vi "NLEISView_v15.vi"() -> ()   [LabVIEW 2018]
doc: "This example shows the Standard Function output mode. \n\nIt also shows some of the parameters which can be changed on the fly."
uses:
  <vilib>/Analysis/baseanly.llb/Mean (DBL).vi
  <vilib>/gmath/NumericalOptimization/Nonlinear Curve Fit TRDL bound.vi
  <vilib>/Analysis/polynomials.llb/Scalar Polynomial Evaluation (DBL).vi
  <vilib>/gmath/NI_Gmath.lvlib
  <vilib>/Analysis/NI_AALPro.lvlib
  <vilib>/Analysis/NI_AALBase.lvlib
panel:
  out "Number of Amps erased":dbl[][](array[numeric]) caption="Mag   Re     Im     Mag   Re     Im    Mag   Re     Im   Mag   Re     Im   Mag   Re     Im\n         V1                 V2                 V3                 V4                V5"
  in  "?":T1(tab)
  in  "Voltage Signal Amplification":string(combo)="1"
  in  "Current Signal Amplification":string(combo)="1"
  in  "Perturbation Method":string(combo)="1"
  in  "IR Setting":enum32{"Single IR", "Multiple IR"}(tab)
  in  "Internal Resistor":string(combo)
  in  "Low Freq (Hz) \nFor IR Switch":dbl
  in  "IR High Freq":string(combo)
  in  "IR Mid Freq":string(combo)
  in  "IR Low Freq":string(combo)
  in  "High Freq  (Hz)\nFor IR Switch":dbl
  in  "Highest Amplitude #":dbl=20.0 format="%#.3f"
  in  "Lowest Amplitude #":dbl=1.0 caption="Amps" format="%#.3f"
  in  "Frequencies High To Low":bool=TRUE
  in  "Highest Freq #":dbl=1.0 format="%#.3f"
  in  "Lowest Freq #":dbl=1.0 caption="Freqs" format="%#.3f"
  in  "Append To File?":bool=TRUE
  in  "Write NLEIS VIEW to File?":bool=TRUE
  in  "Harmonic Nondimensionalization":enum32{"Dimensional", "NonDimensional"}(tab)
  in  "Temperature":dbl=1.0
  out "Vstar":dbl
  in  "Temperature 2":dbl=1.0
  in  "Istar (Amps)":dbl=1.0 format="%.8f"
  in  "Rchem":dbl=1.0
  out "Vstar 2":dbl
  in  "Istar Entered":bool
  in  "Write SUBVI Array?":bool
  in  "File Path Write SUBVI Array":path=path "C:/new3.txt"
  in  "Fitting Parameters":T2(tab)
  in  "LS Program":bool
  in  "Tolerance (vk)":dbl=0.0001
  in  "Fitting Method (vk)":string(combo)="0"
  in  "Gaussian Window\nParameter (B)":dbl=20.0
  in  "Error Noise Filter":dbl=1.5
  in  "Sigma Noise Filter":dbl=1.5
  in  "Lookup Table":bool
  in  "Baseline":bool
  in  "Tolerance (a)":dbl=1e-15
  in  "Max Iterations (a)":i32=1000
  in  "% of V11":dbl=10.0
  in  "% of V22/V33":dbl=50.0
  in  "Fitting Method (a)":string(combo)="0"
  in  "V15 & V35":bool
  in  "V24 Fitting":bool
  in  "V13 Fitting":bool
  in  "Weighting":bool caption="Use\n \n \nDon't Use"
  in  "V1/Alpha Amp to Noise Ratio":dbl=10.0
  in  "V2 Amp to Noise Ratio":dbl=5.0
  in  "V3 Amp to Noise Ratio":dbl=3.0
  in  "V4 Amp to Noise Ratio":dbl=3.0
  in  "V5 Amp to Noise Ratio":dbl=3.0
  out "Graphs Updated":bool
  in  "Alpha Fitting Filters":enum32{"1 Set of Param.", "3 Sets of Param."}(tab)=enum."3 Sets of Param."
  in  "Amps Erase":sgl
  in  "MSE Multiplier":dbl=1.0
  in  "V1 Amps Erase":sgl
  in  "V2 Amps Erase":sgl
  in  "V3 Amps Erase":sgl
  in  "V1 MSE Multiplier":dbl=100.0
  in  "V2 MSE Multiplier":dbl=100.0
  in  "V3 MSE Multiplier":dbl=100.0
  out "Number of Amps used":dbl[](array[numeric])
  in  "stop":bool
  in  "File Path Write NLEISVIEW Data":path=path "C:/Users/Giang/Desktop/NLEIS_test/nleis-test6/diode"
  out "Frequency":dbl=25.298234939575195 format="%#_10f"
  in  "Front Panel Tab Control Icon - Do not delete":enum32{"V vs. Alpha", "Vn vs. Alpha^n"}(tab)=enum."Vn vs. Alpha^n"
  out "V2 Re":cluster{cluster{dbl, "P(a)":dbl}[]}[](graph)
  out "V2 Mag":cluster{cluster{dbl, "P(a)":dbl}[]}[](graph)
  out "V5 Re":T3(graph)
  out "V2 Im":cluster{cluster{dbl, "P(a)":dbl}[]}[](graph)
  out "V3 Mag":cluster{cluster{dbl, "P(a)":dbl}[]}[](graph)
  out "V3 Re":cluster{cluster{dbl, "P(a)":dbl}[]}[](graph)
  out "V3 Im":cluster{cluster{dbl, "P(a)":dbl}[]}[](graph)
  out "V1 Im":cluster{cluster{dbl, "P(a)":dbl}[]}[](graph)
  out "V5 Mag":T3(graph)
  out "V4 Mag":T3(graph)
  out "V4 Re":T3(graph)
  out "V4 Im":cluster{cluster{dbl, "P(a)":dbl}[]}[](graph)
  out "V5 Im":T3(graph)
  out "V1 Mag":cluster{cluster{dbl, dbl}[]}[](graph)=[{[{0.0, 0.0}, {0.11592337776297197, 0.03304485781030145}, {0.17490677190679904, 0.04955962038935185}, {0.3482190445344051, 0.09902951519088735}, {0.5812437888783601, 0.16517748864964857}, {0.8729957405472275, 0.2483952099845861}, {0.9301513780701758, 0.2646275668898653}, {0.9887433954568534, 0.2813401317697576}, {1.0477077074181451, 0.29781838994307164}, {1.1050180353393082, 0.314210624473721}, {1.3370638463516271, 0.38017329335049976}, {1.3957495994333853, 0.39653508030752266}, {1.5127853787825267, 0.429714440189949}, {1.5708225495208372, 0.4461228771616594}]}, {[{0.0, 0.0}, {0.11592337776297197, 0.03295810708345434}, {0.17490677190679904, 0.04972841122082627}, {0.3482190445344051, 0.0990110384083542}, {0.5812437888783601, 0.16529212065005314}, {0.8729957405472275, 0.24829143514258742}, {0.9301513780701758, 0.2645473352700113}, {0.9887433954568534, 0.2812079100684176}, {1.0477077074181451, 0.2979689236770735}, {1.1050180353393082, 0.31425292299017493}, {1.3370638463516271, 0.3800753565931724}, {1.3957495994333853, 0.39668139114349815}, {1.5127853787825267, 0.4297271370666853}, {1.5708225495208372, 0.44607154435403673}]}]
  out "V1 Re":cluster{cluster{dbl, "P(a)":dbl}[]}[](graph)
  out "V4 Im vs. a^4":cluster{cluster{dbl, "P(a)":dbl}[]}[](graph)
  out "V5 Im vs. a^5":cluster{cluster{dbl, "P(a)":dbl}[]}[](graph)
  out "V3 Mag vs. a^3":cluster{cluster{dbl, "P(a)":dbl}[]}[](graph)
  out "V4 Mag vs. a^4":cluster{cluster{dbl, "P(a)":dbl}[]}[](graph)
  out "V5 Mag vs. a^5":cluster{cluster{dbl, "P(a)":dbl}[]}[](graph)
  out "V2 Im vs. a^2":cluster{cluster{dbl, "P(a)":dbl}[]}[](graph)
  out "V2 Re vs. a^2":cluster{cluster{dbl, "P(a)":dbl}[]}[](graph)
  out "V2 Mag vs. a^2":cluster{cluster{dbl, "P(a)":dbl}[]}[](graph)
  out "V3 Im vs. a^3":cluster{cluster{dbl, "P(a)":dbl}[]}[](graph)
  out "V5 Re vs. a^5":cluster{cluster{dbl, "P(a)":dbl}[]}[](graph)
  out "V4 Re vs. a^4":cluster{cluster{dbl, "P(a)":dbl}[]}[](graph)
  out "V3 Re vs. a^3":cluster{cluster{dbl, "P(a)":dbl}[]}[](graph)
  out "V1 Im vs. a^1":cluster{cluster{dbl, "P(a)":dbl}[]}[](graph)
  out "V1 Mag vs. a^1":cluster{cluster{dbl, dbl}[]}[](graph)=[{[{0.0, 0.0}, {0.11592337776297197, 0.03304485781030145}, {0.17490677190679904, 0.04955962038935185}, {0.3482190445344051, 0.09902951519088735}, {0.5812437888783601, 0.16517748864964857}, {0.8729957405472275, 0.2483952099845861}, {0.9301513780701758, 0.2646275668898653}, {0.9887433954568534, 0.2813401317697576}, {1.0477077074181451, 0.29781838994307164}, {1.1050180353393082, 0.314210624473721}, {1.3370638463516271, 0.38017329335049976}, {1.3957495994333853, 0.39653508030752266}, {1.5127853787825267, 0.429714440189949}, {1.5708225495208372, 0.4461228771616594}]}, {[{0.0, 0.0}, {0.11592337776297197, 0.03295810708345434}, {0.17490677190679904, 0.04972841122082627}, {0.3482190445344051, 0.0990110384083542}, {0.5812437888783601, 0.16529212065005314}, {0.8729957405472275, 0.24829143514258742}, {0.9301513780701758, 0.2645473352700113}, {0.9887433954568534, 0.2812079100684176}, {1.0477077074181451, 0.2979689236770735}, {1.1050180353393082, 0.31425292299017493}, {1.3370638463516271, 0.3800753565931724}, {1.3957495994333853, 0.39668139114349815}, {1.5127853787825267, 0.4297271370666853}, {1.5708225495208372, 0.44607154435403673}]}]
  out "V1 Re vs. a^1":cluster{cluster{dbl, "P(a)":dbl}[]}[](graph)
  in  "File Path Read NLEISRUN Data":path=path "C:/Users/Giang/Desktop/NLEIS_test/test6/diode"
  # "MSE Multiplier\n \nAmps Erase\n \nSigma/MSE Noise Filters"
  # "Amplitudes"
  # "Frequencies"
  # "Higher Harmonic\nBounds"
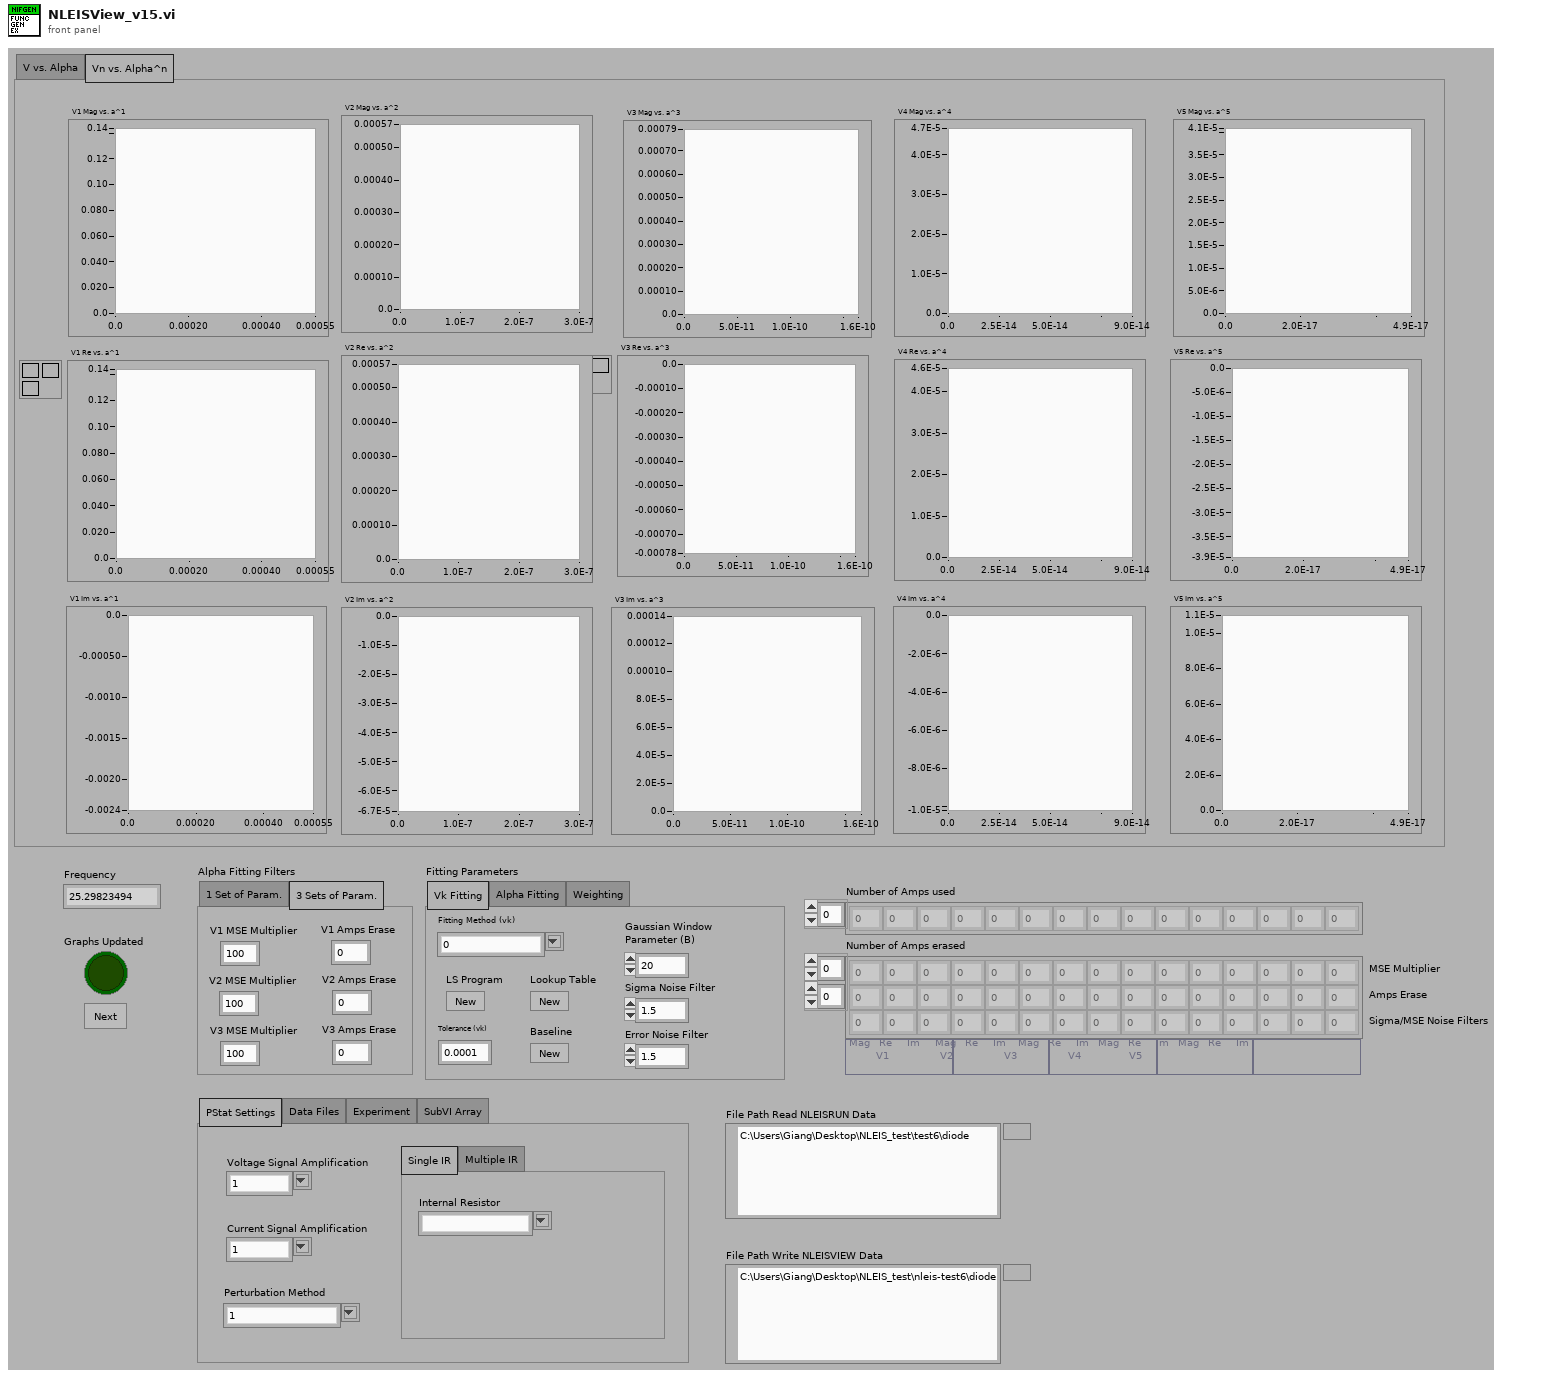
[diagram p1: front panel]
types:
  T1 = enum32{"PStat Settings", "Data Files", "Experiment", "SubVI Array"}
  T2 = enum32{"Vk Fitting", "Alpha Fitting", "Weighting"}
  T3 = cluster{cluster{"new element/subarray":dbl, "P(a)":dbl}[]}[]
  T4 = cluster{"Max Iterations (a)":i32, "Tolerance (a)":dbl}
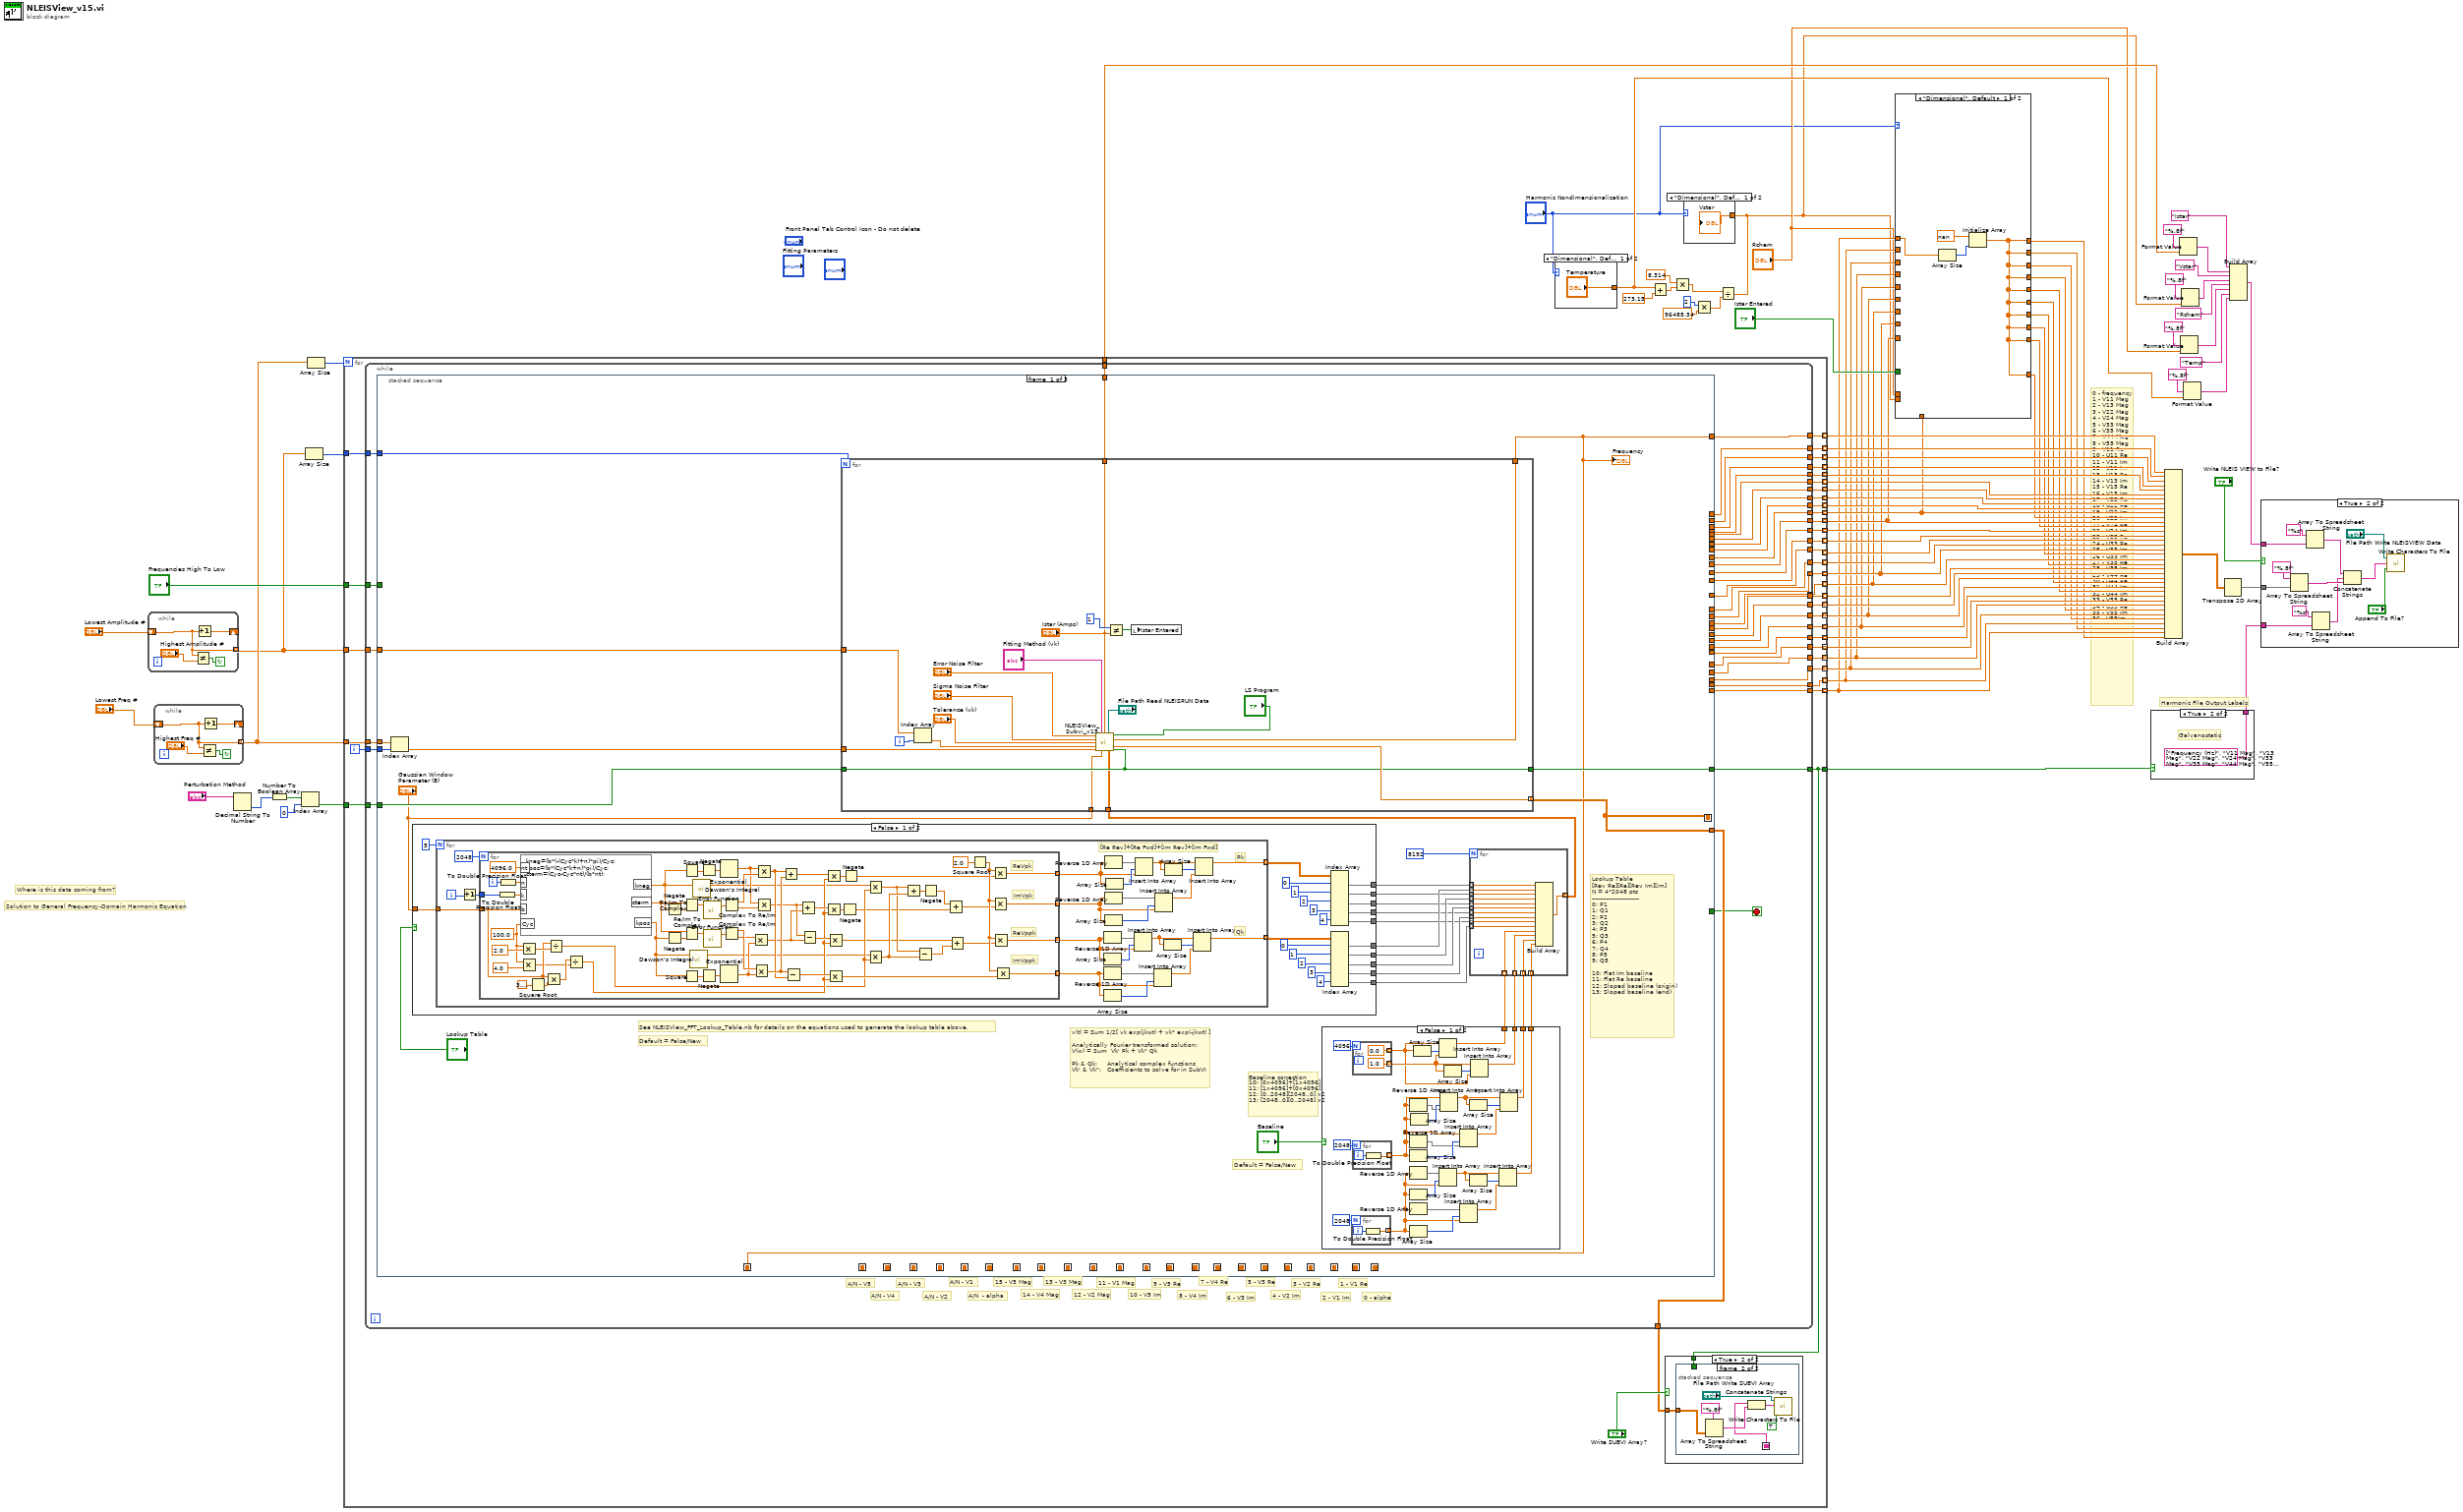
[diagram p0: block diagram]
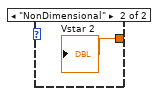
[diagram p2: hidden frame]
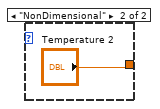
[diagram p3: hidden frame]
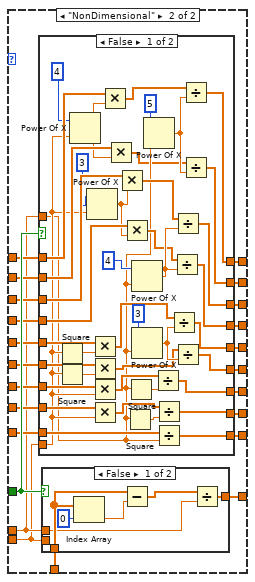
[diagram p4: hidden frame]
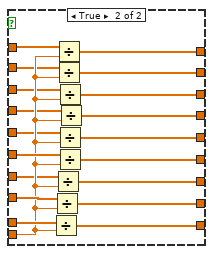
[diagram p5: hidden frame]
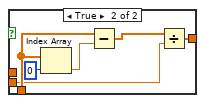
[diagram p6: hidden frame]
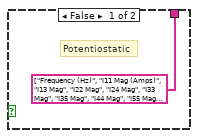
[diagram p8: hidden frame]
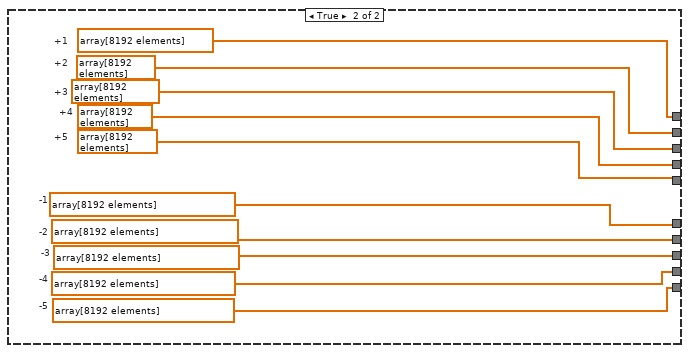
[diagram p9: hidden frame]
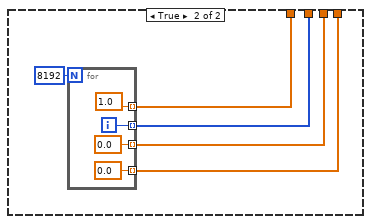
[diagram p10: hidden frame]
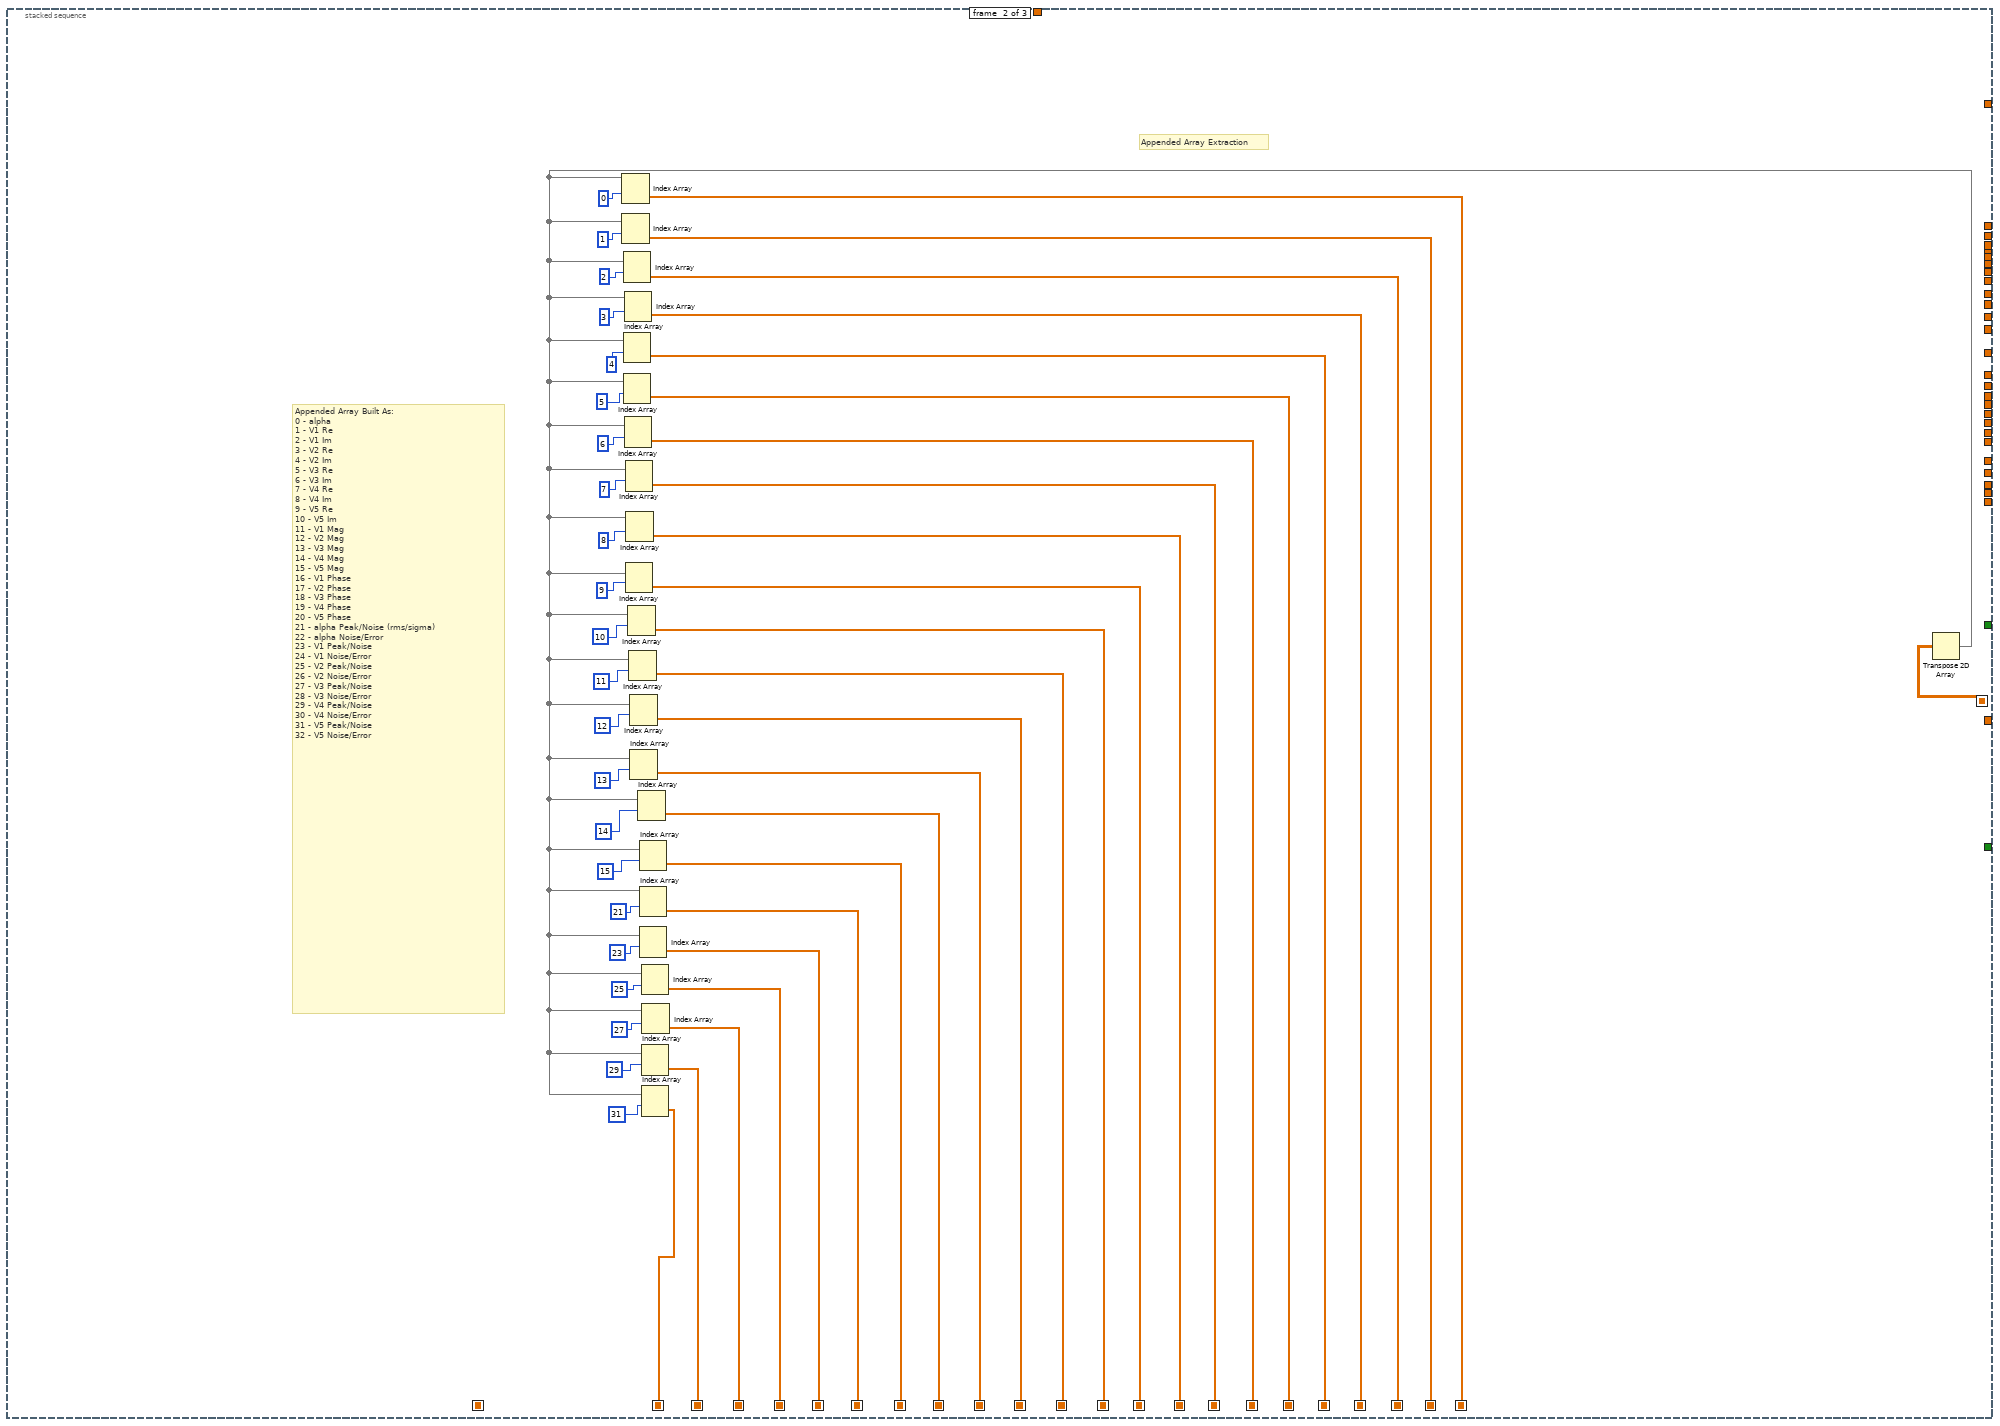
[diagram p11: hidden frame]
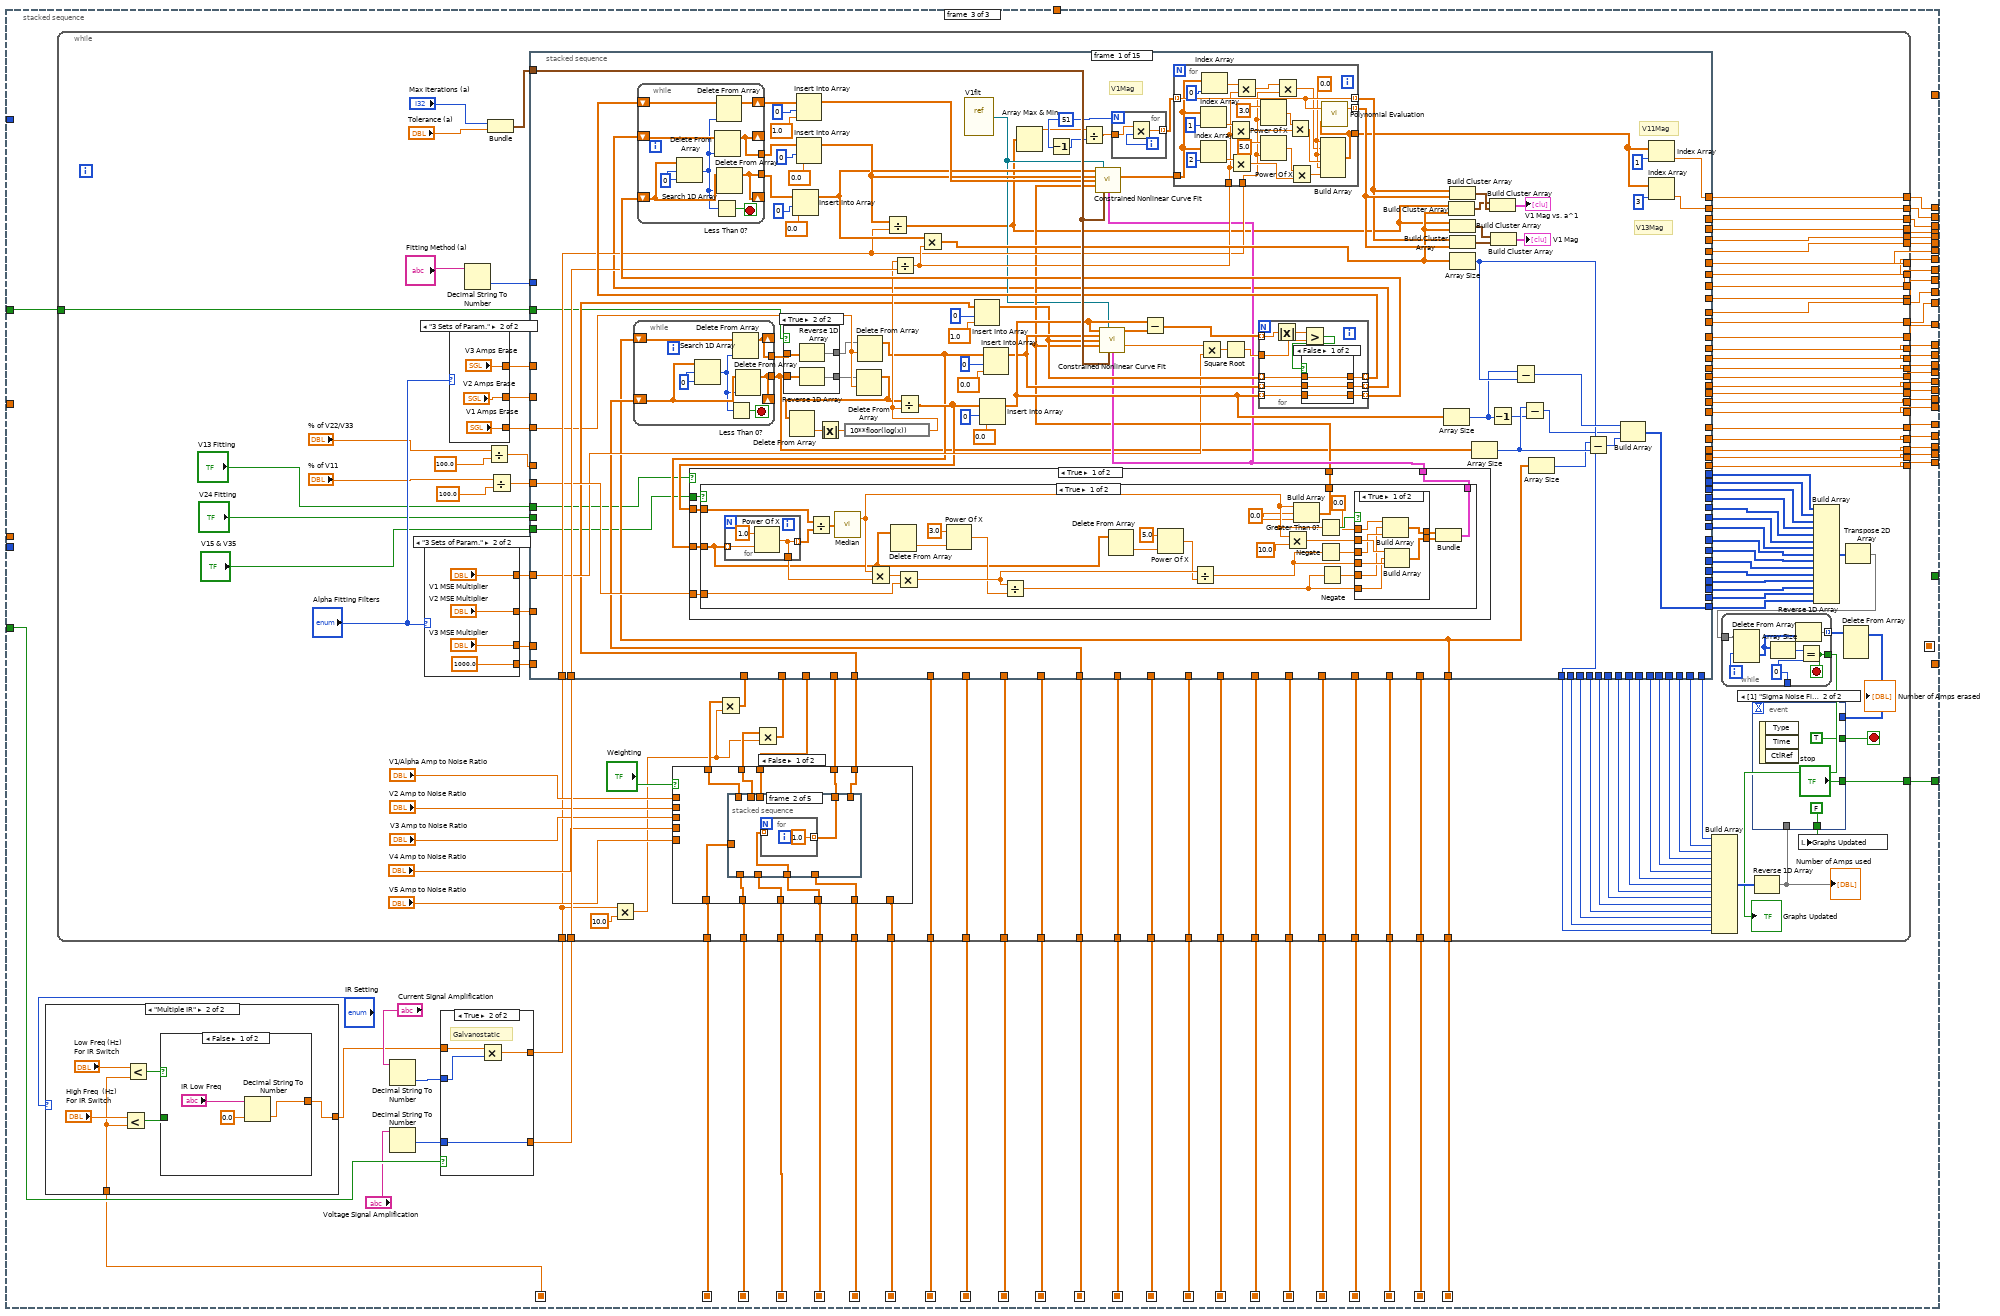
[diagram p12: hidden frame]
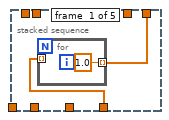
[diagram p13: hidden frame]
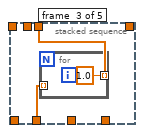
[diagram p14: hidden frame]
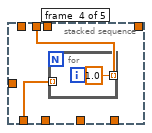
[diagram p15: hidden frame]
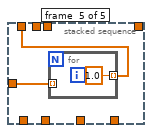
[diagram p16: hidden frame]
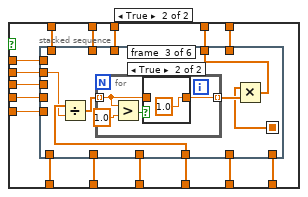
[diagram p17: hidden frame]
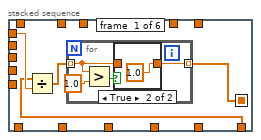
[diagram p18: hidden frame]
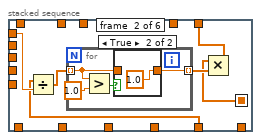
[diagram p20: hidden frame]
diagram:
  # "Where is this data coming from?"
  # "Solution to General Frequency-Domain Harmonic Equation"
  # "0 - frequency\n1 - V11 Mag\n2 - V13 Mag\n3 - V22 Mag\n4 - V24 Mag\n5 - V33 Mag\n6 - V35 Mag\n7 - V44 Mag\n8 - V55 Mag\n9 - V11 Re\n10 - U11 Re\n11 - V11 Im\n12 - U11 Im\n13 - V13 Re\n14 - V13 Im\n15 - V15 Re\n16 - V15 Im\n17 - V22 Re\n18 - U22 Re\n19 - V22 Im\n20 - U22 Im\n21 - V24 Re\n22 - V24 Im\n23 - V33 Re\n24 - U33 Re\n25 - V33 Im\n26 - U33 Im\n27 - V35 Re\n28 - V35 Im\n29 - V44 Re\n30 - U44 Re\n31 - V44 Im\n32 - U44 Im\n33 - V55 Re\n34 - U55 Re\n35 - V55 Im\n36 - U55Im"
  # "Harmonic File Output Labels"
  n1 = while {
    shift-right: [w82] -> _
    shift-left: "Lowest Amplitude #" -> [w83]
    tunnel: [w83] -> w29 mode=indexing
    stop <- w84 continue-if-true
    n2 = Not Equal?(x=w83, y="Highest Amplitude #") -> (x != y?=w84:bool)
    n3 = Increment(x=w83) -> (x+1=w82:dbl)
  }
  n4 = while {
    shift-right: [w86] -> _
    shift-left: "Lowest Freq #" -> [w87]
    tunnel: [w87] -> w30 mode=indexing
    stop <- w88 continue-if-true
    n5 = Not Equal?(x=w87, y="Highest Freq #") -> (x != y?=w88:bool)
    n6 = Increment(x=w87) -> (x+1=w86:dbl)
  }
  n7 = Decimal String To Number(string="Perturbation Method") -> (number=w78:i32)  [unwired: 2 in, 1 out]
  n8 = Number To Boolean Array(number=w78) -> (Boolean array=w80:bool[])
  n9 = Index Array(array=w80, index=0) -> (element=w76:bool)
  n10 = Array Size(array=w29) -> (size(s)=w28:i32)
  n11 = Array Size(array=w30) -> (size(s)=w31:i32)
  n12 = for {
    N: w31 -> [_]
    tunnel: [w124] -> w72 mode=indexing
    tunnel: [w123] -> w71 mode=indexing
    tunnel: [w122] -> w70 mode=indexing
    tunnel: [w121] -> w69 mode=indexing
    tunnel: [w120] -> w68 mode=indexing
    tunnel: [w119] -> w67 mode=indexing
    tunnel: [w118] -> w66 mode=indexing
    tunnel: [w117] -> w65 mode=indexing
    tunnel: [w89] -> w51 mode=indexing
    tunnel: [w116] -> w49 mode=indexing
    tunnel: [w115] -> w64 mode=indexing
    tunnel: [w114] -> w63 mode=indexing
    tunnel: [w113] -> w48 mode=indexing
    tunnel: [w112] -> w47 mode=indexing
    tunnel: [w111] -> w61 mode=indexing
    tunnel: [w110] -> w52 mode=indexing
    tunnel: [w109] -> w46 mode=indexing
    tunnel: [w108] -> w45 mode=indexing
    tunnel: [w107] -> w60 mode=indexing
    tunnel: [w106] -> w59 mode=indexing
    tunnel: [w105] -> w44 mode=indexing
    tunnel: [w104] -> w43 mode=indexing
    tunnel: [w103] -> w42 mode=indexing
    tunnel: [w102] -> w41 mode=indexing
    tunnel: [w101] -> w55 mode=indexing
    tunnel: w30 -> [w100]
    tunnel: w76 -> [w99]
    tunnel: w29 -> [w98]
    tunnel: [w90] -> w75
    tunnel: [w97] -> w62 mode=indexing
    tunnel: [w96] -> w53 mode=indexing
    tunnel: "Frequencies High To Low" -> [w95]
    tunnel: w28 -> [w94]
    tunnel: [w93] -> w18
    i -> [w125]
    n13 = while {
      tunnel: w125 -> [w162]
      tunnel: [w161] -> w124
      tunnel: [w160] -> w123
      tunnel: [w159] -> w122
      tunnel: [w158] -> w121
      tunnel: [w157] -> w120
      tunnel: [w156] -> w119
      tunnel: [w155] -> w118
      tunnel: [w154] -> w117
      tunnel: [w153] -> w116
      tunnel: [w152] -> w115
      tunnel: [w151] -> w114
      tunnel: [w150] -> w113
      tunnel: [w149] -> w112
      tunnel: [w148] -> w111
      tunnel: [w147] -> w110
      tunnel: [w146] -> w109
      tunnel: [w145] -> w108
      tunnel: [w144] -> w107
      tunnel: [w143] -> w106
      tunnel: [w142] -> w105
      tunnel: [w141] -> w104
      tunnel: [w140] -> w103
      tunnel: [w139] -> w102
      tunnel: [w138] -> w101
      tunnel: w100 -> [w137]
      tunnel: w99 -> [w136]
      tunnel: w98 -> [w135]
      tunnel: [w134] -> w97
      tunnel: [w133] -> w96
      tunnel: w95 -> [w132]
      tunnel: w94 -> [w131]
      tunnel: [w130] -> w93
      tunnel: [w129] -> w91
      tunnel: [w128] -> w90
      tunnel: [w127] -> w89
      stop <- w126 stop-if-true
      # "A/N - V5"
      # "A/N - V4"
      # "A/N - V3"
      # "A/N - V2"
      # "A/N - V1"
      # "A/N  - alpha"
      # "15 - V5 Mag"
      # "14 - V4 Mag"
      # "13 - V3 Mag"
      # "12 - V2 Mag"
      # "11 - V1 Mag"
      # "10 - V5 Im"
      # "9 - V5 Re"
      # "8 - V4 Im"
      # "7 - V4 Re"
      # "6 - V3 Im"
      # "5 - V3 Re"
      # "4 - V2 Im"
      # "3 - V2 Re"
      # "2 - V1 Im"
      # "1 - V1 Re"
      # "0 - alpha"
      n14 = stacked-sequence {
        seq-local: [w189 _ _] -> [_ w434 _]
        seq-local: [_ w404 _] -> [_ _ w472]
        seq-local: [_ w402 _] -> [_ _ w471]
        seq-local: [_ w401 _] -> [_ _ w470]
        seq-local: [_ w399 _] -> [_ _ w469]
        seq-local: [_ w398 _] -> [_ _ w468]
        seq-local: [_ w396 _] -> [_ _ w467]
        seq-local: [_ w395 _] -> [_ _ w466]
        seq-local: [_ w417 _] -> [_ _ w465]
        seq-local: [_ w416 _] -> [_ _ w464]
        seq-local: [_ w415 _] -> [_ _ w463]
        seq-local: [_ w414 _] -> [_ _ w462]
        seq-local: [_ w403 _] -> [_ _ w461]
        seq-local: [_ w400 _] -> [_ _ w460]
        seq-local: [_ w397 _] -> [_ _ w459]
        seq-local: [_ w413 _] -> [_ _ w458]
        seq-local: [_ w412 _] -> [_ _ w457]
        seq-local: [w182 _ _] -> [_ _ w444]
        seq-local: [_ w394 _] -> [_ _ w441]
        seq-local: [_ w393 _] -> [_ _ w440]
        seq-local: [_ w392 _] -> [_ _ w439]
        seq-local: [_ w391 _] -> [_ _ w438]
        seq-local: [_ w390 _] -> [_ _ w437]
        seq-local: [_ w389 _] -> [_ _ w436]
        tunnel: w162 -> [w191 _ _]
        tunnel: [_ _ w494] -> w127
        tunnel: [_ _ w493] -> w153
        tunnel: [_ _ w492] -> w152
        tunnel: [_ _ w491] -> w151
        tunnel: [_ _ w490] -> w134
        tunnel: [_ _ w489] -> w133
        tunnel: [_ _ w456] -> w150
        tunnel: [_ _ w488] -> w149
        tunnel: [_ _ w455] -> w148
        tunnel: [_ _ w487] -> w147
        tunnel: [_ _ w452] -> w146
        tunnel: [_ _ w450] -> w145
        tunnel: [_ _ w451] -> w144
        tunnel: [_ _ w449] -> w143
        tunnel: [_ _ w486] -> w142
        tunnel: [_ _ w485] -> w141
        tunnel: [_ _ w484] -> w140
        tunnel: [_ _ w483] -> w139
        tunnel: [_ _ w482] -> w160
        tunnel: [w182 _ _] -> w161
        tunnel: [_ _ w481] -> w159
        tunnel: [_ _ w480] -> w158
        tunnel: [_ _ w479] -> w157
        tunnel: [_ _ w454] -> w156
        tunnel: [_ _ w453] -> w155
        tunnel: [_ _ w448] -> w154
        tunnel: [_ _ w447] -> w138
        tunnel: w137 -> [w190 _ _]
        tunnel: [w189 _ _] -> w129
        tunnel: w136 -> [w188 _ w478]
        tunnel: w135 -> [w187 _ _]
        tunnel: [w186 _ _] -> w128
        tunnel: w132 -> [_ _ w446]
        tunnel: w131 -> [w185 _ _]
        tunnel: [w184 _ _] -> w130
        tunnel: [_ _ w435] -> w126
        frame #0 {
          # "Baseline correction\n10: [0x4096]+[1x4096]\n11: [1x4096]+[0x4096]\n12: [0..2048][2048..0] x2\n13: [2048..0][0..2048] x2"
          # "v(t) = Sum 1/2[ vk exp(jkwt) + vk* exp(-jkwt) ]\n\nAnalytically Fourier transformed solution:\nV(w) = Sum  Vk' Pk + Vk\" Qk\n\nPk & Qk:     Analytical complex functions\nVk' & Vk\":   Coefficients to solve for in SubVI"
          # "Lookup Table\n[Rev Re][Re][Rev Im][Im]\nN = 4*2048 pts\n------------------------\n0: P1\n1: Q1\n2: P2\n3: Q2\n4: P3\n5: Q3\n6: P4\n7: Q4\n8: P5\n9: Q5\n\n10: Flat Im baseline\n11: Flat Re baseline\n12: Sloped baseline (origin)\n13: Sloped baseline (end)"
          # "Default = False/New"
          # "Default = False/New"
          # "See NLEISView_FFT_Lookup_Table.nb for details on the equations used to generate the lookup table above."
          n15 = Index Array(array=w190, index=w191) -> (element=w183:dbl)
          n16 = case shown="False" "Lookup Table" {
            tunnel: [w213 w313] -> w180
            tunnel: [w212 w308] -> w179
            tunnel: [w211 w312] -> w178
            tunnel: [w210 w307] -> w177
            tunnel: [w209 w311] -> w176
            tunnel: [w208 w306] -> w175
            tunnel: [w207 w310] -> w174
            tunnel: [w206 w305] -> w173
            tunnel: [w205 w309] -> w172
            tunnel: [w204 w304] -> w171
            tunnel: "Gaussian Window\nParameter (B)" -> [w203 _]
            frame False {
              n17 = for {
                N: 5 -> [_]
                tunnel: w203 -> [w238]
                tunnel: [w219] -> w215 mode=indexing
                tunnel: [w218] -> w214 mode=indexing
                i -> [w237]
                # "[Re Rev]+[Re Fwd]+[Im Rev]+[Im Fwd]"
                # "Qk"
                # "Pk"
                n18 = Increment(x=w237) -> (x+1=w236:i32)
                n19 = for {
                  N: 2048 -> [_]
                  tunnel: w238 -> [w275]
                  tunnel: w236 -> [w300]
                  tunnel: [w293] -> w229 mode=indexing
                  tunnel: [w294] -> w228 mode=indexing
                  tunnel: [w295] -> w221 mode=indexing
                  tunnel: [w296] -> w220 mode=indexing
                  i -> [w303]
                  w278 = 100.0 ("element")
                  # "ImVppk"
                  # "ReVppk"
                  # "ImVpk"
                  # "ReVpk"
                  n20 = To Double Precision Float(number=w300) -> (double precision float=w299:dbl)
                  n21 = To Double Precision Float(number=w303) -> (double precision float=w301:dbl)
                  n22 = Multiply(x=w278, y=2.0 ("element")) -> (x*y=w279:dbl)
                  n23 = Multiply(x=w278, y=4.0 ("element")) -> (x*y=w272:dbl)
                  n24 = formula code="kneg=(b*(-(Cyc*k)+n)*pi)/Cyc;\nkpos=(b*(Cyc*k+n)*pi)/Cyc;\ncterm=(Cyc-Cyc*nt)/(b*nt);"("n"=w301, "Cyc"=w278, "b"=w275, "k"=w299, "nt"=4096.0 ("element")) -> ("kpos"=w264:dbl, "kneg"=w263:dbl, "cterm"=w285:dbl)
                  n25 = Square Root(x=3.141592653589793) -> (sqrt(x)=w274:dbl)
                  n26 = Multiply(x=w275, y=w274) -> (x*y=w273:dbl)
                  n27 = Divide(x=w275, y=w279) -> (x/y=w251:dbl)
                  n28 = Divide(x=w273, y=w272) -> (x/y=w256:dbl)
                  n29 = Negate(x=w263) -> (-x=w291:dbl)
                  n30 = Negate(x=w264) -> (-x=w284:dbl)
                  n31 = Square(x=w263) -> (x^2=w289:dbl)
                  n32 = Re/Im To Complex(1:w291, 2:w285) -> (0:w290:cdb)
                  n33 = Re/Im To Complex(1:w284, 2:w285) -> (0:w283:cdb)
                  n34 = Square(x=w264) -> (x^2=w282:dbl)
                  n35 = call <vilib>:"Dawson's Integral.vi"("x"=w264) -> ("daw(x)"=w250:dbl)  [unwired: 2 in]
                  n36 = call <vilib>:"Dawson's Integral.vi"("x"=w263) -> ("daw(x)"=w252:dbl)  [unwired: 2 in]
                  n37 = Negate(x=w289) -> (-x=w288:dbl)
                  n38 = Negate(x=w282) -> (-x=w281:dbl)
                  n39 = call <vilib>:"Error Function.vi"("x"=w290) -> ("erf(x)"=w292:dbl)  [unwired: 2 in]
                  n40 = call <vilib>:"Error Function.vi"("x"=w283) -> ("erf(x)"=w286:dbl)  [unwired: 2 in]
                  n41 = Exponential(1:w288) -> (0:w260:dbl)
                  n42 = Exponential(1:w281) -> (0:w257:dbl)
                  n43 = Complex To Re/Im(x + iy=w292) -> (x=w287:dbl, y=w261:dbl)
                  n44 = Complex To Re/Im(x + iy=w286) -> (x=w280:dbl, y=w258:dbl)
                  n45 = Multiply(x=w258, y=w257) -> (x*y=w253:dbl)
                  n46 = Multiply(x=w280, y=w257) -> (x*y=w267:dbl)
                  n47 = Multiply(x=w260, y=w287) -> (x*y=w266:dbl)
                  n48 = Multiply(x=w260, y=w261) -> (x*y=w254:dbl)
                  n49 = Add(x=w266, y=w267) -> (x+y=w271:dbl)
                  n50 = Subtract(x=w267, y=w266) -> (x-y=w268:dbl)
                  n51 = Add(x=w254, y=w253) -> (x+y=w262:dbl)
                  n52 = Subtract(x=w254, y=w253) -> (x-y=w259:dbl)
                  n53 = Multiply(x=w271, y=w256) -> (x*y=w270:dbl)
                  n54 = Multiply(x=w262, y=w256) -> (x*y=w255:dbl)
                  n55 = Multiply(x=w259, y=w256) -> (x*y=w243:dbl)
                  n56 = Multiply(x=w268, y=w256) -> (x*y=w265:dbl)
                  n57 = Negate(x=w255) -> (-x=w246:dbl)
                  n58 = Negate(x=w270) -> (-x=w269:dbl)
                  n59 = Multiply(x=w252, y=w251) -> (x*y=w248:dbl)
                  n60 = Multiply(x=w250, y=w251) -> (x*y=w249:dbl)
                  n61 = Add(x=w248, y=w249) -> (x+y=w247:dbl)
                  n62 = Subtract(x=w248, y=w249) -> (x-y=w244:dbl)
                  n63 = Negate(x=w247) -> (-x=w245:dbl)
                  n64 = Add(x=w245, y=w246) -> (x+y=w242:dbl)
                  n65 = Add(x=w243, y=w244) -> (x+y=w241:dbl)
                  n66 = Square Root(x=2.0 ("element")) -> (sqrt(x)=w297:dbl)
                  n67 = Multiply(x=w297, y=w269) -> (x*y=w293:dbl)
                  n68 = Multiply(x=w297, y=w242) -> (x*y=w294:dbl)
                  n69 = Multiply(x=w297, y=w241) -> (x*y=w295:dbl)
                  n70 = Multiply(x=w297, y=w265) -> (x*y=w296:dbl)
                }
                n71 = Reverse 1D Array(array=w221) -> (reversed array=w222:dbl[])
                n72 = Reverse 1D Array(array=w220) -> (reversed array=w216:dbl[])
                n73 = Array Size(array=w220) -> (size(s)=w223:i32)
                n74 = Array Size(array=w221) -> (size(s)=w224:i32)
                n75 = Reverse 1D Array(array=w229) -> (reversed array=w230:dbl[])
                n76 = Reverse 1D Array(array=w228) -> (reversed array=w217:dbl[])
                n77 = Array Size(array=w228) -> (size(s)=w231:i32)
                n78 = Array Size(array=w229) -> (size(s)=w232:i32)
                n79 = Insert Into Array(array=w222, index=w224, new element=w221) -> (w227:dbl[])
                n80 = Insert Into Array(array=w230, index=w232, new element=w229) -> (w235:dbl[])
                n81 = Insert Into Array(array=w216, index=w223, new element=w220) -> (w226:dbl[])
                n82 = Insert Into Array(array=w217, index=w231, new element=w228) -> (w234:dbl[])
                n83 = Array Size(array=w227) -> (size(s)=w225:i32)
                n84 = Array Size(array=w235) -> (size(s)=w233:i32)
                n85 = Insert Into Array(array=w227, index=w225, new element=w226) -> (w218:dbl[])
                n86 = Insert Into Array(array=w235, index=w233, new element=w234) -> (w219:dbl[])
              }
              n87 = Index Array(array=w215, index (row) #1=0, index (row) #2=1, index (row) #3=2, index (row) #4=3, index (row) #5=4) -> (element #1=w213:dbl[], element #2=w211:dbl[], element #3=w209:dbl[], element #4=w207:dbl[], element #5=w205:dbl[])  [unwired: 5 in]
              n88 = Index Array(array=w214, index (row) #1=0, index (row) #2=1, index (row) #3=2, index (row) #4=3, index (row) #5=4) -> (element #1=w212:dbl[], element #2=w210:dbl[], element #3=w208:dbl[], element #4=w206:dbl[], element #5=w204:dbl[])  [unwired: 5 in]
            }
            frame True {
              w304 = dbl[] array[8192 elements]  # -5
              w309 = dbl[] array[8192 elements]  # +5
              w305 = dbl[] array[8192 elements]  # -4
              w310 = dbl[] array[8192 elements]  # +4
              w306 = dbl[] array[8192 elements]  # -3
              w311 = dbl[] array[8192 elements]  # +3
              w307 = dbl[] array[8192 elements]  # -2
              w312 = dbl[] array[8192 elements]  # +2
              w308 = dbl[] array[8192 elements]  # -1
              w313 = dbl[] array[8192 elements]  # +1
            }
          }
          n89 = case shown="False" "Baseline" {
            tunnel: [w332 w347] -> w170
            tunnel: [w322 w348] -> w169
            tunnel: [w317 w350] -> w168
            tunnel: [w316 w349] -> w167
            frame False {
              n90 = for {
                N: 2048 -> [_]
                tunnel: [w345] -> w333 mode=indexing
                i -> [w346]
                n91 = To Double Precision Float(number=w346) -> (double precision float=w345:dbl)
              }
              n92 = for {
                N: 4096 -> [_]
                tunnel: [0.0 ("element")] -> w318 mode=indexing
                tunnel: [1.0 ("element")] -> w319 mode=indexing
              }
              n93 = for {
                N: 2048 -> [_]
                tunnel: [w341] -> w315 mode=indexing
                i -> [w342]
                n94 = To Double Precision Float(number=w342) -> (double precision float=w341:dbl)
              }
              n95 = Reverse 1D Array(array=w333) -> (reversed array=w335:dbl[])
              n96 = Reverse 1D Array(array=w333) -> (reversed array=w314:dbl[])
              n97 = Array Size(array=w333) -> (size(s)=w336:i32)
              n98 = Reverse 1D Array(array=w315) -> (reversed array=w324:dbl[])
              n99 = Reverse 1D Array(array=w315) -> (reversed array=w323:dbl[])
              n100 = Array Size(array=w315) -> (size(s)=w326:i32)
              n101 = Array Size(array=w333) -> (size(s)=w337:i32)
              n102 = Array Size(array=w315) -> (size(s)=w327:i32)
              n103 = Array Size(array=w318) -> (size(s)=w321:i32)
              n104 = Insert Into Array(array=w318, index=w321, new element=w319) -> (w317:dbl[])
              n105 = Insert Into Array(array=w335, index=w337, new element=w333) -> (w340:dbl[])
              n106 = Insert Into Array(array=w315, index=w327, new element=w324) -> (w330:dbl[])
              n107 = Array Size(array=w319) -> (size(s)=w320:i32)
              n108 = Insert Into Array(array=w314, index=w336, new element=w333) -> (w339:dbl[])
              n109 = Insert Into Array(array=w315, index=w326, new element=w323) -> (w329:dbl[])
              n110 = Array Size(array=w340) -> (size(s)=w338:i32)
              n111 = Array Size(array=w330) -> (size(s)=w328:i32)
              n112 = Insert Into Array(array=w319, index=w320, new element=w318) -> (w316:dbl[])
              n113 = Insert Into Array(array=w340, index=w338, new element=w339) -> (w332:dbl[])
              n114 = Insert Into Array(array=w330, index=w328, new element=w329) -> (w322:dbl[])
            }
            frame True {
              n115 = for {
                N: 8192 -> [_]
                tunnel: [1.0 ("element")] -> w350 mode=indexing
                tunnel: [w354] -> w349 mode=indexing
                tunnel: [0.0 ("element")] -> w348 mode=indexing
                tunnel: [0.0 ("element")] -> w347 mode=indexing
                i -> [w354]
              }
            }
          }
          n116 = for {
            N: 8192 -> [_]
            tunnel: [w370] -> w166 mode=indexing
            tunnel: w180 -> [w369] mode=indexing
            tunnel: w179 -> [w368] mode=indexing
            tunnel: w178 -> [w367] mode=indexing
            tunnel: w177 -> [w366] mode=indexing
            tunnel: w176 -> [w365] mode=indexing
            tunnel: w175 -> [w364] mode=indexing
            tunnel: w174 -> [w363] mode=indexing
            tunnel: w173 -> [w362] mode=indexing
            tunnel: w172 -> [w361] mode=indexing
            tunnel: w171 -> [w360] mode=indexing
            tunnel: w170 -> [w359] mode=indexing
            tunnel: w169 -> [w358] mode=indexing
            tunnel: w168 -> [w357] mode=indexing
            tunnel: w167 -> [w356] mode=indexing
            n117 = Build Array(w369, w368, w367, w366, w365, w364, w363, w362, w361, w360, w357, w356, w358, w359) -> (w370:dbl[])
          }
          n118 = for {
            N: w185 -> [_]
            tunnel: w183 -> [w380]
            tunnel: [w388] -> w189 mode=indexing
            tunnel: w188 -> [w385]
            tunnel: w187 -> [w387]
            tunnel: [w385] -> w186
            tunnel: [w384] -> w182
            tunnel: ["Istar (Amps)"] -> w184
            tunnel: w166 -> [w375]
            tunnel: "Gaussian Window\nParameter (B)" -> [w376]
            i -> [w386]
            n119 = Index Array(array=w387, index=w386) -> (element=w379:dbl)
            n120 = call "NLEISView_Subvi_v15.vi"("Ratio Multiplier"="Error Noise Filter", "Vk Fitting Algorithm"="Fitting Method (vk)", "Char Current (Amps)"="Istar (Amps)", "file path (dialog if empty)"="File Path Read NLEISRUN Data", "LS Program"="LS Program", "Sigma Multiplier"="Sigma Noise Filter", "Vk Fitting Tolerance"="Tolerance (vk)", "Amplitude Run Number"=w379, "Frequency Run Number"=w380, "Gaussian Window\nParameter (B)"=w376, "Lookup Table"=w375, "Perturbation Method"=w385) -> ("Frequency"=w384:sgl, "Fit Coefficients and Noise Ratios"=w388:dbl[])  [unwired: 2 in]
            n121 = Not Equal?(x=1, y="Istar (Amps)") -> (x != y?=w382:bool)
            n122 = local write "Istar Entered"(w382) -> ()
          }
          "Frequency" <- w182
        }
        frame #1 {
          # "Appended Array Built As:\n0 - alpha\n1 - V1 Re\n2 - V1 Im\n3 - V2 Re\n4 - V2 Im\n5 - V3 Re\n6 - V3 Im\n7 - V4 Re\n8 - V4 Im\n9 - V5 Re\n10 - V5 Im\n11 - V1 Mag\n12 - V2 Mag\n13 - V3 Mag\n14 - V4 Mag\n15 - V5 Mag\n16 - V1 Phase\n17 - V2 Phase\n18 - V3 Phase\n19 - V4 Phase\n20 - V5 Phase\n21 - alpha Peak/Noise (rms/sigma)\n22 - alpha Noise/Error\n23 - V1 Peak/Noise\n24 - V1 Noise/Error\n25 - V2 Peak/Noise\n26 - V2 Noise/Error\n27 - V3 Peak/Noise\n28 - V3 Noise/Error\n29 - V4 Peak/Noise\n30 - V4 Noise/Error\n31 - V5 Peak/Noise\n32 - V5 Noise/Error"
          # "Appended Array Extraction"
          n123 = Transpose 2D Array(2D array=w434) -> (transposed array=w405:dbl[][])
          n124 = Index Array(array=w405, index (row)=0) -> (element=w404:dbl[])  [unwired: 1 in]
          n125 = Index Array(array=w405, index (row)=1) -> (element=w402:dbl[])  [unwired: 1 in]
          n126 = Index Array(array=w405, index (row)=2) -> (element=w401:dbl[])  [unwired: 1 in]
          n127 = Index Array(array=w405, index (row)=4) -> (element=w398:dbl[])  [unwired: 1 in]
          n128 = Index Array(array=w405, index (row)=5) -> (element=w396:dbl[])  [unwired: 1 in]
          n129 = Index Array(array=w405, index (row)=3) -> (element=w399:dbl[])  [unwired: 1 in]
          n130 = Index Array(array=w405, index (row)=6) -> (element=w395:dbl[])  [unwired: 1 in]
          n131 = Index Array(array=w405, index (row)=7) -> (element=w417:dbl[])  [unwired: 1 in]
          n132 = Index Array(array=w405, index (row)=9) -> (element=w415:dbl[])  [unwired: 1 in]
          n133 = Index Array(array=w405, index (row)=8) -> (element=w416:dbl[])  [unwired: 1 in]
          n134 = Index Array(array=w405, index (row)=10) -> (element=w414:dbl[])  [unwired: 1 in]
          n135 = Index Array(array=w405, index (row)=11) -> (element=w403:dbl[])  [unwired: 1 in]
          n136 = Index Array(array=w405, index (row)=12) -> (element=w400:dbl[])  [unwired: 1 in]
          n137 = Index Array(array=w405, index (row)=13) -> (element=w397:dbl[])  [unwired: 1 in]
          n138 = Index Array(array=w405, index (row)=14) -> (element=w413:dbl[])  [unwired: 1 in]
          n139 = Index Array(array=w405, index (row)=15) -> (element=w412:dbl[])  [unwired: 1 in]
          n140 = Index Array(array=w405, index (row)=21) -> (element=w394:dbl[])  [unwired: 1 in]
          n141 = Index Array(array=w405, index (row)=23) -> (element=w393:dbl[])  [unwired: 1 in]
          n142 = Index Array(array=w405, index (row)=25) -> (element=w392:dbl[])  [unwired: 1 in]
          n143 = Index Array(array=w405, index (row)=29) -> (element=w390:dbl[])  [unwired: 1 in]
          n144 = Index Array(array=w405, index (row)=31) -> (element=w389:dbl[])  [unwired: 1 in]
          n145 = Index Array(array=w405, index (row)=27) -> (element=w391:dbl[])  [unwired: 1 in]
        }
        frame #2 {
          n146 = case shown="\"Multiple IR\"" "IR Setting" {
            tunnel: w444 -> [_ w3641]
            tunnel: [w3637 w3640] -> w443
            frame "Single IR", Default {
              n147 = Decimal String To Number(string="Internal Resistor", default (0L)=0.0 ("y")) -> (number=w3637:dbl)  [unwired: 1 in, 1 out]
            }
            frame "Multiple IR" {
              n148 = Less?(x="High Freq  (Hz)\nFor IR Switch", y=w3641) -> (x < y?=w3644:bool)
              n149 = Less?(x="Low Freq (Hz) \nFor IR Switch", y=w3641) -> (x < y?=w3642:bool)
              n150 = case shown="False" w3642 {
                tunnel: w3644 -> [_ w3650]
                tunnel: [w3646 w3649] -> w3640
                frame False {
                  n151 = Decimal String To Number(string="IR Low Freq", default (0L)=0.0 ("y")) -> (number=w3646:dbl)  [unwired: 1 in, 1 out]
                }
                frame True {
                  n152 = case shown="True" w3650 {
                    tunnel: [w3651 w3655] -> w3649
                    frame False {
                      n153 = Decimal String To Number(string="IR Mid Freq", default (0L)=0.0 ("y")) -> (number=w3651:dbl)  [unwired: 1 in, 1 out]
                    }
                    frame True {
                      n154 = Decimal String To Number(string="IR High Freq", default (0L)=0.0 ("y")) -> (number=w3655:dbl)  [unwired: 1 in, 1 out]
                    }
                  }
                }
              }
            }
          }
          n155 = Decimal String To Number(string="Current Signal Amplification") -> (number=w476:i32)  [unwired: 2 in, 1 out]
          n156 = Decimal String To Number(string="Voltage Signal Amplification") -> (number=w474:i32)  [unwired: 2 in, 1 out]
          n157 = case shown="True" w478 {
            tunnel: w443 -> [w3660 w3664]
            tunnel: w476 -> [w3659 w3663]
            tunnel: [w3658 w3662] -> w445
            tunnel: w474 -> [w3658 w3661]
            tunnel: [w3657 w3661] -> w473
            frame False {
              # "Potentiostatic"
              n158 = Multiply(x=w3660, y=w3659) -> (x*y=w3657:dbl)
            }
            frame True {
              # "Galvanostatic"
              n159 = Multiply(x=w3664, y=w3663) -> (x*y=w3662:dbl)
            }
          }
          n160 = while {
            tunnel: [w577] -> w494
            tunnel: [w622] -> w493
            tunnel: [w621] -> w492
            tunnel: [w620] -> w491
            tunnel: [w619] -> w490
            tunnel: [w618] -> w489
            tunnel: [w617] -> w488
            tunnel: [w616] -> w487
            tunnel: [w615] -> w486
            tunnel: [w614] -> w485
            tunnel: [w613] -> w484
            tunnel: [w612] -> w483
            tunnel: [w576] -> w482
            tunnel: [w611] -> w481
            tunnel: [w610] -> w480
            tunnel: [w609] -> w479
            tunnel: w473 -> [w607]
            tunnel: w472 -> [w502]
            tunnel: w471 -> [w503]
            tunnel: w470 -> [w504]
            tunnel: w469 -> [w505]
            tunnel: w468 -> [w506]
            tunnel: w467 -> [w507]
            tunnel: w466 -> [w508]
            tunnel: w465 -> [w509]
            tunnel: w464 -> [w510]
            tunnel: w463 -> [w511]
            tunnel: w462 -> [w512]
            tunnel: w461 -> [w513]
            tunnel: w460 -> [w514]
            tunnel: w459 -> [w515]
            tunnel: w458 -> [w516]
            tunnel: w457 -> [w517]
            tunnel: [w606] -> w456
            tunnel: [w605] -> w455
            tunnel: [w604] -> w454
            tunnel: [w603] -> w453
            tunnel: [w602] -> w452
            tunnel: [w601] -> w451
            tunnel: [w600] -> w450
            tunnel: [w599] -> w449
            tunnel: [w598] -> w448
            tunnel: [w597] -> w447
            tunnel: w446 -> [w596]
            tunnel: w445 -> [w526]
            tunnel: w441 -> [w538]
            tunnel: w440 -> [w525]
            tunnel: w439 -> [w524]
            tunnel: w438 -> [w546]
            tunnel: w437 -> [w545]
            tunnel: w436 -> [w544]
            tunnel: [w495] -> w435
            stop <- w553 stop-if-true
            n161 = case shown="\"3 Sets of Param.\"" "Alpha Fitting Filters" {
              tunnel: ["MSE Multiplier" "V3 MSE Multiplier"] -> w608
              tunnel: ["MSE Multiplier" "V2 MSE Multiplier"] -> w559
              tunnel: ["MSE Multiplier" "V1 MSE Multiplier"] -> w558
              tunnel: [1000.0 1000.0] -> w539
              frame "1 Set of Param.", Default {
              }
              frame "3 Sets of Param." {
              }
            }
            n162 = case shown="\"3 Sets of Param.\"" "Alpha Fitting Filters" {
              tunnel: ["Amps Erase" "V1 Amps Erase"] -> w501
              tunnel: ["Amps Erase" "V2 Amps Erase"] -> w500
              tunnel: ["Amps Erase" "V3 Amps Erase"] -> w499
              frame "1 Set of Param.", Default {
              }
              frame "3 Sets of Param." {
              }
            }
            n163 = Decimal String To Number(string="Fitting Method (a)") -> (number=w536:i32)  [unwired: 2 in, 1 out]
            n164 = Divide(x="% of V22/V33", y=100.0) -> (x/y=w528:dbl)
            n165 = Bundle("Max Iterations (a)"="Max Iterations (a)", "Tolerance (a)"="Tolerance (a)") -> (w540:T4)  [unwired: 1 in]
            n166 = Divide(x="% of V11", y=100.0) -> (x/y=w532:dbl)
            n167 = Multiply(x=w526, y=10.0) -> (x*y=w523:dbl)
            n168 = case shown="False" "Weighting" {
              tunnel: w524 -> [w631 w663]
              tunnel: "V1/Alpha Amp to Noise Ratio" -> [_ w662]
              tunnel: "V2 Amp to Noise Ratio" -> [_ w661]
              tunnel: "V3 Amp to Noise Ratio" -> [_ w660]
              tunnel: [w627 w659] -> w518
              tunnel: [w626 w658] -> w519
              tunnel: [w625 w657] -> w520
              tunnel: [w624 w656] -> w534
              tunnel: [w623 w655] -> w535
              tunnel: w538 -> [_ w654]
              tunnel: w525 -> [w632 w653]
              tunnel: w546 -> [w630 w652]
              tunnel: w545 -> [w629 w651]
              tunnel: w544 -> [w628 w650]
              tunnel: "V4 Amp to Noise Ratio" -> [_ w649]
              tunnel: "V5 Amp to Noise Ratio" -> [_ w648]
              frame False {
                n169 = stacked-sequence {
                  tunnel: w632 -> [w634 _ _ _ _]
                  tunnel: w631 -> [_ w636 _ _ _]
                  tunnel: w630 -> [_ _ w640 _ _]
                  tunnel: w629 -> [_ _ _ w643 _]
                  tunnel: w628 -> [_ _ _ _ w646]
                  tunnel: [w633 _ _ _ _] -> w627
                  tunnel: [_ w637 _ _ _] -> w626
                  tunnel: [_ _ w639 _ _] -> w625
                  tunnel: [_ _ _ w642 _] -> w624
                  tunnel: [_ _ _ _ w645] -> w623
                  frame #0 {
                    n170 = for {
                      tunnel: [1.0] -> w633 mode=indexing
                      tunnel: w634 -> [_] mode=indexing
                    }
                  }
                  frame #1 {
                    n171 = for {
                      tunnel: [1.0] -> w637 mode=indexing
                      tunnel: w636 -> [_] mode=indexing
                    }
                  }
                  frame #2 {
                    n172 = for {
                      tunnel: [1.0] -> w639 mode=indexing
                      tunnel: w640 -> [_] mode=indexing
                    }
                  }
                  frame #3 {
                    n173 = for {
                      tunnel: [1.0] -> w642 mode=indexing
                      tunnel: w643 -> [_] mode=indexing
                    }
                  }
                  frame #4 {
                    n174 = for {
                      tunnel: [1.0] -> w645 mode=indexing
                      tunnel: w646 -> [_] mode=indexing
                    }
                  }
                }
              }
              frame True {
                n175 = stacked-sequence {
                  seq-local: [w665 _ _ _ _ _] -> [_ w676 w689 w701 w713 w725]
                  tunnel: w663 -> [_ _ w688 _ _ _]
                  tunnel: w662 -> [w666 w678 _ _ _ _]
                  tunnel: w661 -> [_ _ w687 _ _ _]
                  tunnel: w660 -> [_ _ _ w699 _ _]
                  tunnel: [_ _ _ _ _ w722] -> w655
                  tunnel: [_ _ _ _ w710 _] -> w656
                  tunnel: [_ _ _ w698 _ _] -> w657
                  tunnel: [_ _ w686 _ _ _] -> w658
                  tunnel: [_ w674 _ _ _ _] -> w659
                  tunnel: w654 -> [w664 _ _ _ _ _]
                  tunnel: w653 -> [_ w675 _ _ _ _]
                  tunnel: w652 -> [_ _ _ w700 _ _]
                  tunnel: w651 -> [_ _ _ _ w712 _]
                  tunnel: w650 -> [_ _ _ _ _ w724]
                  tunnel: w649 -> [_ _ _ _ w711 _]
                  tunnel: w648 -> [_ _ _ _ _ w723]
                  frame #0 {
                    n176 = Divide(x=w664, y=w666) -> (x/y=w667:dbl[])
                    n177 = for {
                      tunnel: w667 -> [w669] mode=indexing
                      tunnel: [w668] -> w665 mode=indexing
                      n178 = Greater?(x=w669, y=1.0) -> (0:w671:bool)
                      n179 = case shown="True" w671 {
                        tunnel: w669 -> [w672 _]
                        tunnel: [w672 1.0] -> w668
                        frame False {
                        }
                        frame True {
                        }
                      }
                    }
                  }
                  frame #1 {
                    n180 = Divide(x=w675, y=w678) -> (x/y=w679:dbl[])
                    n181 = for {
                      tunnel: w679 -> [w681] mode=indexing
                      tunnel: [w680] -> w677 mode=indexing
                      n182 = Greater?(x=w681, y=1.0) -> (0:w683:bool)
                      n183 = case shown="True" w683 {
                        tunnel: w681 -> [w684 _]
                        tunnel: [w684 1.0] -> w680
                        frame False {
                        }
                        frame True {
                        }
                      }
                    }
                    n184 = Multiply(x=w676, y=w677) -> (x*y=w674:dbl[])
                  }
                  frame #2 {
                    n185 = Divide(x=w688, y=w687) -> (x/y=w691:dbl[])
                    n186 = for {
                      tunnel: w691 -> [w693] mode=indexing
                      tunnel: [w692] -> w690 mode=indexing
                      n187 = Greater?(x=w693, y=1.0) -> (0:w695:bool)
                      n188 = case shown="True" w695 {
                        tunnel: w693 -> [w696 _]
                        tunnel: [w696 1.0] -> w692
                        frame False {
                        }
                        frame True {
                        }
                      }
                    }
                    n189 = Multiply(x=w689, y=w690) -> (x*y=w686:dbl[])
                  }
                  frame #3 {
                    n190 = Divide(x=w700, y=w699) -> (x/y=w703:dbl[])
                    n191 = for {
                      tunnel: w703 -> [w705] mode=indexing
                      tunnel: [w704] -> w702 mode=indexing
                      n192 = Greater?(x=w705, y=1.0) -> (0:w707:bool)
                      n193 = case shown="True" w707 {
                        tunnel: w705 -> [w708 _]
                        tunnel: [w708 1.0] -> w704
                        frame False {
                        }
                        frame True {
                        }
                      }
                    }
                    n194 = Multiply(x=w701, y=w702) -> (x*y=w698:dbl[])
                  }
                  frame #4 {
                    n195 = Divide(x=w712, y=w711) -> (x/y=w715:dbl[])
                    n196 = for {
                      tunnel: w715 -> [w717] mode=indexing
                      tunnel: [w716] -> w714 mode=indexing
                      n197 = Greater?(x=w717, y=1.0) -> (0:w719:bool)
                      n198 = case shown="True" w719 {
                        tunnel: w717 -> [w720 _]
                        tunnel: [w720 1.0] -> w716
                        frame False {
                        }
                        frame True {
                        }
                      }
                    }
                    n199 = Multiply(x=w713, y=w714) -> (x*y=w710:dbl[])
                  }
                  frame #5 {
                    n200 = Divide(x=w724, y=w723) -> (x/y=w727:dbl[])
                    n201 = for {
                      tunnel: w727 -> [w729] mode=indexing
                      tunnel: [w728] -> w726 mode=indexing
                      n202 = Greater?(x=w729, y=1.0) -> (0:w731:bool)
                      n203 = case shown="True" w731 {
                        tunnel: w729 -> [w732 _]
                        tunnel: [w732 1.0] -> w728
                        frame False {
                        }
                        frame True {
                        }
                      }
                    }
                    n204 = Multiply(x=w725, y=w726) -> (x*y=w722:dbl[])
                  }
                }
              }
            }
            n205 = Multiply(x=w535, y=w523) -> (x*y=w522:dbl[])
            n206 = Multiply(x=w534, y=w523) -> (x*y=w521:dbl[])
            n207 = stacked-sequence {
              tunnel: w607 -> [w798 w1064 w1329 w1584 w1798 w2012 w2229 w2444 w2657 w2902 w3036 w3170 w3304 w3438 w3572]
              tunnel: w503 -> [_ w1043 _ _ _ _ _ _ _ _ _ _ _ _ _]
              tunnel: w504 -> [_ _ w1308 _ _ _ _ _ _ _ _ _ _ _ _]
              tunnel: w526 -> [w794 w1061 w1327 w1581 w1795 w2009 w2226 w2441 w2654 w2906 w3040 w3174 w3308 w3442 w3576]
              tunnel: [_ w1044 _ _ _ _ _ _ _ _ _ _ _ _ _] -> w577
              tunnel: [_ _ w1309 _ _ _ _ _ _ _ _ _ _ _ _] -> w622
              tunnel: [_ w1049 _ _ _ _ _ _ _ _ _ _ _ _ _] -> w621
              tunnel: [_ _ w1314 _ _ _ _ _ _ _ _ _ _ _ _] -> w620
              tunnel: [_ w1048 _ _ _ _ _ _ _ _ _ _ _ _ _] -> w619
              tunnel: [_ _ w1313 _ _ _ _ _ _ _ _ _ _ _ _] -> w618
              tunnel: [_ _ _ _ w1789 _ _ _ _ _ _ _ _ _ _] -> w606
              tunnel: [_ _ _ _ _ w2003 _ _ _ _ _ _ _ _ _] -> w617
              tunnel: [_ _ _ _ w1794 _ _ _ _ _ _ _ _ _ _] -> w605
              tunnel: [_ _ _ _ _ w2006 _ _ _ _ _ _ _ _ _] -> w616
              tunnel: [_ _ _ _ _ _ _ w2432 _ _ _ _ _ _ _] -> w602
              tunnel: [_ _ _ _ _ _ _ _ w2645 _ _ _ _ _ _] -> w600
              tunnel: [_ _ _ _ _ _ _ w2437 _ _ _ _ _ _ _] -> w601
              tunnel: [_ _ _ _ _ _ _ _ w2650 _ _ _ _ _ _] -> w599
              tunnel: [_ _ _ _ _ _ _ _ _ _ w3015 _ _ _ _] -> w615
              tunnel: [_ _ _ _ _ _ _ _ _ _ _ w3148 _ _ _] -> w614
              tunnel: [_ _ _ _ _ _ _ _ _ _ _ _ _ w3415 _] -> w613
              tunnel: [_ _ _ _ _ _ _ _ _ _ _ _ _ _ w3549] -> w612
              tunnel: w507 -> [_ _ _ _ _ _ _ w2420 _ _ _ _ _ _ _]
              tunnel: w505 -> [_ _ _ _ w1788 _ _ _ _ _ _ _ _ _ _]
              tunnel: w506 -> [_ _ _ _ _ w2002 _ _ _ _ _ _ _ _ _]
              tunnel: w508 -> [_ _ _ _ _ _ _ _ w2644 _ _ _ _ _ _]
              tunnel: w509 -> [_ _ _ _ _ _ _ _ _ _ w3012 _ _ _ _]
              tunnel: w510 -> [_ _ _ _ _ _ _ _ _ _ _ w3146 _ _ _]
              tunnel: w511 -> [_ _ _ _ _ _ _ _ _ _ _ _ _ w3414 _]
              tunnel: w512 -> [_ _ _ _ _ _ _ _ _ _ _ _ _ _ w3548]
              tunnel: w513 -> [w774 _ _ _ _ _ _ _ _ _ _ _ _ _ _]
              tunnel: w514 -> [_ _ _ w1574 _ _ _ _ _ _ _ _ _ _ _]
              tunnel: w515 -> [_ _ _ _ _ _ w2216 _ _ _ _ _ _ _ _]
              tunnel: w516 -> [_ _ _ _ _ _ _ _ _ w2878 _ _ _ _ _]
              tunnel: w517 -> [_ _ _ _ _ _ _ _ _ _ _ _ w3280 _ _]
              tunnel: [w781 _ _ _ _ _ _ _ _ _ _ _ _ _ _] -> w576
              tunnel: [w782 _ _ _ _ _ _ _ _ _ _ _ _ _ _] -> w611
              tunnel: [_ _ _ w1578 _ _ _ _ _ _ _ _ _ _ _] -> w610
              tunnel: [_ _ _ w1577 _ _ _ _ _ _ _ _ _ _ _] -> w609
              tunnel: [_ _ _ _ _ _ w2221 _ _ _ _ _ _ _ _] -> w604
              tunnel: [_ _ _ _ _ _ w2222 _ _ _ _ _ _ _ _] -> w603
              tunnel: [_ _ _ _ _ _ _ _ _ w2880 _ _ _ _ _] -> w598
              tunnel: [_ _ _ _ _ _ _ _ _ _ _ _ w3281 _ _] -> w597
              tunnel: w608 -> [_ _ _ _ _ _ w2224 w2439 w2652 _ _ _ _ _ _]
              tunnel: w596 -> [w766 w1035 w1301 w1568 w1779 w1994 w2206 w2421 w2634 w2895 w3029 w3163 w3297 w3431 w3565]
              tunnel: [w762 _ _ _ _ _ _ _ _ _ _ _ _ _ _] -> w560
              tunnel: [_ w1029 _ _ _ _ _ _ _ _ _ _ _ _ _] -> w561
              tunnel: [_ _ w1290 _ _ _ _ _ _ _ _ _ _ _ _] -> w562
              tunnel: [_ _ _ w1560 _ _ _ _ _ _ _ _ _ _ _] -> w563
              tunnel: [_ _ _ _ w1773 _ _ _ _ _ _ _ _ _ _] -> w564
              tunnel: [_ _ _ _ _ w1987 _ _ _ _ _ _ _ _ _] -> w565
              tunnel: [_ _ _ _ _ _ w2199 _ _ _ _ _ _ _ _] -> w566
              tunnel: [_ _ _ _ _ _ _ w2415 _ _ _ _ _ _ _] -> w567
              tunnel: [_ _ _ _ _ _ _ _ w2627 _ _ _ _ _ _] -> w568
              tunnel: [_ _ _ _ _ _ _ _ _ w2837 _ _ _ _ _] -> w569
              tunnel: [_ _ _ _ _ _ _ _ _ _ w2971 _ _ _ _] -> w570
              tunnel: [_ _ _ _ _ _ _ _ _ _ _ w3106 _ _ _] -> w571
              tunnel: [_ _ _ _ _ _ _ _ _ _ _ _ w3238 _ _] -> w572
              tunnel: [_ _ _ _ _ _ _ _ _ _ _ _ _ w3374 _] -> w573
              tunnel: [_ _ _ _ _ _ _ _ _ _ _ _ _ _ w3507] -> w574
              tunnel: [w780 _ _ _ _ _ _ _ _ _ _ _ _ _ _] -> w594
              tunnel: [_ w1028 _ _ _ _ _ _ _ _ _ _ _ _ _] -> w593
              tunnel: [_ _ w1293 _ _ _ _ _ _ _ _ _ _ _ _] -> w592
              tunnel: [_ _ _ w1557 _ _ _ _ _ _ _ _ _ _ _] -> w591
              tunnel: [_ _ _ _ w1770 _ _ _ _ _ _ _ _ _ _] -> w590
              tunnel: [_ _ _ _ _ w1984 _ _ _ _ _ _ _ _ _] -> w589
              tunnel: [_ _ _ _ _ _ w2198 _ _ _ _ _ _ _ _] -> w588
              tunnel: [_ _ _ _ _ _ _ w2412 _ _ _ _ _ _ _] -> w587
              tunnel: [_ _ _ _ _ _ _ _ w2626 _ _ _ _ _ _] -> w586
              tunnel: [_ _ _ _ _ _ _ _ _ w2879 _ _ _ _ _] -> w585
              tunnel: [_ _ _ _ _ _ _ _ _ _ w2970 _ _ _ _] -> w584
              tunnel: [_ _ _ _ _ _ _ _ _ _ _ w3103 _ _ _] -> w583
              tunnel: [_ _ _ _ _ _ _ _ _ _ _ _ w3237 _ _] -> w582
              tunnel: [_ _ _ _ _ _ _ _ _ _ _ _ _ w3372 _] -> w581
              tunnel: [_ _ _ _ _ _ _ _ _ _ _ _ _ _ w3506] -> w580
              tunnel: w502 -> [w760 w1022 w1287 w1556 w1769 w1983 w2195 w2409 w2623 w2836 w2969 w3104 w3240 w3371 w3505]
              tunnel: w559 -> [_ _ _ w1622 w1836 w2050 _ _ _ _ _ _ _ _ _]
              tunnel: w558 -> [w789 w1056 w1321 _ _ _ _ _ _ _ _ _ _ _ _]
              tunnel: w518 -> [w788 w1055 w1320 _ _ _ _ _ _ _ _ _ _ _ _]
              tunnel: w519 -> [_ _ _ w1588 w1802 w2016 _ _ _ _ _ _ _ _ _]
              tunnel: w520 -> [_ _ _ _ _ _ w2223 w2438 w2651 _ _ _ _ _ _]
              tunnel: w521 -> [_ _ _ _ _ _ _ _ _ w2877 w3014 w3147 _ _ _]
              tunnel: w522 -> [_ _ _ _ _ _ _ _ _ _ _ _ w3282 w3416 w3550]
              tunnel: w540 -> [w827 w1093 w1358 w1624 w1838 w2052 w2266 w2480 w2694 w2885 w3020 w3154 w3288 w3422 w3556]
              tunnel: w539 -> [_ _ _ _ _ _ _ _ _ w2876 w3013 w3149 w3283 w3417 w3551]
              tunnel: w536 -> [_ _ _ _ _ _ _ _ _ _ _ _ _ _ _]
              tunnel: w532 -> [w790 w1057 w1322 _ _ _ _ _ _ _ _ _ _ _ _]
              tunnel: w528 -> [_ _ _ w1590 w1804 w2018 w2234 w2448 w2662 _ _ _ _ _ _]
              tunnel: w501 -> [w773 w1036 w1300 _ _ _ _ _ _ _ _ _ _ _ _]
              tunnel: w500 -> [_ _ _ w1567 w1778 w1993 _ _ _ _ _ _ _ _ _]
              tunnel: w499 -> [_ _ _ _ _ _ w2207 w2422 w2635 _ _ _ _ _ _]
              tunnel: "V13 Fitting" -> [w756 w1019 w1284 _ _ _ _ _ _ _ _ _ _ _ _]
              tunnel: "V15 & V35" -> [w755 w1018 w1283 _ _ _ w2192 w2406 w2620 _ _ _ _ _ _]
              tunnel: "V24 Fitting" -> [_ _ _ w1551 w1764 w1978 _ _ _ _ _ _ _ _ _]
              frame #0 {
                w824 = 51
                # "V1Mag"
                # "V11Mag"
                # "V13Mag"
                n208 = while {
                  shift-right: [w1014] -> _
                  shift-left: w760 -> [w1016]
                  shift-right: [w1017] -> _
                  shift-left: w774 -> [w1015]
                  tunnel: [w1017] -> w764
                  tunnel: [w1014] -> w769
                  stop <- w1012 stop-if-true
                  w1013 = 0
                  n209 = Search 1D Array(1D array=w1015, element=w1013, start index (0)=w1013) -> (index of element=w1011:i32)
                  n210 = Less Than 0?(x=w1011) -> (x < 0?=w1012:bool)
                  n211 = Delete From Array(array=w1016, index=w1011) -> (array with subset deleted=w1014:dbl[])  [unwired: 1 in, 1 out]
                  n212 = Delete From Array(array=w1015, index=w1011) -> (array with subset deleted=w1017:dbl[])  [unwired: 1 in, 1 out]
                }
                n213 = case shown="True" w766 {
                  tunnel: w769 -> [w841 w845]
                  tunnel: [w841 w844] -> w768
                  tunnel: w764 -> [w840 w843]
                  tunnel: [w840 w842] -> w767
                  frame False {
                  }
                  frame True {
                    n214 = Reverse 1D Array(array=w845) -> (reversed array=w844:dbl[])
                    n215 = Reverse 1D Array(array=w843) -> (reversed array=w842:dbl[])
                  }
                }
                n216 = Delete From Array(array=w767, length=w773) -> (array with subset deleted=w772:dbl[])  [unwired: 1 in, 1 out]
                n217 = Delete From Array(array=w772) -> (deleted portion=w779:dbl)  [unwired: 2 in, 1 out]
                n218 = Absolute Value(x=w779) -> (abs(x)=w778:dbl)
                n219 = expression code="10**floor(log(x))"(w778) -> (w796:dbl)
                n220 = Delete From Array(array=w768, length=w773) -> (array with subset deleted=w770:dbl[])  [unwired: 1 in, 1 out]
                n221 = Divide(x=w796, y=w798) -> (x/y=w795:dbl)
                n222 = Divide(x=w772, y=w796) -> (x/y=w771:dbl[])
                n223 = case shown="True" w756 {
                  tunnel: w755 -> [w851 _]
                  tunnel: w770 -> [w850 w950]
                  tunnel: w771 -> [w849 w949]
                  tunnel: [w848 w948] -> w791
                  tunnel: [w847 w947] -> w792
                  tunnel: w790 -> [w846 _]
                  frame True {
                    n224 = case shown="True" w851 {
                      tunnel: w850 -> [w854 w901]
                      tunnel: w849 -> [w879 w921]
                      tunnel: [w877 w919] -> w848
                      tunnel: [w872 w914] -> w847
                      tunnel: w846 -> [w859 w903]
                      frame True {
                        w860 = 0.0 ("y")
                        n225 = for {
                          tunnel: [w896] -> w878 mode=indexing
                          tunnel: w854 -> [w897] mode=indexing
                          tunnel: [w896] -> w866
                          n226 = Power Of X(1:w897, 2:1.0 ("y")) -> (0:w896:dbl)
                        }
                        n227 = Divide(x=w879, y=w878) -> (x/y=w876:dbl[])
                        n228 = call <vilib>:"Median.vi"("X"=w876) -> ("median"=w867:dbl)  [unwired: 1 out]
                        n229 = Multiply(x=w867, y=w866) -> (x*y=w865:dbl)
                        n230 = Delete From Array(array=w854) -> (deleted portion=w857:dbl)  [unwired: 2 in, 1 out]
                        n231 = Multiply(x=w865, y=w859) -> (x*y=w864:dbl)
                        n232 = Power Of X(1:w857, 2:3.0 ("y")) -> (0:w856:dbl)
                        n233 = Divide(x=w864, y=w856) -> (x/y=w861:dbl)
                        n234 = Delete From Array(array=w854) -> (deleted portion=w853:dbl)  [unwired: 2 in, 1 out]
                        n235 = Power Of X(1:w853, 2:5.0 ("y")) -> (0:w852:dbl)
                        n236 = Divide(x=w864, y=w852) -> (x/y=w863:dbl)
                        n237 = Multiply(x=w867, y=10.0) -> (x*y=w870:dbl)
                        n238 = Build Array(w867, w860, w860) -> (w877:dbl[])
                        n239 = Greater Than 0?(x=w867) -> (x > 0?=w871:bool)
                        n240 = Negate(x=w863) -> (-x=w869:dbl)
                        n241 = Negate(x=w861) -> (-x=w862:dbl)
                        n242 = case shown="True" w871 {
                          tunnel: [w887 w895] -> w874
                          tunnel: [w886 w894] -> w873
                          tunnel: w870 -> [w884 w893]
                          tunnel: w869 -> [w883 w891]
                          tunnel: 0.0 ("y") -> [w885 w892]
                          tunnel: w863 -> [w882 w890]
                          tunnel: w862 -> [w881 w888]
                          tunnel: w861 -> [w880 w889]
                          frame True {
                            n243 = Build Array(w885, w881, w883) -> (w887:dbl[])
                            n244 = Build Array(w884, w880, w882) -> (w886:dbl[])
                          }
                          frame False {
                            n245 = Build Array(w892, w888, w891) -> (w894:dbl[])
                            n246 = Build Array(w893, w889, w890) -> (w895:dbl[])
                          }
                        }
                        n247 = Bundle(w874, w873) -> (w872:cluster{dbl[], dbl[]})  [unwired: 1 in]
                      }
                      frame False {
                        w904 = 0.0 ("y")
                        n248 = for {
                          tunnel: [w934] -> w920 mode=indexing
                          tunnel: w901 -> [w935] mode=indexing
                          tunnel: [w934] -> w909
                          n249 = Power Of X(1:w935, 2:1.0 ("y")) -> (0:w934:dbl)
                        }
                        n250 = Divide(x=w921, y=w920) -> (x/y=w918:dbl[])
                        n251 = call <vilib>:"Median.vi"("X"=w918) -> ("median"=w910:dbl)  [unwired: 1 out]
                        n252 = Multiply(x=w910, y=w909) -> (x*y=w908:dbl)
                        n253 = Multiply(x=w908, y=w903) -> (x*y=w907:dbl)
                        n254 = Delete From Array(array=w901) -> (deleted portion=w900:dbl)  [unwired: 2 in, 1 out]
                        n255 = Power Of X(1:w900, 2:3.0 ("y")) -> (0:w899:dbl)
                        n256 = Divide(x=w907, y=w899) -> (x/y=w905:dbl)
                        n257 = Multiply(x=w910, y=10.0) -> (x*y=w912:dbl)
                        n258 = Build Array(w910, w904, w904) -> (w919:dbl[])
                        n259 = Greater Than 0?(x=w910) -> (x > 0?=w913:bool)
                        n260 = Negate(x=w905) -> (-x=w906:dbl)
                        n261 = case shown="True" w913 {
                          tunnel: [w927 w933] -> w916
                          tunnel: [w926 w932] -> w915
                          tunnel: w912 -> [w925 w931]
                          tunnel: 0.0 ("y") -> [w922 w928]
                          tunnel: w906 -> [w924 w929]
                          tunnel: w905 -> [w923 w930]
                          frame True {
                            n262 = Build Array(w922, w924, w922) -> (w927:dbl[])
                            n263 = Build Array(w925, w923, w922) -> (w926:dbl[])
                          }
                          frame False {
                            n264 = Build Array(w928, w929, w928) -> (w932:dbl[])
                            n265 = Build Array(w931, w930, w928) -> (w933:dbl[])
                          }
                        }
                        n266 = Bundle(w916, w915) -> (w914:cluster{dbl[], dbl[]})  [unwired: 1 in]
                      }
                    }
                  }
                  frame False {
                    w937 = 0.0 ("y")
                    n267 = for {
                      tunnel: [w959] -> w946 mode=indexing
                      tunnel: w950 -> [w960] mode=indexing
                      n268 = Power Of X(1:w960, 2:1.0 ("y")) -> (0:w959:dbl)
                    }
                    n269 = Divide(x=w949, y=w946) -> (x/y=w945:dbl[])
                    n270 = call <vilib>:"Median.vi"("X"=w945) -> ("median"=w938:dbl)  [unwired: 1 out]
                    n271 = Multiply(x=w938, y=10.0) -> (x*y=w940:dbl)
                    n272 = Build Array(w938, w937, w937) -> (w948:dbl[])
                    n273 = Greater Than 0?(x=w938) -> (x > 0?=w941:bool)
                    n274 = case shown="False" w941 {
                      tunnel: [w954 w958] -> w943
                      tunnel: [w953 w957] -> w942
                      tunnel: w940 -> [w952 w956]
                      tunnel: 0.0 ("y") -> [w951 w955]
                      frame True {
                        n275 = Build Array(w951, w951, w951) -> (w954:dbl[])
                        n276 = Build Array(w952, w951, w951) -> (w953:dbl[])
                      }
                      frame False {
                        n277 = Build Array(w955, w955, w955) -> (w957:dbl[])
                        n278 = Build Array(w956, w955, w955) -> (w958:dbl[])
                      }
                    }
                    n279 = Bundle(w943, w942) -> (w947:cluster{dbl[], dbl[]})  [unwired: 1 in]
                  }
                }
                n280 = vi-ref "V1fit.vi"() -> (w787:refnum<vi>)
                n281 = Insert Into Array(array=w788, index=0, new element=1.0 ("new element/subarray")) -> (w803:dbl[])
                n282 = Insert Into Array(array=w771, index=0, new element=0.0 ("new element/subarray")) -> (w808:dbl[])
                n283 = Insert Into Array(array=w770, index=0, new element=0.0 ("new element/subarray")) -> (w807:dbl[])
                n284 = Decrement(x=w824) -> (x-1=w823:i32)
                n285 = call-poly <vilib>:"Constrained Nonlinear Curve Fit.vi"("Y"=w808, "f(x,a)"=w787, "X"=w807, "Weight"=w803, "initial parameters"=w791, "termination"=w827, "parameter bounds"=w792) -> ("best nonlinear fit"=w830:dbl[], "residue"=w831:dbl)  [unwired: 3 in, 4 out]
                n286 = Subtract(x=w808, y=w830) -> (x-y=w805:dbl[])
                n287 = Multiply(x=w831, y=w789) -> (x*y=w839:dbl)
                n288 = Square Root(x=w839) -> (sqrt(x)=w804:dbl)
                n289 = for {
                  tunnel: w805 -> [w979] mode=indexing
                  tunnel: w804 -> [w980]
                  tunnel: w807 -> [w976] mode=indexing
                  tunnel: w808 -> [w975] mode=indexing
                  tunnel: [w974] -> w776 mode=indexing
                  tunnel: [w973] -> w806 mode=indexing
                  tunnel: w803 -> [w972] mode=indexing
                  tunnel: [w971] -> w802 mode=indexing
                  n290 = Absolute Value(x=w979) -> (abs(x)=w978:dbl)
                  n291 = Greater?(x=w978, y=w980) -> (0:w977:bool)
                  n292 = case shown="False" w977 {
                    tunnel: w976 -> [w983 _]
                    tunnel: w975 -> [w982 _]
                    tunnel: [w983 w984] -> w974
                    tunnel: [w982 w984] -> w973
                    tunnel: w972 -> [w981 _]
                    tunnel: [w981 w984] -> w971
                    frame False {
                    }
                    frame True {
                      w984 = 0.0
                    }
                  }
                }
                n293 = while {
                  shift-right: [w967] -> _
                  shift-left: w776 -> [w969]
                  shift-right: [w970] -> _
                  shift-left: w806 -> [w968]
                  tunnel: [w970] -> w812
                  tunnel: [w967] -> w813
                  shift-right: [w963] -> w809
                  shift-left: w802 -> [w962]
                  stop <- w965 stop-if-true
                  w966 = 0
                  n294 = Search 1D Array(1D array=w968, element=w966, start index (0)=w966) -> (index of element=w964:i32)
                  n295 = Less Than 0?(x=w964) -> (x < 0?=w965:bool)
                  n296 = Delete From Array(array=w969, index=w964) -> (array with subset deleted=w967:dbl[])  [unwired: 1 in, 1 out]
                  n297 = Delete From Array(array=w962, index=w964) -> (array with subset deleted=w963:dbl[])  [unwired: 1 in, 1 out]
                  n298 = Delete From Array(array=w968, index=w964) -> (array with subset deleted=w970:dbl[])  [unwired: 1 in, 1 out]
                }
                n299 = Insert Into Array(array=w812, index=0, new element=0.0 ("new element/subarray")) -> (w799:dbl[])
                n300 = Insert Into Array(array=w809, index=0, new element=1.0 ("new element/subarray")) -> (w801:dbl[])
                n301 = Insert Into Array(array=w813, index=0, new element=0.0 ("new element/subarray")) -> (w800:dbl[])
                n302 = Divide(x=w800, y=w794) -> (x/y=w785:dbl[])
                n303 = Multiply(x=w799, y=w795) -> (x*y=w797:dbl[])
                n304 = Array Max & Min(array=w785) -> (max value=w775:dbl)  [unwired: 3 out]
                n305 = Divide(x=w775, y=w823) -> (x/y=w825:dbl)
                n306 = call-poly <vilib>:"Constrained Nonlinear Curve Fit.vi"("Y"=w799, "f(x,a)"=w787, "X"=w800, "Weight"=w801, "initial parameters"=w791, "termination"=w827, "parameter bounds"=w792) -> ("best fit parameters"=w793:dbl[])  [unwired: 3 in, 5 out]
                n307 = for {
                  N: w824 -> [_]
                  tunnel: w825 -> [w987]
                  tunnel: [w985] -> w826 mode=indexing
                  i -> [w986]
                  n308 = Multiply(x=w987, y=w986) -> (x*y=w985:dbl)
                }
                n309 = for {
                  tunnel: w826 -> [w1009] mode=indexing
                  tunnel: [w1010] -> w818 mode=indexing
                  tunnel: w793 -> [w994]
                  tunnel: [w1009] -> w786 mode=indexing
                  tunnel: w795 -> [w993]
                  tunnel: w794 -> [w989]
                  tunnel: [w988] -> w777
                  w996 = 0.0
                  n310 = Index Array(array=w994, index=1) -> (element=w1006:dbl)
                  n311 = Index Array(array=w994, index=2) -> (element=w1005:dbl)
                  n312 = Index Array(array=w994, index=0) -> (element=w992:dbl)
                  n313 = Multiply(x=w1006, y=w993) -> (x*y=w1001:dbl)
                  n314 = Multiply(x=w1005, y=w993) -> (x*y=w999:dbl)
                  n315 = Multiply(x=w992, y=w993) -> (x*y=w991:dbl)
                  n316 = Power Of X(1:w989, 2:3.0 ("y")) -> (0:w1003:dbl)
                  n317 = Power Of X(1:w989, 2:5.0 ("y")) -> (0:w1000:dbl)
                  n318 = Multiply(x=w991, y=w989) -> (x*y=w990:dbl)
                  n319 = Multiply(x=w1003, y=w1001) -> (x*y=w998:dbl)
                  n320 = Multiply(x=w1000, y=w999) -> (x*y=w997:dbl)
                  n321 = Build Array(w996, w990, w996, w998, w996, w997) -> (w988:dbl[])
                  n322 = call-poly <vilib>:"Polynomial Evaluation.vi"("P(x)"=w988, "a"=w1009) -> ("P(a)"=w1010:dbl)  [unwired: 1 out]
                }
                n323 = Array Size(array=w808) -> (size(s)=w758:i32)
                n324 = Build Cluster Array(w785, w797) -> (w821:cluster{dbl, dbl}[])
                n325 = Build Cluster Array(w786, w818) -> (w822:cluster{dbl, "P(a)":dbl}[])
                n326 = Build Cluster Array(w785, w797) -> (w820:cluster{dbl, dbl}[])
                n327 = Build Cluster Array(w786, w818) -> (w819:cluster{dbl, "P(a)":dbl}[])
                n328 = Array Size(array=w797) -> (size(s)=w762:i32)
                n329 = Array Size(array=w764) -> (size(s)=w763:i32)
                n330 = Build Cluster Array(w821, w822) -> (→"V1 Mag vs. a^1":cluster{cluster{dbl, "P(a)":dbl}[]}[])
                n331 = Decrement(x=w758) -> (x-1=w757:i32)
                n332 = Build Cluster Array(w820, w819) -> (→"V1 Mag":cluster{cluster{dbl, "P(a)":dbl}[]}[])
                n333 = Subtract(x=w758, y=w762) -> (x-y=w834:i32)
                n334 = Subtract(x=w763, y=w757) -> (x-y=w761:i32)
                n335 = Array Size(array=w760) -> (size(s)=w759:i32)
                n336 = Subtract(x=w759, y=w763) -> (x-y=w765:i32)
                n337 = Build Array(w834, w761, w765) -> (w780:i32[])
                n338 = Index Array(array=w777, index=1) -> (element=w781:dbl)
                n339 = Index Array(array=w777, index=3) -> (element=w782:dbl)
              }
              frame #1 {
                w1090 = 51
                # "V11 Re"
                # "V13 Re"
                # "V15 Re"
                # "V1 Re"
                n340 = while {
                  shift-right: [w1114] -> _
                  shift-left: w1022 -> [w1116]
                  shift-right: [w1117] -> _
                  shift-left: w1043 -> [w1115]
                  tunnel: [w1117] -> w1026
                  tunnel: [w1114] -> w1037
                  stop <- w1112 stop-if-true
                  w1113 = 0
                  n341 = Search 1D Array(1D array=w1115, element=w1113, start index (0)=w1113) -> (index of element=w1111:i32)
                  n342 = Less Than 0?(x=w1111) -> (x < 0?=w1112:bool)
                  n343 = Delete From Array(array=w1116, index=w1111) -> (array with subset deleted=w1114:dbl[])  [unwired: 1 in, 1 out]
                  n344 = Delete From Array(array=w1115, index=w1111) -> (array with subset deleted=w1117:dbl[])  [unwired: 1 in, 1 out]
                }
                n345 = case shown="True" w1035 {
                  tunnel: w1037 -> [w1106 w1110]
                  tunnel: [w1106 w1109] -> w1039
                  tunnel: w1026 -> [w1105 w1108]
                  tunnel: [w1105 w1107] -> w1038
                  frame False {
                  }
                  frame True {
                    n346 = Reverse 1D Array(array=w1110) -> (reversed array=w1109:dbl[])
                    n347 = Reverse 1D Array(array=w1108) -> (reversed array=w1107:dbl[])
                  }
                }
                n348 = Delete From Array(array=w1038, length=w1036) -> (array with subset deleted=w1040:dbl[])  [unwired: 1 in, 1 out]
                n349 = Delete From Array(array=w1040) -> (deleted portion=w1042:dbl)  [unwired: 2 in, 1 out]
                n350 = Absolute Value(x=w1042) -> (abs(x)=w1041:dbl)
                n351 = expression code="10**floor(log(x))"(w1041) -> (w1034:dbl)
                n352 = Delete From Array(array=w1039, length=w1036) -> (array with subset deleted=w1032:dbl[])  [unwired: 1 in, 1 out]
                n353 = Divide(x=w1034, y=w1064) -> (x/y=w1062:dbl)
                n354 = Divide(x=w1040, y=w1034) -> (x/y=w1033:dbl[])
                n355 = case shown="True" w1019 {
                  tunnel: w1018 -> [w1123 _]
                  tunnel: w1032 -> [w1122 w1222]
                  tunnel: w1033 -> [w1121 w1221]
                  tunnel: [w1120 w1220] -> w1058
                  tunnel: [w1119 w1219] -> w1059
                  tunnel: w1057 -> [w1118 _]
                  frame True {
                    n356 = case shown="True" w1123 {
                      tunnel: w1122 -> [w1126 w1173]
                      tunnel: w1121 -> [w1151 w1193]
                      tunnel: [w1149 w1191] -> w1120
                      tunnel: [w1144 w1186] -> w1119
                      tunnel: w1118 -> [w1131 w1175]
                      frame True {
                        w1132 = 0.0 ("y")
                        n357 = for {
                          tunnel: [w1168] -> w1150 mode=indexing
                          tunnel: w1126 -> [w1169] mode=indexing
                          tunnel: [w1168] -> w1138
                          n358 = Power Of X(1:w1169, 2:1.0 ("y")) -> (0:w1168:dbl)
                        }
                        n359 = Divide(x=w1151, y=w1150) -> (x/y=w1148:dbl[])
                        n360 = call <vilib>:"Median.vi"("X"=w1148) -> ("median"=w1139:dbl)  [unwired: 1 out]
                        n361 = Multiply(x=w1139, y=w1138) -> (x*y=w1137:dbl)
                        n362 = Delete From Array(array=w1126) -> (deleted portion=w1129:dbl)  [unwired: 2 in, 1 out]
                        n363 = Multiply(x=w1137, y=w1131) -> (x*y=w1136:dbl)
                        n364 = Power Of X(1:w1129, 2:3.0 ("y")) -> (0:w1128:dbl)
                        n365 = Divide(x=w1136, y=w1128) -> (x/y=w1133:dbl)
                        n366 = Delete From Array(array=w1126) -> (deleted portion=w1125:dbl)  [unwired: 2 in, 1 out]
                        n367 = Power Of X(1:w1125, 2:5.0 ("y")) -> (0:w1124:dbl)
                        n368 = Divide(x=w1136, y=w1124) -> (x/y=w1135:dbl)
                        n369 = Multiply(x=w1139, y=10.0) -> (x*y=w1142:dbl)
                        n370 = Build Array(w1139, w1132, w1132) -> (w1149:dbl[])
                        n371 = Greater Than 0?(x=w1139) -> (x > 0?=w1143:bool)
                        n372 = Negate(x=w1135) -> (-x=w1141:dbl)
                        n373 = Negate(x=w1133) -> (-x=w1134:dbl)
                        n374 = case shown="True" w1143 {
                          tunnel: [w1159 w1167] -> w1146
                          tunnel: [w1158 w1166] -> w1145
                          tunnel: w1142 -> [w1156 w1165]
                          tunnel: w1141 -> [w1155 w1163]
                          tunnel: 0.0 ("y") -> [w1157 w1164]
                          tunnel: w1135 -> [w1154 w1162]
                          tunnel: w1134 -> [w1153 w1160]
                          tunnel: w1133 -> [w1152 w1161]
                          frame True {
                            n375 = Build Array(w1157, w1153, w1155) -> (w1159:dbl[])
                            n376 = Build Array(w1156, w1152, w1154) -> (w1158:dbl[])
                          }
                          frame False {
                            n377 = Build Array(w1164, w1160, w1163) -> (w1166:dbl[])
                            n378 = Build Array(w1165, w1161, w1162) -> (w1167:dbl[])
                          }
                        }
                        n379 = Bundle(w1146, w1145) -> (w1144:cluster{dbl[], dbl[]})  [unwired: 1 in]
                      }
                      frame False {
                        w1176 = 0.0 ("y")
                        n380 = for {
                          tunnel: [w1206] -> w1192 mode=indexing
                          tunnel: w1173 -> [w1207] mode=indexing
                          tunnel: [w1206] -> w1181
                          n381 = Power Of X(1:w1207, 2:1.0 ("y")) -> (0:w1206:dbl)
                        }
                        n382 = Divide(x=w1193, y=w1192) -> (x/y=w1190:dbl[])
                        n383 = call <vilib>:"Median.vi"("X"=w1190) -> ("median"=w1182:dbl)  [unwired: 1 out]
                        n384 = Multiply(x=w1182, y=w1181) -> (x*y=w1180:dbl)
                        n385 = Multiply(x=w1180, y=w1175) -> (x*y=w1179:dbl)
                        n386 = Delete From Array(array=w1173) -> (deleted portion=w1172:dbl)  [unwired: 2 in, 1 out]
                        n387 = Power Of X(1:w1172, 2:3.0 ("y")) -> (0:w1171:dbl)
                        n388 = Divide(x=w1179, y=w1171) -> (x/y=w1177:dbl)
                        n389 = Multiply(x=w1182, y=10.0) -> (x*y=w1184:dbl)
                        n390 = Build Array(w1182, w1176, w1176) -> (w1191:dbl[])
                        n391 = Greater Than 0?(x=w1182) -> (x > 0?=w1185:bool)
                        n392 = Negate(x=w1177) -> (-x=w1178:dbl)
                        n393 = case shown="True" w1185 {
                          tunnel: [w1199 w1205] -> w1188
                          tunnel: [w1198 w1204] -> w1187
                          tunnel: w1184 -> [w1197 w1203]
                          tunnel: 0.0 ("y") -> [w1194 w1200]
                          tunnel: w1178 -> [w1196 w1201]
                          tunnel: w1177 -> [w1195 w1202]
                          frame True {
                            n394 = Build Array(w1194, w1196, w1194) -> (w1199:dbl[])
                            n395 = Build Array(w1197, w1195, w1194) -> (w1198:dbl[])
                          }
                          frame False {
                            n396 = Build Array(w1200, w1201, w1200) -> (w1204:dbl[])
                            n397 = Build Array(w1203, w1202, w1200) -> (w1205:dbl[])
                          }
                        }
                        n398 = Bundle(w1188, w1187) -> (w1186:cluster{dbl[], dbl[]})  [unwired: 1 in]
                      }
                    }
                  }
                  frame False {
                    w1209 = 0.0 ("y")
                    n399 = for {
                      tunnel: [w1231] -> w1218 mode=indexing
                      tunnel: w1222 -> [w1232] mode=indexing
                      n400 = Power Of X(1:w1232, 2:1.0 ("y")) -> (0:w1231:dbl)
                    }
                    n401 = Divide(x=w1221, y=w1218) -> (x/y=w1217:dbl[])
                    n402 = call <vilib>:"Median.vi"("X"=w1217) -> ("median"=w1210:dbl)  [unwired: 1 out]
                    n403 = Multiply(x=w1210, y=10.0) -> (x*y=w1212:dbl)
                    n404 = Build Array(w1210, w1209, w1209) -> (w1220:dbl[])
                    n405 = Greater Than 0?(x=w1210) -> (x > 0?=w1213:bool)
                    n406 = case shown="False" w1213 {
                      tunnel: [w1226 w1230] -> w1215
                      tunnel: [w1225 w1229] -> w1214
                      tunnel: w1212 -> [w1224 w1228]
                      tunnel: 0.0 ("y") -> [w1223 w1227]
                      frame True {
                        n407 = Build Array(w1223, w1223, w1223) -> (w1226:dbl[])
                        n408 = Build Array(w1224, w1223, w1223) -> (w1225:dbl[])
                      }
                      frame False {
                        n409 = Build Array(w1227, w1227, w1227) -> (w1229:dbl[])
                        n410 = Build Array(w1228, w1227, w1227) -> (w1230:dbl[])
                      }
                    }
                    n411 = Bundle(w1215, w1214) -> (w1219:cluster{dbl[], dbl[]})  [unwired: 1 in]
                  }
                }
                n412 = vi-ref "V1fit.vi"() -> (w1054:refnum<vi>)
                n413 = Insert Into Array(array=w1055, index=0, new element=1.0 ("new element/subarray")) -> (w1069:dbl[])
                n414 = Insert Into Array(array=w1033, index=0, new element=0.0 ("new element/subarray")) -> (w1027:dbl[])
                n415 = Insert Into Array(array=w1032, index=0, new element=0.0 ("new element/subarray")) -> (w1074:dbl[])
                n416 = Decrement(x=w1090) -> (x-1=w1089:i32)
                n417 = call-poly <vilib>:"Constrained Nonlinear Curve Fit.vi"("Y"=w1027, "f(x,a)"=w1054, "X"=w1074, "Weight"=w1069, "initial parameters"=w1058, "termination"=w1093, "parameter bounds"=w1059) -> ("best nonlinear fit"=w1096:dbl[], "residue"=w1097:dbl)  [unwired: 3 in, 4 out]
                n418 = Subtract(x=w1027, y=w1096) -> (x-y=w1071:dbl[])
                n419 = Multiply(x=w1097, y=w1056) -> (x*y=w1104:dbl)
                n420 = Square Root(x=w1104) -> (sqrt(x)=w1070:dbl)
                n421 = for {
                  tunnel: w1071 -> [w1251] mode=indexing
                  tunnel: w1070 -> [w1252]
                  tunnel: w1074 -> [w1248] mode=indexing
                  tunnel: w1027 -> [w1247] mode=indexing
                  tunnel: [w1246] -> w1072 mode=indexing
                  tunnel: [w1245] -> w1073 mode=indexing
                  tunnel: w1069 -> [w1244] mode=indexing
                  tunnel: [w1243] -> w1068 mode=indexing
                  n422 = Absolute Value(x=w1251) -> (abs(x)=w1250:dbl)
                  n423 = Greater?(x=w1250, y=w1252) -> (0:w1249:bool)
                  n424 = case shown="False" w1249 {
                    tunnel: w1248 -> [w1255 _]
                    tunnel: w1247 -> [w1254 _]
                    tunnel: [w1255 w1256] -> w1246
                    tunnel: [w1254 w1256] -> w1245
                    tunnel: w1244 -> [w1253 _]
                    tunnel: [w1253 w1256] -> w1243
                    frame False {
                    }
                    frame True {
                      w1256 = 0.0
                    }
                  }
                }
                n425 = while {
                  shift-right: [w1239] -> _
                  shift-left: w1072 -> [w1241]
                  shift-right: [w1242] -> _
                  shift-left: w1073 -> [w1240]
                  tunnel: [w1242] -> w1078
                  tunnel: [w1239] -> w1079
                  shift-right: [w1235] -> w1075
                  shift-left: w1068 -> [w1234]
                  stop <- w1237 stop-if-true
                  w1238 = 0
                  n426 = Search 1D Array(1D array=w1240, element=w1238, start index (0)=w1238) -> (index of element=w1236:i32)
                  n427 = Less Than 0?(x=w1236) -> (x < 0?=w1237:bool)
                  n428 = Delete From Array(array=w1241, index=w1236) -> (array with subset deleted=w1239:dbl[])  [unwired: 1 in, 1 out]
                  n429 = Delete From Array(array=w1234, index=w1236) -> (array with subset deleted=w1235:dbl[])  [unwired: 1 in, 1 out]
                  n430 = Delete From Array(array=w1240, index=w1236) -> (array with subset deleted=w1242:dbl[])  [unwired: 1 in, 1 out]
                }
                n431 = Insert Into Array(array=w1078, index=0, new element=0.0 ("new element/subarray")) -> (w1065:dbl[])
                n432 = Insert Into Array(array=w1075, index=0, new element=1.0 ("new element/subarray")) -> (w1067:dbl[])
                n433 = Insert Into Array(array=w1079, index=0, new element=0.0 ("new element/subarray")) -> (w1066:dbl[])
                n434 = Divide(x=w1066, y=w1061) -> (x/y=w1052:dbl[])
                n435 = Multiply(x=w1065, y=w1062) -> (x*y=w1063:dbl[])
                n436 = Array Max & Min(array=w1052) -> (max value=w1045:dbl)  [unwired: 3 out]
                n437 = Divide(x=w1045, y=w1089) -> (x/y=w1091:dbl)
                n438 = call-poly <vilib>:"Constrained Nonlinear Curve Fit.vi"("Y"=w1065, "f(x,a)"=w1054, "X"=w1066, "Weight"=w1067, "initial parameters"=w1058, "termination"=w1093, "parameter bounds"=w1059) -> ("best fit parameters"=w1047:dbl[])  [unwired: 3 in, 5 out]
                n439 = for {
                  N: w1090 -> [_]
                  tunnel: w1091 -> [w1259]
                  tunnel: [w1257] -> w1092 mode=indexing
                  i -> [w1258]
                  n440 = Multiply(x=w1259, y=w1258) -> (x*y=w1257:dbl)
                }
                n441 = for {
                  tunnel: w1092 -> [w1281] mode=indexing
                  tunnel: [w1282] -> w1084 mode=indexing
                  tunnel: w1047 -> [w1266]
                  tunnel: [w1281] -> w1053 mode=indexing
                  tunnel: w1062 -> [w1265]
                  tunnel: w1061 -> [w1261]
                  tunnel: [w1260] -> w1046
                  w1268 = 0.0
                  n442 = Index Array(array=w1266, index=1) -> (element=w1278:dbl)
                  n443 = Index Array(array=w1266, index=2) -> (element=w1277:dbl)
                  n444 = Index Array(array=w1266, index=0) -> (element=w1264:dbl)
                  n445 = Multiply(x=w1278, y=w1265) -> (x*y=w1273:dbl)
                  n446 = Multiply(x=w1277, y=w1265) -> (x*y=w1271:dbl)
                  n447 = Multiply(x=w1264, y=w1265) -> (x*y=w1263:dbl)
                  n448 = Power Of X(1:w1261, 2:3.0 ("y")) -> (0:w1275:dbl)
                  n449 = Power Of X(1:w1261, 2:5.0 ("y")) -> (0:w1272:dbl)
                  n450 = Multiply(x=w1263, y=w1261) -> (x*y=w1262:dbl)
                  n451 = Multiply(x=w1275, y=w1273) -> (x*y=w1270:dbl)
                  n452 = Multiply(x=w1272, y=w1271) -> (x*y=w1269:dbl)
                  n453 = Build Array(w1268, w1262, w1268, w1270, w1268, w1269) -> (w1260:dbl[])
                  n454 = call-poly <vilib>:"Polynomial Evaluation.vi"("P(x)"=w1260, "a"=w1281) -> ("P(a)"=w1282:dbl)  [unwired: 1 out]
                }
                n455 = Array Size(array=w1027) -> (size(s)=w1030:i32)
                n456 = Build Cluster Array(w1052, w1063) -> (w1087:cluster{dbl, dbl}[])
                n457 = Build Cluster Array(w1053, w1084) -> (w1088:cluster{dbl, "P(a)":dbl}[])
                n458 = Build Cluster Array(w1052, w1063) -> (w1086:cluster{dbl, dbl}[])
                n459 = Build Cluster Array(w1053, w1084) -> (w1085:cluster{dbl, "P(a)":dbl}[])
                n460 = Array Size(array=w1063) -> (size(s)=w1029:i32)
                n461 = Array Size(array=w1026) -> (size(s)=w1024:i32)
                n462 = Decrement(x=w1030) -> (x-1=w1021:i32)
                n463 = Build Cluster Array(w1087, w1088) -> (→"V1 Re vs. a^1":cluster{cluster{dbl, "P(a)":dbl}[]}[])
                n464 = Build Cluster Array(w1086, w1085) -> (→"V1 Re":cluster{cluster{dbl, "P(a)":dbl}[]}[])
                n465 = Subtract(x=w1030, y=w1029) -> (x-y=w1031:i32)
                n466 = Subtract(x=w1024, y=w1021) -> (x-y=w1025:i32)
                n467 = Array Size(array=w1022) -> (size(s)=w1020:i32)
                n468 = Subtract(x=w1020, y=w1024) -> (x-y=w1023:i32)
                n469 = Build Array(w1031, w1025, w1023) -> (w1028:i32[])
                n470 = Index Array(array=w1046, index=5) -> (element=w1048:dbl)
                n471 = Index Array(array=w1046, index=1) -> (element=w1044:dbl)
                n472 = Index Array(array=w1046, index=3) -> (element=w1049:dbl)
              }
              frame #2 {
                w1355 = 51
                # "V11 Im"
                # "V13 Im"
                # "V15 Im"
                # "V1 Im"
                n473 = while {
                  shift-right: [w1379] -> _
                  shift-left: w1287 -> [w1381]
                  shift-right: [w1382] -> _
                  shift-left: w1308 -> [w1380]
                  tunnel: [w1382] -> w1292
                  tunnel: [w1379] -> w1302
                  stop <- w1377 stop-if-true
                  w1378 = 0
                  n474 = Search 1D Array(1D array=w1380, element=w1378, start index (0)=w1378) -> (index of element=w1376:i32)
                  n475 = Less Than 0?(x=w1376) -> (x < 0?=w1377:bool)
                  n476 = Delete From Array(array=w1381, index=w1376) -> (array with subset deleted=w1379:dbl[])  [unwired: 1 in, 1 out]
                  n477 = Delete From Array(array=w1380, index=w1376) -> (array with subset deleted=w1382:dbl[])  [unwired: 1 in, 1 out]
                }
                n478 = case shown="True" w1301 {
                  tunnel: w1302 -> [w1371 w1375]
                  tunnel: [w1371 w1374] -> w1304
                  tunnel: w1292 -> [w1370 w1373]
                  tunnel: [w1370 w1372] -> w1303
                  frame False {
                  }
                  frame True {
                    n479 = Reverse 1D Array(array=w1375) -> (reversed array=w1374:dbl[])
                    n480 = Reverse 1D Array(array=w1373) -> (reversed array=w1372:dbl[])
                  }
                }
                n481 = Delete From Array(array=w1303, length=w1300) -> (array with subset deleted=w1305:dbl[])  [unwired: 1 in, 1 out]
                n482 = Delete From Array(array=w1305) -> (deleted portion=w1307:dbl)  [unwired: 2 in, 1 out]
                n483 = Absolute Value(x=w1307) -> (abs(x)=w1306:dbl)
                n484 = expression code="10**floor(log(x))"(w1306) -> (w1299:dbl)
                n485 = Delete From Array(array=w1304, length=w1300) -> (array with subset deleted=w1297:dbl[])  [unwired: 1 in, 1 out]
                n486 = Divide(x=w1299, y=w1329) -> (x/y=w1328:dbl)
                n487 = Divide(x=w1305, y=w1299) -> (x/y=w1298:dbl[])
                n488 = case shown="True" w1284 {
                  tunnel: w1283 -> [w1388 _]
                  tunnel: w1297 -> [w1387 w1487]
                  tunnel: w1298 -> [w1386 w1486]
                  tunnel: [w1385 w1485] -> w1323
                  tunnel: [w1384 w1484] -> w1324
                  tunnel: w1322 -> [w1383 _]
                  frame True {
                    n489 = case shown="True" w1388 {
                      tunnel: w1387 -> [w1391 w1438]
                      tunnel: w1386 -> [w1416 w1458]
                      tunnel: [w1414 w1456] -> w1385
                      tunnel: [w1409 w1451] -> w1384
                      tunnel: w1383 -> [w1396 w1440]
                      frame True {
                        w1397 = 0.0 ("y")
                        n490 = for {
                          tunnel: [w1433] -> w1415 mode=indexing
                          tunnel: w1391 -> [w1434] mode=indexing
                          tunnel: [w1433] -> w1403
                          n491 = Power Of X(1:w1434, 2:1.0 ("y")) -> (0:w1433:dbl)
                        }
                        n492 = Divide(x=w1416, y=w1415) -> (x/y=w1413:dbl[])
                        n493 = call <vilib>:"Median.vi"("X"=w1413) -> ("median"=w1404:dbl)  [unwired: 1 out]
                        n494 = Multiply(x=w1404, y=w1403) -> (x*y=w1402:dbl)
                        n495 = Delete From Array(array=w1391) -> (deleted portion=w1394:dbl)  [unwired: 2 in, 1 out]
                        n496 = Multiply(x=w1402, y=w1396) -> (x*y=w1401:dbl)
                        n497 = Power Of X(1:w1394, 2:3.0 ("y")) -> (0:w1393:dbl)
                        n498 = Divide(x=w1401, y=w1393) -> (x/y=w1398:dbl)
                        n499 = Delete From Array(array=w1391) -> (deleted portion=w1390:dbl)  [unwired: 2 in, 1 out]
                        n500 = Power Of X(1:w1390, 2:5.0 ("y")) -> (0:w1389:dbl)
                        n501 = Divide(x=w1401, y=w1389) -> (x/y=w1400:dbl)
                        n502 = Multiply(x=w1404, y=10.0) -> (x*y=w1407:dbl)
                        n503 = Build Array(w1404, w1397, w1397) -> (w1414:dbl[])
                        n504 = Greater Than 0?(x=w1404) -> (x > 0?=w1408:bool)
                        n505 = Negate(x=w1400) -> (-x=w1406:dbl)
                        n506 = Negate(x=w1398) -> (-x=w1399:dbl)
                        n507 = case shown="True" w1408 {
                          tunnel: [w1424 w1432] -> w1411
                          tunnel: [w1423 w1431] -> w1410
                          tunnel: w1407 -> [w1421 w1430]
                          tunnel: w1406 -> [w1420 w1428]
                          tunnel: 0.0 ("y") -> [w1422 w1429]
                          tunnel: w1400 -> [w1419 w1427]
                          tunnel: w1399 -> [w1418 w1425]
                          tunnel: w1398 -> [w1417 w1426]
                          frame True {
                            n508 = Build Array(w1422, w1418, w1420) -> (w1424:dbl[])
                            n509 = Build Array(w1421, w1417, w1419) -> (w1423:dbl[])
                          }
                          frame False {
                            n510 = Build Array(w1429, w1425, w1428) -> (w1431:dbl[])
                            n511 = Build Array(w1430, w1426, w1427) -> (w1432:dbl[])
                          }
                        }
                        n512 = Bundle(w1411, w1410) -> (w1409:cluster{dbl[], dbl[]})  [unwired: 1 in]
                      }
                      frame False {
                        w1441 = 0.0 ("y")
                        n513 = for {
                          tunnel: [w1471] -> w1457 mode=indexing
                          tunnel: w1438 -> [w1472] mode=indexing
                          tunnel: [w1471] -> w1446
                          n514 = Power Of X(1:w1472, 2:1.0 ("y")) -> (0:w1471:dbl)
                        }
                        n515 = Divide(x=w1458, y=w1457) -> (x/y=w1455:dbl[])
                        n516 = call <vilib>:"Median.vi"("X"=w1455) -> ("median"=w1447:dbl)  [unwired: 1 out]
                        n517 = Multiply(x=w1447, y=w1446) -> (x*y=w1445:dbl)
                        n518 = Multiply(x=w1445, y=w1440) -> (x*y=w1444:dbl)
                        n519 = Delete From Array(array=w1438) -> (deleted portion=w1437:dbl)  [unwired: 2 in, 1 out]
                        n520 = Power Of X(1:w1437, 2:3.0 ("y")) -> (0:w1436:dbl)
                        n521 = Divide(x=w1444, y=w1436) -> (x/y=w1442:dbl)
                        n522 = Multiply(x=w1447, y=10.0) -> (x*y=w1449:dbl)
                        n523 = Build Array(w1447, w1441, w1441) -> (w1456:dbl[])
                        n524 = Greater Than 0?(x=w1447) -> (x > 0?=w1450:bool)
                        n525 = Negate(x=w1442) -> (-x=w1443:dbl)
                        n526 = case shown="True" w1450 {
                          tunnel: [w1464 w1470] -> w1453
                          tunnel: [w1463 w1469] -> w1452
                          tunnel: w1449 -> [w1462 w1468]
                          tunnel: 0.0 ("y") -> [w1459 w1465]
                          tunnel: w1443 -> [w1461 w1466]
                          tunnel: w1442 -> [w1460 w1467]
                          frame True {
                            n527 = Build Array(w1459, w1461, w1459) -> (w1464:dbl[])
                            n528 = Build Array(w1462, w1460, w1459) -> (w1463:dbl[])
                          }
                          frame False {
                            n529 = Build Array(w1465, w1466, w1465) -> (w1469:dbl[])
                            n530 = Build Array(w1468, w1467, w1465) -> (w1470:dbl[])
                          }
                        }
                        n531 = Bundle(w1453, w1452) -> (w1451:cluster{dbl[], dbl[]})  [unwired: 1 in]
                      }
                    }
                  }
                  frame False {
                    w1474 = 0.0 ("y")
                    n532 = for {
                      tunnel: [w1496] -> w1483 mode=indexing
                      tunnel: w1487 -> [w1497] mode=indexing
                      n533 = Power Of X(1:w1497, 2:1.0 ("y")) -> (0:w1496:dbl)
                    }
                    n534 = Divide(x=w1486, y=w1483) -> (x/y=w1482:dbl[])
                    n535 = call <vilib>:"Median.vi"("X"=w1482) -> ("median"=w1475:dbl)  [unwired: 1 out]
                    n536 = Multiply(x=w1475, y=10.0) -> (x*y=w1477:dbl)
                    n537 = Build Array(w1475, w1474, w1474) -> (w1485:dbl[])
                    n538 = Greater Than 0?(x=w1475) -> (x > 0?=w1478:bool)
                    n539 = case shown="False" w1478 {
                      tunnel: [w1491 w1495] -> w1480
                      tunnel: [w1490 w1494] -> w1479
                      tunnel: w1477 -> [w1489 w1493]
                      tunnel: 0.0 ("y") -> [w1488 w1492]
                      frame True {
                        n540 = Build Array(w1488, w1488, w1488) -> (w1491:dbl[])
                        n541 = Build Array(w1489, w1488, w1488) -> (w1490:dbl[])
                      }
                      frame False {
                        n542 = Build Array(w1492, w1492, w1492) -> (w1494:dbl[])
                        n543 = Build Array(w1493, w1492, w1492) -> (w1495:dbl[])
                      }
                    }
                    n544 = Bundle(w1480, w1479) -> (w1484:cluster{dbl[], dbl[]})  [unwired: 1 in]
                  }
                }
                n545 = vi-ref "V1fit.vi"() -> (w1319:refnum<vi>)
                n546 = Insert Into Array(array=w1320, index=0, new element=1.0 ("new element/subarray")) -> (w1334:dbl[])
                n547 = Insert Into Array(array=w1298, index=0, new element=0.0 ("new element/subarray")) -> (w1291:dbl[])
                n548 = Insert Into Array(array=w1297, index=0, new element=0.0 ("new element/subarray")) -> (w1339:dbl[])
                n549 = Decrement(x=w1355) -> (x-1=w1354:i32)
                n550 = call-poly <vilib>:"Constrained Nonlinear Curve Fit.vi"("Y"=w1291, "f(x,a)"=w1319, "X"=w1339, "Weight"=w1334, "initial parameters"=w1323, "termination"=w1358, "parameter bounds"=w1324) -> ("best nonlinear fit"=w1361:dbl[], "residue"=w1362:dbl)  [unwired: 3 in, 4 out]
                n551 = Subtract(x=w1291, y=w1361) -> (x-y=w1336:dbl[])
                n552 = Multiply(x=w1362, y=w1321) -> (x*y=w1369:dbl)
                n553 = Square Root(x=w1369) -> (sqrt(x)=w1335:dbl)
                n554 = for {
                  tunnel: w1336 -> [w1516] mode=indexing
                  tunnel: w1335 -> [w1517]
                  tunnel: w1339 -> [w1513] mode=indexing
                  tunnel: w1291 -> [w1512] mode=indexing
                  tunnel: [w1511] -> w1337 mode=indexing
                  tunnel: [w1510] -> w1338 mode=indexing
                  tunnel: w1334 -> [w1509] mode=indexing
                  tunnel: [w1508] -> w1333 mode=indexing
                  n555 = Absolute Value(x=w1516) -> (abs(x)=w1515:dbl)
                  n556 = Greater?(x=w1515, y=w1517) -> (0:w1514:bool)
                  n557 = case shown="False" w1514 {
                    tunnel: w1513 -> [w1520 _]
                    tunnel: w1512 -> [w1519 _]
                    tunnel: [w1520 w1521] -> w1511
                    tunnel: [w1519 w1521] -> w1510
                    tunnel: w1509 -> [w1518 _]
                    tunnel: [w1518 w1521] -> w1508
                    frame False {
                    }
                    frame True {
                      w1521 = 0.0
                    }
                  }
                }
                n558 = while {
                  shift-right: [w1504] -> _
                  shift-left: w1337 -> [w1506]
                  shift-right: [w1507] -> _
                  shift-left: w1338 -> [w1505]
                  tunnel: [w1507] -> w1343
                  tunnel: [w1504] -> w1344
                  shift-right: [w1500] -> w1340
                  shift-left: w1333 -> [w1499]
                  stop <- w1502 stop-if-true
                  w1503 = 0
                  n559 = Search 1D Array(1D array=w1505, element=w1503, start index (0)=w1503) -> (index of element=w1501:i32)
                  n560 = Less Than 0?(x=w1501) -> (x < 0?=w1502:bool)
                  n561 = Delete From Array(array=w1506, index=w1501) -> (array with subset deleted=w1504:dbl[])  [unwired: 1 in, 1 out]
                  n562 = Delete From Array(array=w1499, index=w1501) -> (array with subset deleted=w1500:dbl[])  [unwired: 1 in, 1 out]
                  n563 = Delete From Array(array=w1505, index=w1501) -> (array with subset deleted=w1507:dbl[])  [unwired: 1 in, 1 out]
                }
                n564 = Insert Into Array(array=w1343, index=0, new element=0.0 ("new element/subarray")) -> (w1330:dbl[])
                n565 = Insert Into Array(array=w1340, index=0, new element=1.0 ("new element/subarray")) -> (w1332:dbl[])
                n566 = Insert Into Array(array=w1344, index=0, new element=0.0 ("new element/subarray")) -> (w1331:dbl[])
                n567 = Divide(x=w1331, y=w1327) -> (x/y=w1317:dbl[])
                n568 = Multiply(x=w1330, y=w1328) -> (x*y=w1312:dbl[])
                n569 = Array Max & Min(array=w1317) -> (max value=w1310:dbl)  [unwired: 3 out]
                n570 = Divide(x=w1310, y=w1354) -> (x/y=w1356:dbl)
                n571 = call-poly <vilib>:"Constrained Nonlinear Curve Fit.vi"("Y"=w1330, "f(x,a)"=w1319, "X"=w1331, "Weight"=w1332, "initial parameters"=w1323, "termination"=w1358, "parameter bounds"=w1324) -> ("best fit parameters"=w1325:dbl[])  [unwired: 3 in, 5 out]
                n572 = for {
                  N: w1355 -> [_]
                  tunnel: w1356 -> [w1524]
                  tunnel: [w1522] -> w1357 mode=indexing
                  i -> [w1523]
                  n573 = Multiply(x=w1524, y=w1523) -> (x*y=w1522:dbl)
                }
                n574 = for {
                  tunnel: w1357 -> [w1546] mode=indexing
                  tunnel: [w1547] -> w1349 mode=indexing
                  tunnel: w1325 -> [w1531]
                  tunnel: [w1546] -> w1318 mode=indexing
                  tunnel: w1328 -> [w1530]
                  tunnel: w1327 -> [w1526]
                  tunnel: [w1525] -> w1311
                  w1533 = 0.0
                  n575 = Index Array(array=w1531, index=1) -> (element=w1543:dbl)
                  n576 = Index Array(array=w1531, index=2) -> (element=w1542:dbl)
                  n577 = Index Array(array=w1531, index=0) -> (element=w1529:dbl)
                  n578 = Multiply(x=w1543, y=w1530) -> (x*y=w1538:dbl)
                  n579 = Multiply(x=w1542, y=w1530) -> (x*y=w1536:dbl)
                  n580 = Multiply(x=w1529, y=w1530) -> (x*y=w1528:dbl)
                  n581 = Power Of X(1:w1526, 2:3.0 ("y")) -> (0:w1540:dbl)
                  n582 = Power Of X(1:w1526, 2:5.0 ("y")) -> (0:w1537:dbl)
                  n583 = Multiply(x=w1528, y=w1526) -> (x*y=w1527:dbl)
                  n584 = Multiply(x=w1540, y=w1538) -> (x*y=w1535:dbl)
                  n585 = Multiply(x=w1537, y=w1536) -> (x*y=w1534:dbl)
                  n586 = Build Array(w1533, w1527, w1533, w1535, w1533, w1534) -> (w1525:dbl[])
                  n587 = call-poly <vilib>:"Polynomial Evaluation.vi"("P(x)"=w1525, "a"=w1546) -> ("P(a)"=w1547:dbl)  [unwired: 1 out]
                }
                n588 = Array Size(array=w1291) -> (size(s)=w1295:i32)
                n589 = Build Cluster Array(w1317, w1312) -> (w1352:cluster{dbl, dbl}[])
                n590 = Build Cluster Array(w1318, w1349) -> (w1353:cluster{dbl, "P(a)":dbl}[])
                n591 = Build Cluster Array(w1317, w1312) -> (w1351:cluster{dbl, dbl}[])
                n592 = Build Cluster Array(w1318, w1349) -> (w1350:cluster{dbl, "P(a)":dbl}[])
                n593 = Array Size(array=w1312) -> (size(s)=w1290:i32)
                n594 = Array Size(array=w1292) -> (size(s)=w1289:i32)
                n595 = Decrement(x=w1295) -> (x-1=w1286:i32)
                n596 = Build Cluster Array(w1352, w1353) -> (→"V1 Im vs. a^1":cluster{cluster{dbl, "P(a)":dbl}[]}[])
                n597 = Build Cluster Array(w1351, w1350) -> (→"V1 Im":cluster{cluster{dbl, "P(a)":dbl}[]}[])
                n598 = Subtract(x=w1295, y=w1290) -> (x-y=w1296:i32)
                n599 = Subtract(x=w1289, y=w1286) -> (x-y=w1294:i32)
                n600 = Array Size(array=w1287) -> (size(s)=w1285:i32)
                n601 = Subtract(x=w1285, y=w1289) -> (x-y=w1288:i32)
                n602 = Build Array(w1296, w1294, w1288) -> (w1293:i32[])
                n603 = Index Array(array=w1311, index=5) -> (element=w1313:dbl)
                n604 = Index Array(array=w1311, index=1) -> (element=w1309:dbl)
                n605 = Index Array(array=w1311, index=3) -> (element=w1314:dbl)
              }
              frame #3 {
                (unwired) 0 ("index")
                w1618 = 51
                # "V2 Mag"
                # "V24 Mag"
                # "V22 Mag"
                n606 = while {
                  shift-right: [w1645] -> _
                  shift-left: w1556 -> [w1647]
                  shift-right: [w1648] -> _
                  shift-left: w1574 -> [w1646]
                  tunnel: [w1648] -> w1558
                  tunnel: [w1645] -> w1564
                  stop <- w1643 stop-if-true
                  w1644 = 0
                  n607 = Search 1D Array(1D array=w1646, element=w1644, start index (0)=w1644) -> (index of element=w1642:i32)
                  n608 = Less Than 0?(x=w1642) -> (x < 0?=w1643:bool)
                  n609 = Delete From Array(array=w1647, index=w1642) -> (array with subset deleted=w1645:dbl[])  [unwired: 1 in, 1 out]
                  n610 = Delete From Array(array=w1646, index=w1642) -> (array with subset deleted=w1648:dbl[])  [unwired: 1 in, 1 out]
                }
                n611 = case shown="True" w1568 {
                  tunnel: w1564 -> [w1637 w1641]
                  tunnel: [w1637 w1640] -> w1570
                  tunnel: w1558 -> [w1636 w1639]
                  tunnel: [w1636 w1638] -> w1569
                  frame False {
                  }
                  frame True {
                    n612 = Reverse 1D Array(array=w1641) -> (reversed array=w1640:dbl[])
                    n613 = Reverse 1D Array(array=w1639) -> (reversed array=w1638:dbl[])
                  }
                }
                n614 = Delete From Array(array=w1570, length=w1567, index=0) -> (array with subset deleted=w1566:dbl[])  [unwired: 1 out]
                n615 = feedback #1() -> (w1548:dbl)  [unwired: 1 in]
                n616 = Delete From Array(array=w1569, length=w1567, index=w1548) -> (array with subset deleted=w1571:dbl[])  [unwired: 1 out]
                n617 = Delete From Array(array=w1571) -> (deleted portion=w1573:dbl)  [unwired: 2 in, 1 out]
                n618 = Absolute Value(x=w1573) -> (abs(x)=w1572:dbl)
                n619 = expression code="10**floor(log(x))"(w1572) -> (w1549:dbl)
                n620 = Divide(x=w1548, y=w1584) -> (x/y=w1582:dbl)
                n621 = Divide(x=w1571, y=w1548) -> (x/y=w1565:dbl[])
                n622 = case shown="True" w1551 {
                  tunnel: w1566 -> [w1654 w1700]
                  tunnel: w1565 -> [w1671 w1699]
                  tunnel: [w1670 w1698] -> w1592
                  tunnel: [w1669 w1697] -> w1591
                  tunnel: w1590 -> [w1651 _]
                  frame True {
                    n623 = for {
                      tunnel: [w1684] -> w1668 mode=indexing
                      tunnel: w1654 -> [w1685] mode=indexing
                      tunnel: [w1684] -> w1660
                      n624 = Power Of X(1:w1685, 2:2.0 ("y")) -> (0:w1684:dbl)
                    }
                    n625 = Divide(x=w1671, y=w1668) -> (x/y=w1667:dbl[])
                    n626 = call <vilib>:"Median.vi"("X"=w1667) -> ("median"=w1649:dbl)  [unwired: 1 out]
                    n627 = Multiply(x=w1649, y=w1660) -> (x*y=w1659:dbl)
                    n628 = Multiply(x=w1659, y=w1651) -> (x*y=w1658:dbl)
                    n629 = Delete From Array(array=w1654) -> (deleted portion=w1655:dbl)  [unwired: 2 in, 1 out]
                    n630 = Power Of X(1:w1655, 2:4.0 ("y")) -> (0:w1653:dbl)
                    n631 = Divide(x=w1658, y=w1653) -> (x/y=w1656:dbl)
                    n632 = Multiply(x=w1649, y=10.0) -> (x*y=w1662:dbl)
                    n633 = Build Array(w1649, 0.0 ("y")) -> (w1670:dbl[])
                    n634 = Greater Than 0?(x=w1649) -> (x > 0?=w1663:bool)
                    n635 = Negate(x=w1656) -> (-x=w1657:dbl)
                    n636 = case shown="True" w1663 {
                      tunnel: [w1677 w1683] -> w1665
                      tunnel: [w1676 w1682] -> w1664
                      tunnel: w1662 -> [w1675 w1681]
                      tunnel: 0.0 ("y") -> [w1672 w1678]
                      tunnel: w1657 -> [w1674 w1679]
                      tunnel: w1656 -> [w1673 w1680]
                      frame True {
                        n637 = Build Array(w1672, w1674) -> (w1677:dbl[])
                        n638 = Build Array(w1675, w1673) -> (w1676:dbl[])
                      }
                      frame False {
                        n639 = Build Array(w1678, w1679) -> (w1682:dbl[])
                        n640 = Build Array(w1681, w1680) -> (w1683:dbl[])
                      }
                    }
                    n641 = Bundle(w1665, w1664) -> (w1669:cluster{dbl[], dbl[]})  [unwired: 1 in]
                  }
                  frame False {
                    n642 = for {
                      tunnel: [w1709] -> w1696 mode=indexing
                      tunnel: w1700 -> [w1710] mode=indexing
                      n643 = Power Of X(1:w1710, 2:2.0 ("y")) -> (0:w1709:dbl)
                    }
                    n644 = Divide(x=w1699, y=w1696) -> (x/y=w1695:dbl[])
                    n645 = call <vilib>:"Median.vi"("X"=w1695) -> ("median"=w1688:dbl)  [unwired: 1 out]
                    n646 = Multiply(x=w1688, y=10.0) -> (x*y=w1690:dbl)
                    n647 = Build Array(w1688, 0.0 ("y")) -> (w1698:dbl[])
                    n648 = Greater Than 0?(x=w1688) -> (x > 0?=w1691:bool)
                    n649 = case shown="True" w1691 {
                      tunnel: [w1704 w1708] -> w1693
                      tunnel: [w1703 w1707] -> w1692
                      tunnel: w1690 -> [w1702 w1706]
                      tunnel: 0.0 ("y") -> [w1701 w1705]
                      frame True {
                        n650 = Build Array(w1701, w1701) -> (w1704:dbl[])
                        n651 = Build Array(w1702, w1701) -> (w1703:dbl[])
                      }
                      frame False {
                        n652 = Build Array(w1705, w1705) -> (w1707:dbl[])
                        n653 = Build Array(w1706, w1705) -> (w1708:dbl[])
                      }
                    }
                    n654 = Bundle(w1693, w1692) -> (w1697:cluster{dbl[], dbl[]})  [unwired: 1 in]
                  }
                }
                n655 = feedback-in #1(w1549) -> ()
                n656 = vi-ref "V2fit.vi"() -> (w1623:refnum<vi>)
                n657 = Insert Into Array(array=w1588, index=0, new element=1.0 ("new element/subarray")) -> (w1594:dbl[])
                n658 = Insert Into Array(array=w1565, index=0, new element=0.0 ("new element/subarray")) -> (w1559:dbl[])
                n659 = Insert Into Array(array=w1566, index=0, new element=0.0 ("new element/subarray")) -> (w1599:dbl[])
                n660 = Decrement(x=w1618) -> (x-1=w1617:i32)
                n661 = call-poly <vilib>:"Constrained Nonlinear Curve Fit.vi"("Y"=w1559, "f(x,a)"=w1623, "X"=w1599, "Weight"=w1594, "initial parameters"=w1592, "termination"=w1624, "parameter bounds"=w1591) -> ("best nonlinear fit"=w1627:dbl[], "residue"=w1628:dbl)  [unwired: 3 in, 4 out]
                n662 = Subtract(x=w1559, y=w1627) -> (x-y=w1596:dbl[])
                n663 = Multiply(x=w1628, y=w1622) -> (x*y=w1635:dbl)
                n664 = Square Root(x=w1635) -> (sqrt(x)=w1595:dbl)
                n665 = for {
                  tunnel: w1596 -> [w1729] mode=indexing
                  tunnel: w1595 -> [w1730]
                  tunnel: w1599 -> [w1726] mode=indexing
                  tunnel: w1559 -> [w1725] mode=indexing
                  tunnel: [w1724] -> w1597 mode=indexing
                  tunnel: [w1723] -> w1598 mode=indexing
                  tunnel: w1594 -> [w1722] mode=indexing
                  tunnel: [w1721] -> w1593 mode=indexing
                  n666 = Absolute Value(x=w1729) -> (abs(x)=w1728:dbl)
                  n667 = Greater?(x=w1728, y=w1730) -> (0:w1727:bool)
                  n668 = case shown="False" w1727 {
                    tunnel: w1726 -> [w1733 _]
                    tunnel: w1725 -> [w1732 _]
                    tunnel: [w1733 w1734] -> w1724
                    tunnel: [w1732 w1734] -> w1723
                    tunnel: w1722 -> [w1731 _]
                    tunnel: [w1731 w1734] -> w1721
                    frame False {
                    }
                    frame True {
                      w1734 = 0.0
                    }
                  }
                }
                n669 = while {
                  shift-right: [w1717] -> _
                  shift-left: w1597 -> [w1719]
                  shift-right: [w1720] -> _
                  shift-left: w1598 -> [w1718]
                  tunnel: [w1720] -> w1603
                  tunnel: [w1717] -> w1604
                  shift-right: [w1713] -> w1600
                  shift-left: w1593 -> [w1712]
                  stop <- w1715 stop-if-true
                  w1716 = 0
                  n670 = Search 1D Array(1D array=w1718, element=w1716, start index (0)=w1716) -> (index of element=w1714:i32)
                  n671 = Less Than 0?(x=w1714) -> (x < 0?=w1715:bool)
                  n672 = Delete From Array(array=w1719, index=w1714) -> (array with subset deleted=w1717:dbl[])  [unwired: 1 in, 1 out]
                  n673 = Delete From Array(array=w1712, index=w1714) -> (array with subset deleted=w1713:dbl[])  [unwired: 1 in, 1 out]
                  n674 = Delete From Array(array=w1718, index=w1714) -> (array with subset deleted=w1720:dbl[])  [unwired: 1 in, 1 out]
                }
                n675 = Insert Into Array(array=w1603, index=0, new element=0.0 ("new element/subarray")) -> (w1586:dbl[])
                n676 = Insert Into Array(array=w1600, index=0, new element=1.0 ("new element/subarray")) -> (w1589:dbl[])
                n677 = Insert Into Array(array=w1604, index=0, new element=0.0 ("new element/subarray")) -> (w1587:dbl[])
                n678 = Divide(x=w1587, y=w1581) -> (x/y=w1585:dbl[])
                n679 = Multiply(x=w1586, y=w1582) -> (x*y=w1583:dbl[])
                n680 = Array Max & Min(array=w1585) -> (max value=w1575:dbl)  [unwired: 3 out]
                n681 = Divide(x=w1575, y=w1617) -> (x/y=w1619:dbl)
                n682 = call-poly <vilib>:"Constrained Nonlinear Curve Fit.vi"("Y"=w1586, "f(x,a)"=w1623, "X"=w1587, "Weight"=w1589, "initial parameters"=w1592, "termination"=w1624, "parameter bounds"=w1591) -> ("best fit parameters"=w1611:dbl[])  [unwired: 3 in, 5 out]
                n683 = for {
                  N: w1618 -> [_]
                  tunnel: w1619 -> [w1740]
                  tunnel: [w1738] -> w1621 mode=indexing
                  i -> [w1739]
                  n684 = Multiply(x=w1740, y=w1739) -> (x*y=w1738:dbl)
                }
                n685 = for {
                  tunnel: w1621 -> [w1758] mode=indexing
                  tunnel: [w1759] -> w1610 mode=indexing
                  tunnel: w1611 -> [w1755]
                  tunnel: [w1758] -> w1609 mode=indexing
                  tunnel: w1582 -> [w1750]
                  tunnel: w1581 -> [w1742]
                  tunnel: [w1741] -> w1576
                  w1743 = 0.0
                  n686 = Index Array(array=w1755, index=0) -> (element=w1754:dbl)
                  n687 = Index Array(array=w1755, index=1) -> (element=w1753:dbl)
                  n688 = Multiply(x=w1754, y=w1750) -> (x*y=w1746:dbl)
                  n689 = Multiply(x=w1753, y=w1750) -> (x*y=w1744:dbl)
                  n690 = Power Of X(1:w1742, 2:2.0 ("y")) -> (0:w1748:dbl)
                  n691 = Power Of X(1:w1742, 2:4.0 ("y")) -> (0:w1745:dbl)
                  n692 = Multiply(x=w1748, y=w1746) -> (x*y=w1752:dbl)
                  n693 = Multiply(x=w1745, y=w1744) -> (x*y=w1751:dbl)
                  n694 = Build Array(w1743, w1743, w1752, w1743, w1751, w1743) -> (w1741:dbl[])
                  n695 = call-poly <vilib>:"Polynomial Evaluation.vi"("P(x)"=w1741, "a"=w1758) -> ("P(a)"=w1759:dbl)  [unwired: 1 out]
                }
                n696 = for {
                  tunnel: [w1761] -> w1614 mode=indexing
                  tunnel: w1585 -> [w1760] mode=indexing
                  n697 = Power Of X(1:w1760, 2:2.0 ("y")) -> (0:w1761:dbl)
                }
                n698 = for {
                  tunnel: [w1736] -> w1620 mode=indexing
                  tunnel: w1609 -> [w1735] mode=indexing
                  n699 = Power Of X(1:w1735, 2:2.0 ("y")) -> (0:w1736:dbl)
                }
                n700 = Array Size(array=w1559) -> (size(s)=w1562:i32)
                n701 = Build Cluster Array(w1614, w1583) -> (w1615:cluster{dbl, dbl}[])
                n702 = Build Cluster Array(w1620, w1610) -> (w1616:cluster{dbl, "P(a)":dbl}[])
                n703 = Build Cluster Array(w1585, w1583) -> (w1613:cluster{dbl, dbl}[])
                n704 = Build Cluster Array(w1609, w1610) -> (w1612:cluster{dbl, "P(a)":dbl}[])
                n705 = Array Size(array=w1583) -> (size(s)=w1560:i32)
                n706 = Array Size(array=w1558) -> (size(s)=w1554:i32)
                n707 = Decrement(x=w1562) -> (x-1=w1553:i32)
                n708 = Build Cluster Array(w1615, w1616) -> (→"V2 Mag vs. a^2":cluster{cluster{dbl, "P(a)":dbl}[]}[])
                n709 = Build Cluster Array(w1613, w1612) -> (→"V2 Mag":cluster{cluster{dbl, "P(a)":dbl}[]}[])
                n710 = Subtract(x=w1562, y=w1560) -> (x-y=w1563:i32)
                n711 = Subtract(x=w1554, y=w1553) -> (x-y=w1561:i32)
                n712 = Array Size(array=w1556) -> (size(s)=w1552:i32)
                n713 = Subtract(x=w1552, y=w1554) -> (x-y=w1555:i32)
                n714 = Build Array(w1563, w1561, w1555) -> (w1557:i32[])
                n715 = Index Array(array=w1576, index=2) -> (element=w1578:dbl)
                n716 = Index Array(array=w1576, index=4) -> (element=w1577:dbl)
              }
              frame #4 {
                w1763 = 0 ("index")
                w1832 = 51
                # "V22 Re"
                # "V24 Re"
                # "V2 Re"
                n717 = while {
                  shift-right: [w1859] -> _
                  shift-left: w1769 -> [w1861]
                  shift-right: [w1862] -> _
                  shift-left: w1788 -> [w1860]
                  tunnel: [w1862] -> w1771
                  tunnel: [w1859] -> w1782
                  stop <- w1857 stop-if-true
                  w1858 = 0
                  n718 = Search 1D Array(1D array=w1860, element=w1858, start index (0)=w1858) -> (index of element=w1856:i32)
                  n719 = Less Than 0?(x=w1856) -> (x < 0?=w1857:bool)
                  n720 = Delete From Array(array=w1861, index=w1856) -> (array with subset deleted=w1859:dbl[])  [unwired: 1 in, 1 out]
                  n721 = Delete From Array(array=w1860, index=w1856) -> (array with subset deleted=w1862:dbl[])  [unwired: 1 in, 1 out]
                }
                n722 = case shown="True" w1779 {
                  tunnel: w1782 -> [w1851 w1855]
                  tunnel: [w1851 w1854] -> w1784
                  tunnel: w1771 -> [w1850 w1853]
                  tunnel: [w1850 w1852] -> w1783
                  frame False {
                  }
                  frame True {
                    n723 = Reverse 1D Array(array=w1855) -> (reversed array=w1854:dbl[])
                    n724 = Reverse 1D Array(array=w1853) -> (reversed array=w1852:dbl[])
                  }
                }
                n725 = Delete From Array(array=w1783, length=w1778, index=w1763) -> (array with subset deleted=w1785:dbl[])  [unwired: 1 out]
                n726 = Delete From Array(array=w1785) -> (deleted portion=w1787:dbl)  [unwired: 2 in, 1 out]
                n727 = Absolute Value(x=w1787) -> (abs(x)=w1786:dbl)
                n728 = expression code="10**floor(log(x))"(w1786) -> (w1777:dbl)
                n729 = Delete From Array(array=w1784, length=w1778, index=w1763) -> (array with subset deleted=w1781:dbl[])  [unwired: 1 out]
                n730 = Divide(x=w1777, y=w1798) -> (x/y=w1796:dbl)
                n731 = Divide(x=w1785, y=w1777) -> (x/y=w1780:dbl[])
                n732 = case shown="True" w1764 {
                  tunnel: w1781 -> [w1868 w1914]
                  tunnel: w1780 -> [w1885 w1913]
                  tunnel: [w1884 w1912] -> w1806
                  tunnel: [w1883 w1911] -> w1805
                  tunnel: w1804 -> [w1865 _]
                  frame True {
                    n733 = for {
                      tunnel: [w1898] -> w1882 mode=indexing
                      tunnel: w1868 -> [w1899] mode=indexing
                      tunnel: [w1898] -> w1874
                      n734 = Power Of X(1:w1899, 2:2.0 ("y")) -> (0:w1898:dbl)
                    }
                    n735 = Divide(x=w1885, y=w1882) -> (x/y=w1881:dbl[])
                    n736 = call <vilib>:"Median.vi"("X"=w1881) -> ("median"=w1863:dbl)  [unwired: 1 out]
                    n737 = Multiply(x=w1863, y=w1874) -> (x*y=w1873:dbl)
                    n738 = Multiply(x=w1873, y=w1865) -> (x*y=w1872:dbl)
                    n739 = Delete From Array(array=w1868) -> (deleted portion=w1869:dbl)  [unwired: 2 in, 1 out]
                    n740 = Power Of X(1:w1869, 2:4.0 ("y")) -> (0:w1867:dbl)
                    n741 = Divide(x=w1872, y=w1867) -> (x/y=w1870:dbl)
                    n742 = Multiply(x=w1863, y=10.0) -> (x*y=w1876:dbl)
                    n743 = Build Array(w1863, 0.0 ("y")) -> (w1884:dbl[])
                    n744 = Greater Than 0?(x=w1863) -> (x > 0?=w1877:bool)
                    n745 = Negate(x=w1870) -> (-x=w1871:dbl)
                    n746 = case shown="True" w1877 {
                      tunnel: [w1891 w1897] -> w1879
                      tunnel: [w1890 w1896] -> w1878
                      tunnel: w1876 -> [w1889 w1895]
                      tunnel: 0.0 ("y") -> [w1886 w1892]
                      tunnel: w1871 -> [w1888 w1893]
                      tunnel: w1870 -> [w1887 w1894]
                      frame True {
                        n747 = Build Array(w1886, w1888) -> (w1891:dbl[])
                        n748 = Build Array(w1889, w1887) -> (w1890:dbl[])
                      }
                      frame False {
                        n749 = Build Array(w1892, w1893) -> (w1896:dbl[])
                        n750 = Build Array(w1895, w1894) -> (w1897:dbl[])
                      }
                    }
                    n751 = Bundle(w1879, w1878) -> (w1883:cluster{dbl[], dbl[]})  [unwired: 1 in]
                  }
                  frame False {
                    n752 = for {
                      tunnel: [w1923] -> w1910 mode=indexing
                      tunnel: w1914 -> [w1924] mode=indexing
                      n753 = Power Of X(1:w1924, 2:2.0 ("y")) -> (0:w1923:dbl)
                    }
                    n754 = Divide(x=w1913, y=w1910) -> (x/y=w1909:dbl[])
                    n755 = call <vilib>:"Median.vi"("X"=w1909) -> ("median"=w1902:dbl)  [unwired: 1 out]
                    n756 = Multiply(x=w1902, y=10.0) -> (x*y=w1904:dbl)
                    n757 = Build Array(w1902, 0.0 ("y")) -> (w1912:dbl[])
                    n758 = Greater Than 0?(x=w1902) -> (x > 0?=w1905:bool)
                    n759 = case shown="True" w1905 {
                      tunnel: [w1918 w1922] -> w1907
                      tunnel: [w1917 w1921] -> w1906
                      tunnel: w1904 -> [w1916 w1920]
                      tunnel: 0.0 ("y") -> [w1915 w1919]
                      frame True {
                        n760 = Build Array(w1915, w1915) -> (w1918:dbl[])
                        n761 = Build Array(w1916, w1915) -> (w1917:dbl[])
                      }
                      frame False {
                        n762 = Build Array(w1919, w1919) -> (w1921:dbl[])
                        n763 = Build Array(w1920, w1919) -> (w1922:dbl[])
                      }
                    }
                    n764 = Bundle(w1907, w1906) -> (w1911:cluster{dbl[], dbl[]})  [unwired: 1 in]
                  }
                }
                n765 = vi-ref "V2fit.vi"() -> (w1837:refnum<vi>)
                n766 = Insert Into Array(array=w1802, index=0, new element=1.0 ("new element/subarray")) -> (w1808:dbl[])
                n767 = Insert Into Array(array=w1780, index=0, new element=0.0 ("new element/subarray")) -> (w1772:dbl[])
                n768 = Insert Into Array(array=w1781, index=0, new element=0.0 ("new element/subarray")) -> (w1813:dbl[])
                n769 = Decrement(x=w1832) -> (x-1=w1831:i32)
                n770 = call-poly <vilib>:"Constrained Nonlinear Curve Fit.vi"("Y"=w1772, "f(x,a)"=w1837, "X"=w1813, "Weight"=w1808, "initial parameters"=w1806, "termination"=w1838, "parameter bounds"=w1805) -> ("best nonlinear fit"=w1841:dbl[], "residue"=w1842:dbl)  [unwired: 3 in, 4 out]
                n771 = Subtract(x=w1772, y=w1841) -> (x-y=w1810:dbl[])
                n772 = Multiply(x=w1842, y=w1836) -> (x*y=w1849:dbl)
                n773 = Square Root(x=w1849) -> (sqrt(x)=w1809:dbl)
                n774 = for {
                  tunnel: w1810 -> [w1943] mode=indexing
                  tunnel: w1809 -> [w1944]
                  tunnel: w1813 -> [w1940] mode=indexing
                  tunnel: w1772 -> [w1939] mode=indexing
                  tunnel: [w1938] -> w1811 mode=indexing
                  tunnel: [w1937] -> w1812 mode=indexing
                  tunnel: w1808 -> [w1936] mode=indexing
                  tunnel: [w1935] -> w1807 mode=indexing
                  n775 = Absolute Value(x=w1943) -> (abs(x)=w1942:dbl)
                  n776 = Greater?(x=w1942, y=w1944) -> (0:w1941:bool)
                  n777 = case shown="False" w1941 {
                    tunnel: w1940 -> [w1947 _]
                    tunnel: w1939 -> [w1946 _]
                    tunnel: [w1947 w1948] -> w1938
                    tunnel: [w1946 w1948] -> w1937
                    tunnel: w1936 -> [w1945 _]
                    tunnel: [w1945 w1948] -> w1935
                    frame False {
                    }
                    frame True {
                      w1948 = 0.0
                    }
                  }
                }
                n778 = while {
                  shift-right: [w1931] -> _
                  shift-left: w1811 -> [w1933]
                  shift-right: [w1934] -> _
                  shift-left: w1812 -> [w1932]
                  tunnel: [w1934] -> w1817
                  tunnel: [w1931] -> w1818
                  shift-right: [w1927] -> w1814
                  shift-left: w1807 -> [w1926]
                  stop <- w1929 stop-if-true
                  w1930 = 0
                  n779 = Search 1D Array(1D array=w1932, element=w1930, start index (0)=w1930) -> (index of element=w1928:i32)
                  n780 = Less Than 0?(x=w1928) -> (x < 0?=w1929:bool)
                  n781 = Delete From Array(array=w1933, index=w1928) -> (array with subset deleted=w1931:dbl[])  [unwired: 1 in, 1 out]
                  n782 = Delete From Array(array=w1926, index=w1928) -> (array with subset deleted=w1927:dbl[])  [unwired: 1 in, 1 out]
                  n783 = Delete From Array(array=w1932, index=w1928) -> (array with subset deleted=w1934:dbl[])  [unwired: 1 in, 1 out]
                }
                n784 = Insert Into Array(array=w1817, index=0, new element=0.0 ("new element/subarray")) -> (w1800:dbl[])
                n785 = Insert Into Array(array=w1814, index=0, new element=1.0 ("new element/subarray")) -> (w1803:dbl[])
                n786 = Insert Into Array(array=w1818, index=0, new element=0.0 ("new element/subarray")) -> (w1801:dbl[])
                n787 = Divide(x=w1801, y=w1795) -> (x/y=w1799:dbl[])
                n788 = Multiply(x=w1800, y=w1796) -> (x*y=w1797:dbl[])
                n789 = Array Max & Min(array=w1799) -> (max value=w1790:dbl)  [unwired: 3 out]
                n790 = Divide(x=w1790, y=w1831) -> (x/y=w1833:dbl)
                n791 = call-poly <vilib>:"Constrained Nonlinear Curve Fit.vi"("Y"=w1800, "f(x,a)"=w1837, "X"=w1801, "Weight"=w1803, "initial parameters"=w1806, "termination"=w1838, "parameter bounds"=w1805) -> ("best fit parameters"=w1825:dbl[])  [unwired: 3 in, 5 out]
                n792 = for {
                  N: w1832 -> [_]
                  tunnel: w1833 -> [w1954]
                  tunnel: [w1952] -> w1835 mode=indexing
                  i -> [w1953]
                  n793 = Multiply(x=w1954, y=w1953) -> (x*y=w1952:dbl)
                }
                n794 = for {
                  tunnel: w1835 -> [w1972] mode=indexing
                  tunnel: [w1973] -> w1824 mode=indexing
                  tunnel: w1825 -> [w1969]
                  tunnel: [w1972] -> w1823 mode=indexing
                  tunnel: w1796 -> [w1964]
                  tunnel: w1795 -> [w1956]
                  tunnel: [w1955] -> w1791
                  w1957 = 0.0
                  n795 = Index Array(array=w1969, index=0) -> (element=w1968:dbl)
                  n796 = Index Array(array=w1969, index=1) -> (element=w1967:dbl)
                  n797 = Multiply(x=w1968, y=w1964) -> (x*y=w1960:dbl)
                  n798 = Multiply(x=w1967, y=w1964) -> (x*y=w1958:dbl)
                  n799 = Power Of X(1:w1956, 2:2.0 ("y")) -> (0:w1962:dbl)
                  n800 = Power Of X(1:w1956, 2:4.0 ("y")) -> (0:w1959:dbl)
                  n801 = Multiply(x=w1962, y=w1960) -> (x*y=w1966:dbl)
                  n802 = Multiply(x=w1959, y=w1958) -> (x*y=w1965:dbl)
                  n803 = Build Array(w1957, w1957, w1966, w1957, w1965, w1957) -> (w1955:dbl[])
                  n804 = call-poly <vilib>:"Polynomial Evaluation.vi"("P(x)"=w1955, "a"=w1972) -> ("P(a)"=w1973:dbl)  [unwired: 1 out]
                }
                n805 = for {
                  tunnel: [w1975] -> w1828 mode=indexing
                  tunnel: w1799 -> [w1974] mode=indexing
                  n806 = Power Of X(1:w1974, 2:2.0 ("y")) -> (0:w1975:dbl)
                }
                n807 = for {
                  tunnel: [w1950] -> w1834 mode=indexing
                  tunnel: w1823 -> [w1949] mode=indexing
                  n808 = Power Of X(1:w1949, 2:2.0 ("y")) -> (0:w1950:dbl)
                }
                n809 = Array Size(array=w1772) -> (size(s)=w1775:i32)
                n810 = Build Cluster Array(w1828, w1797) -> (w1829:cluster{dbl, dbl}[])
                n811 = Build Cluster Array(w1834, w1824) -> (w1830:cluster{dbl, "P(a)":dbl}[])
                n812 = Build Cluster Array(w1799, w1797) -> (w1827:cluster{dbl, dbl}[])
                n813 = Build Cluster Array(w1823, w1824) -> (w1826:cluster{dbl, "P(a)":dbl}[])
                n814 = Array Size(array=w1797) -> (size(s)=w1773:i32)
                n815 = Array Size(array=w1771) -> (size(s)=w1768:i32)
                n816 = Decrement(x=w1775) -> (x-1=w1766:i32)
                n817 = Build Cluster Array(w1829, w1830) -> (→"V2 Re vs. a^2":cluster{cluster{dbl, "P(a)":dbl}[]}[])
                n818 = Build Cluster Array(w1827, w1826) -> (→"V2 Re":cluster{cluster{dbl, "P(a)":dbl}[]}[])
                n819 = Subtract(x=w1775, y=w1773) -> (x-y=w1776:i32)
                n820 = Subtract(x=w1768, y=w1766) -> (x-y=w1774:i32)
                n821 = Array Size(array=w1769) -> (size(s)=w1765:i32)
                n822 = Subtract(x=w1765, y=w1768) -> (x-y=w1767:i32)
                n823 = Build Array(w1776, w1774, w1767) -> (w1770:i32[])
                n824 = Index Array(array=w1791, index=2) -> (element=w1789:dbl)
                n825 = Index Array(array=w1791, index=4) -> (element=w1794:dbl)
              }
              frame #5 {
                w1977 = 0 ("index")
                w2046 = 51
                # "V24 Im"
                # "V22 Im"
                # "V2 Im"
                n826 = while {
                  shift-right: [w2073] -> _
                  shift-left: w1983 -> [w2075]
                  shift-right: [w2076] -> _
                  shift-left: w2002 -> [w2074]
                  tunnel: [w2076] -> w1985
                  tunnel: [w2073] -> w1991
                  stop <- w2071 stop-if-true
                  w2072 = 0
                  n827 = Search 1D Array(1D array=w2074, element=w2072, start index (0)=w2072) -> (index of element=w2070:i32)
                  n828 = Less Than 0?(x=w2070) -> (x < 0?=w2071:bool)
                  n829 = Delete From Array(array=w2075, index=w2070) -> (array with subset deleted=w2073:dbl[])  [unwired: 1 in, 1 out]
                  n830 = Delete From Array(array=w2074, index=w2070) -> (array with subset deleted=w2076:dbl[])  [unwired: 1 in, 1 out]
                }
                n831 = case shown="True" w1994 {
                  tunnel: w1991 -> [w2065 w2069]
                  tunnel: [w2065 w2068] -> w1998
                  tunnel: w1985 -> [w2064 w2067]
                  tunnel: [w2064 w2066] -> w1997
                  frame False {
                  }
                  frame True {
                    n832 = Reverse 1D Array(array=w2069) -> (reversed array=w2068:dbl[])
                    n833 = Reverse 1D Array(array=w2067) -> (reversed array=w2066:dbl[])
                  }
                }
                n834 = Delete From Array(array=w1997, length=w1993, index=w1977) -> (array with subset deleted=w1999:dbl[])  [unwired: 1 out]
                n835 = Delete From Array(array=w1999) -> (deleted portion=w2001:dbl)  [unwired: 2 in, 1 out]
                n836 = Absolute Value(x=w2001) -> (abs(x)=w2000:dbl)
                n837 = expression code="10**floor(log(x))"(w2000) -> (w1992:dbl)
                n838 = Delete From Array(array=w1998, length=w1993, index=w1977) -> (array with subset deleted=w1995:dbl[])  [unwired: 1 out]
                n839 = Divide(x=w1992, y=w2012) -> (x/y=w2010:dbl)
                n840 = Divide(x=w1999, y=w1992) -> (x/y=w1996:dbl[])
                n841 = case shown="True" w1978 {
                  tunnel: w1995 -> [w2082 w2128]
                  tunnel: w1996 -> [w2099 w2127]
                  tunnel: [w2098 w2126] -> w2020
                  tunnel: [w2097 w2125] -> w2019
                  tunnel: w2018 -> [w2079 _]
                  frame True {
                    n842 = for {
                      tunnel: [w2112] -> w2096 mode=indexing
                      tunnel: w2082 -> [w2113] mode=indexing
                      tunnel: [w2112] -> w2088
                      n843 = Power Of X(1:w2113, 2:2.0 ("y")) -> (0:w2112:dbl)
                    }
                    n844 = Divide(x=w2099, y=w2096) -> (x/y=w2095:dbl[])
                    n845 = call <vilib>:"Median.vi"("X"=w2095) -> ("median"=w2077:dbl)  [unwired: 1 out]
                    n846 = Multiply(x=w2077, y=w2088) -> (x*y=w2087:dbl)
                    n847 = Multiply(x=w2087, y=w2079) -> (x*y=w2086:dbl)
                    n848 = Delete From Array(array=w2082) -> (deleted portion=w2083:dbl)  [unwired: 2 in, 1 out]
                    n849 = Power Of X(1:w2083, 2:4.0 ("y")) -> (0:w2081:dbl)
                    n850 = Divide(x=w2086, y=w2081) -> (x/y=w2084:dbl)
                    n851 = Multiply(x=w2077, y=10.0) -> (x*y=w2090:dbl)
                    n852 = Build Array(w2077, 0.0 ("y")) -> (w2098:dbl[])
                    n853 = Greater Than 0?(x=w2077) -> (x > 0?=w2091:bool)
                    n854 = Negate(x=w2084) -> (-x=w2085:dbl)
                    n855 = case shown="True" w2091 {
                      tunnel: [w2105 w2111] -> w2093
                      tunnel: [w2104 w2110] -> w2092
                      tunnel: w2090 -> [w2103 w2109]
                      tunnel: 0.0 ("y") -> [w2100 w2106]
                      tunnel: w2085 -> [w2102 w2107]
                      tunnel: w2084 -> [w2101 w2108]
                      frame True {
                        n856 = Build Array(w2100, w2102) -> (w2105:dbl[])
                        n857 = Build Array(w2103, w2101) -> (w2104:dbl[])
                      }
                      frame False {
                        n858 = Build Array(w2106, w2107) -> (w2110:dbl[])
                        n859 = Build Array(w2109, w2108) -> (w2111:dbl[])
                      }
                    }
                    n860 = Bundle(w2093, w2092) -> (w2097:cluster{dbl[], dbl[]})  [unwired: 1 in]
                  }
                  frame False {
                    n861 = for {
                      tunnel: [w2137] -> w2124 mode=indexing
                      tunnel: w2128 -> [w2138] mode=indexing
                      n862 = Power Of X(1:w2138, 2:2.0 ("y")) -> (0:w2137:dbl)
                    }
                    n863 = Divide(x=w2127, y=w2124) -> (x/y=w2123:dbl[])
                    n864 = call <vilib>:"Median.vi"("X"=w2123) -> ("median"=w2116:dbl)  [unwired: 1 out]
                    n865 = Multiply(x=w2116, y=10.0) -> (x*y=w2118:dbl)
                    n866 = Build Array(w2116, 0.0 ("y")) -> (w2126:dbl[])
                    n867 = Greater Than 0?(x=w2116) -> (x > 0?=w2119:bool)
                    n868 = case shown="True" w2119 {
                      tunnel: [w2132 w2136] -> w2121
                      tunnel: [w2131 w2135] -> w2120
                      tunnel: w2118 -> [w2130 w2134]
                      tunnel: 0.0 ("y") -> [w2129 w2133]
                      frame True {
                        n869 = Build Array(w2129, w2129) -> (w2132:dbl[])
                        n870 = Build Array(w2130, w2129) -> (w2131:dbl[])
                      }
                      frame False {
                        n871 = Build Array(w2133, w2133) -> (w2135:dbl[])
                        n872 = Build Array(w2134, w2133) -> (w2136:dbl[])
                      }
                    }
                    n873 = Bundle(w2121, w2120) -> (w2125:cluster{dbl[], dbl[]})  [unwired: 1 in]
                  }
                }
                n874 = vi-ref "V2fit.vi"() -> (w2051:refnum<vi>)
                n875 = Insert Into Array(array=w2016, index=0, new element=1.0 ("new element/subarray")) -> (w2022:dbl[])
                n876 = Insert Into Array(array=w1996, index=0, new element=0.0 ("new element/subarray")) -> (w1986:dbl[])
                n877 = Insert Into Array(array=w1995, index=0, new element=0.0 ("new element/subarray")) -> (w2027:dbl[])
                n878 = Decrement(x=w2046) -> (x-1=w2045:i32)
                n879 = call-poly <vilib>:"Constrained Nonlinear Curve Fit.vi"("Y"=w1986, "f(x,a)"=w2051, "X"=w2027, "Weight"=w2022, "initial parameters"=w2020, "termination"=w2052, "parameter bounds"=w2019) -> ("best nonlinear fit"=w2055:dbl[], "residue"=w2056:dbl)  [unwired: 3 in, 4 out]
                n880 = Subtract(x=w1986, y=w2055) -> (x-y=w2024:dbl[])
                n881 = Multiply(x=w2056, y=w2050) -> (x*y=w2063:dbl)
                n882 = Square Root(x=w2063) -> (sqrt(x)=w2023:dbl)
                n883 = for {
                  tunnel: w2024 -> [w2157] mode=indexing
                  tunnel: w2023 -> [w2158]
                  tunnel: w2027 -> [w2154] mode=indexing
                  tunnel: w1986 -> [w2153] mode=indexing
                  tunnel: [w2152] -> w2025 mode=indexing
                  tunnel: [w2151] -> w2026 mode=indexing
                  tunnel: w2022 -> [w2150] mode=indexing
                  tunnel: [w2149] -> w2021 mode=indexing
                  n884 = Absolute Value(x=w2157) -> (abs(x)=w2156:dbl)
                  n885 = Greater?(x=w2156, y=w2158) -> (0:w2155:bool)
                  n886 = case shown="False" w2155 {
                    tunnel: w2154 -> [w2161 _]
                    tunnel: w2153 -> [w2160 _]
                    tunnel: [w2161 w2162] -> w2152
                    tunnel: [w2160 w2162] -> w2151
                    tunnel: w2150 -> [w2159 _]
                    tunnel: [w2159 w2162] -> w2149
                    frame False {
                    }
                    frame True {
                      w2162 = 0.0
                    }
                  }
                }
                n887 = while {
                  shift-right: [w2145] -> _
                  shift-left: w2025 -> [w2147]
                  shift-right: [w2148] -> _
                  shift-left: w2026 -> [w2146]
                  tunnel: [w2148] -> w2031
                  tunnel: [w2145] -> w2032
                  shift-right: [w2141] -> w2028
                  shift-left: w2021 -> [w2140]
                  stop <- w2143 stop-if-true
                  w2144 = 0
                  n888 = Search 1D Array(1D array=w2146, element=w2144, start index (0)=w2144) -> (index of element=w2142:i32)
                  n889 = Less Than 0?(x=w2142) -> (x < 0?=w2143:bool)
                  n890 = Delete From Array(array=w2147, index=w2142) -> (array with subset deleted=w2145:dbl[])  [unwired: 1 in, 1 out]
                  n891 = Delete From Array(array=w2140, index=w2142) -> (array with subset deleted=w2141:dbl[])  [unwired: 1 in, 1 out]
                  n892 = Delete From Array(array=w2146, index=w2142) -> (array with subset deleted=w2148:dbl[])  [unwired: 1 in, 1 out]
                }
                n893 = Insert Into Array(array=w2031, index=0, new element=0.0 ("new element/subarray")) -> (w2014:dbl[])
                n894 = Insert Into Array(array=w2028, index=0, new element=1.0 ("new element/subarray")) -> (w2017:dbl[])
                n895 = Insert Into Array(array=w2032, index=0, new element=0.0 ("new element/subarray")) -> (w2015:dbl[])
                n896 = Divide(x=w2015, y=w2009) -> (x/y=w2013:dbl[])
                n897 = Multiply(x=w2014, y=w2010) -> (x*y=w2011:dbl[])
                n898 = Array Max & Min(array=w2013) -> (max value=w2004:dbl)  [unwired: 3 out]
                n899 = Divide(x=w2004, y=w2045) -> (x/y=w2047:dbl)
                n900 = call-poly <vilib>:"Constrained Nonlinear Curve Fit.vi"("Y"=w2014, "f(x,a)"=w2051, "X"=w2015, "Weight"=w2017, "initial parameters"=w2020, "termination"=w2052, "parameter bounds"=w2019) -> ("best fit parameters"=w2039:dbl[])  [unwired: 3 in, 5 out]
                n901 = for {
                  N: w2046 -> [_]
                  tunnel: w2047 -> [w2168]
                  tunnel: [w2166] -> w2049 mode=indexing
                  i -> [w2167]
                  n902 = Multiply(x=w2168, y=w2167) -> (x*y=w2166:dbl)
                }
                n903 = for {
                  tunnel: w2049 -> [w2186] mode=indexing
                  tunnel: [w2187] -> w2038 mode=indexing
                  tunnel: w2039 -> [w2183]
                  tunnel: [w2186] -> w2037 mode=indexing
                  tunnel: w2010 -> [w2178]
                  tunnel: w2009 -> [w2170]
                  tunnel: [w2169] -> w2005
                  w2171 = 0.0
                  n904 = Index Array(array=w2183, index=0) -> (element=w2182:dbl)
                  n905 = Index Array(array=w2183, index=1) -> (element=w2181:dbl)
                  n906 = Multiply(x=w2182, y=w2178) -> (x*y=w2174:dbl)
                  n907 = Multiply(x=w2181, y=w2178) -> (x*y=w2172:dbl)
                  n908 = Power Of X(1:w2170, 2:2.0 ("y")) -> (0:w2176:dbl)
                  n909 = Power Of X(1:w2170, 2:4.0 ("y")) -> (0:w2173:dbl)
                  n910 = Multiply(x=w2176, y=w2174) -> (x*y=w2180:dbl)
                  n911 = Multiply(x=w2173, y=w2172) -> (x*y=w2179:dbl)
                  n912 = Build Array(w2171, w2171, w2180, w2171, w2179, w2171) -> (w2169:dbl[])
                  n913 = call-poly <vilib>:"Polynomial Evaluation.vi"("P(x)"=w2169, "a"=w2186) -> ("P(a)"=w2187:dbl)  [unwired: 1 out]
                }
                n914 = for {
                  tunnel: [w2189] -> w2042 mode=indexing
                  tunnel: w2013 -> [w2188] mode=indexing
                  n915 = Power Of X(1:w2188, 2:2.0 ("y")) -> (0:w2189:dbl)
                }
                n916 = for {
                  tunnel: [w2164] -> w2048 mode=indexing
                  tunnel: w2037 -> [w2163] mode=indexing
                  n917 = Power Of X(1:w2163, 2:2.0 ("y")) -> (0:w2164:dbl)
                }
                n918 = Array Size(array=w1986) -> (size(s)=w1989:i32)
                n919 = Build Cluster Array(w2042, w2011) -> (w2043:cluster{dbl, dbl}[])
                n920 = Build Cluster Array(w2048, w2038) -> (w2044:cluster{dbl, "P(a)":dbl}[])
                n921 = Build Cluster Array(w2013, w2011) -> (w2041:cluster{dbl, dbl}[])
                n922 = Build Cluster Array(w2037, w2038) -> (w2040:cluster{dbl, "P(a)":dbl}[])
                n923 = Array Size(array=w2011) -> (size(s)=w1987:i32)
                n924 = Array Size(array=w1985) -> (size(s)=w1982:i32)
                n925 = Decrement(x=w1989) -> (x-1=w1980:i32)
                n926 = Build Cluster Array(w2043, w2044) -> (→"V2 Im vs. a^2":cluster{cluster{dbl, "P(a)":dbl}[]}[])
                n927 = Build Cluster Array(w2041, w2040) -> (→"V2 Im":cluster{cluster{dbl, "P(a)":dbl}[]}[])
                n928 = Subtract(x=w1989, y=w1987) -> (x-y=w1990:i32)
                n929 = Subtract(x=w1982, y=w1980) -> (x-y=w1988:i32)
                n930 = Array Size(array=w1983) -> (size(s)=w1979:i32)
                n931 = Subtract(x=w1979, y=w1982) -> (x-y=w1981:i32)
                n932 = Build Array(w1990, w1988, w1981) -> (w1984:i32[])
                n933 = Index Array(array=w2005, index=2) -> (element=w2003:dbl)
                n934 = Index Array(array=w2005, index=4) -> (element=w2006:dbl)
              }
              frame #6 {
                w2191 = 0 ("index")
                w2262 = 51
                # "V35 Mag"
                # "V33 Mag"
                # "V3 Mag"
                n935 = while {
                  shift-right: [w2287] -> _
                  shift-left: w2195 -> [w2289]
                  shift-right: [w2290] -> _
                  shift-left: w2216 -> [w2288]
                  tunnel: [w2290] -> w2200
                  tunnel: [w2287] -> w2205
                  stop <- w2285 stop-if-true
                  w2286 = 0
                  n936 = Search 1D Array(1D array=w2288, element=w2286, start index (0)=w2286) -> (index of element=w2284:i32)
                  n937 = Less Than 0?(x=w2284) -> (x < 0?=w2285:bool)
                  n938 = Delete From Array(array=w2289, index=w2284) -> (array with subset deleted=w2287:dbl[])  [unwired: 1 in, 1 out]
                  n939 = Delete From Array(array=w2288, index=w2284) -> (array with subset deleted=w2290:dbl[])  [unwired: 1 in, 1 out]
                }
                n940 = case shown="True" w2206 {
                  tunnel: w2205 -> [w2279 w2283]
                  tunnel: [w2279 w2282] -> w2212
                  tunnel: w2200 -> [w2278 w2281]
                  tunnel: [w2278 w2280] -> w2211
                  frame False {
                  }
                  frame True {
                    n941 = Reverse 1D Array(array=w2283) -> (reversed array=w2282:dbl[])
                    n942 = Reverse 1D Array(array=w2281) -> (reversed array=w2280:dbl[])
                  }
                }
                n943 = Delete From Array(array=w2211, length=w2207, index=w2191) -> (array with subset deleted=w2213:dbl[])  [unwired: 1 out]
                n944 = Delete From Array(array=w2213) -> (deleted portion=w2215:dbl)  [unwired: 2 in, 1 out]
                n945 = Absolute Value(x=w2215) -> (abs(x)=w2214:dbl)
                n946 = expression code="10**floor(log(x))"(w2214) -> (w2208:dbl)
                n947 = Delete From Array(array=w2212, length=w2207, index=w2191) -> (array with subset deleted=w2210:dbl[])  [unwired: 1 out]
                n948 = Divide(x=w2208, y=w2229) -> (x/y=w2227:dbl)
                n949 = Divide(x=w2213, y=w2208) -> (x/y=w2209:dbl[])
                n950 = case shown="True" w2192 {
                  tunnel: w2210 -> [w2296 w2342]
                  tunnel: w2209 -> [w2313 w2341]
                  tunnel: [w2312 w2340] -> w2236
                  tunnel: [w2311 w2339] -> w2235
                  tunnel: w2234 -> [w2293 _]
                  frame True {
                    n951 = for {
                      tunnel: [w2326] -> w2310 mode=indexing
                      tunnel: w2296 -> [w2327] mode=indexing
                      tunnel: [w2326] -> w2302
                      n952 = Power Of X(1:w2327, 2:3.0 ("y")) -> (0:w2326:dbl)
                    }
                    n953 = Divide(x=w2313, y=w2310) -> (x/y=w2309:dbl[])
                    n954 = call <vilib>:"Median.vi"("X"=w2309) -> ("median"=w2291:dbl)  [unwired: 1 out]
                    n955 = Multiply(x=w2291, y=w2302) -> (x*y=w2301:dbl)
                    n956 = Multiply(x=w2301, y=w2293) -> (x*y=w2300:dbl)
                    n957 = Delete From Array(array=w2296) -> (deleted portion=w2297:dbl)  [unwired: 2 in, 1 out]
                    n958 = Power Of X(1:w2297, 2:5.0 ("y")) -> (0:w2295:dbl)
                    n959 = Divide(x=w2300, y=w2295) -> (x/y=w2298:dbl)
                    n960 = Multiply(x=w2291, y=10.0) -> (x*y=w2304:dbl)
                    n961 = Build Array(w2291, 0.0 ("y")) -> (w2312:dbl[])
                    n962 = Greater Than 0?(x=w2291) -> (x > 0?=w2305:bool)
                    n963 = Negate(x=w2298) -> (-x=w2299:dbl)
                    n964 = case shown="True" w2305 {
                      tunnel: [w2319 w2325] -> w2307
                      tunnel: [w2318 w2324] -> w2306
                      tunnel: w2304 -> [w2317 w2323]
                      tunnel: 0.0 ("y") -> [w2314 w2320]
                      tunnel: w2299 -> [w2316 w2321]
                      tunnel: w2298 -> [w2315 w2322]
                      frame True {
                        n965 = Build Array(w2314, w2316) -> (w2319:dbl[])
                        n966 = Build Array(w2317, w2315) -> (w2318:dbl[])
                      }
                      frame False {
                        n967 = Build Array(w2320, w2321) -> (w2324:dbl[])
                        n968 = Build Array(w2323, w2322) -> (w2325:dbl[])
                      }
                    }
                    n969 = Bundle(w2307, w2306) -> (w2311:cluster{dbl[], dbl[]})  [unwired: 1 in]
                  }
                  frame False {
                    n970 = for {
                      tunnel: [w2351] -> w2338 mode=indexing
                      tunnel: w2342 -> [w2352] mode=indexing
                      n971 = Power Of X(1:w2352, 2:3.0 ("y")) -> (0:w2351:dbl)
                    }
                    n972 = Divide(x=w2341, y=w2338) -> (x/y=w2337:dbl[])
                    n973 = call-poly <vilib>:"Mean.vi"("X"=w2337) -> ("mean"=w2330:dbl)  [unwired: 1 out]
                    n974 = Multiply(x=w2330, y=10.0) -> (x*y=w2332:dbl)
                    n975 = Build Array(w2330, 0.0 ("y")) -> (w2340:dbl[])
                    n976 = Greater Than 0?(x=w2330) -> (x > 0?=w2333:bool)
                    n977 = case shown="True" w2333 {
                      tunnel: [w2346 w2350] -> w2335
                      tunnel: [w2345 w2349] -> w2334
                      tunnel: w2332 -> [w2344 w2348]
                      tunnel: 0.0 ("y") -> [w2343 w2347]
                      frame True {
                        n978 = Build Array(w2343, w2343) -> (w2346:dbl[])
                        n979 = Build Array(w2344, w2343) -> (w2345:dbl[])
                      }
                      frame False {
                        n980 = Build Array(w2347, w2347) -> (w2349:dbl[])
                        n981 = Build Array(w2348, w2347) -> (w2350:dbl[])
                      }
                    }
                    n982 = Bundle(w2335, w2334) -> (w2339:cluster{dbl[], dbl[]})  [unwired: 1 in]
                  }
                }
                n983 = vi-ref "V3fit.vi"() -> (w2225:refnum<vi>)
                n984 = Insert Into Array(array=w2223, index=0, new element=1.0 ("new element/subarray")) -> (w2238:dbl[])
                n985 = Insert Into Array(array=w2209, index=0, new element=0.0 ("new element/subarray")) -> (w2201:dbl[])
                n986 = Insert Into Array(array=w2210, index=0, new element=0.0 ("new element/subarray")) -> (w2243:dbl[])
                n987 = Decrement(x=w2262) -> (x-1=w2261:i32)
                n988 = call-poly <vilib>:"Constrained Nonlinear Curve Fit.vi"("Y"=w2201, "f(x,a)"=w2225, "X"=w2243, "Weight"=w2238, "initial parameters"=w2236, "termination"=w2266, "parameter bounds"=w2235) -> ("best nonlinear fit"=w2269:dbl[], "residue"=w2270:dbl)  [unwired: 3 in, 4 out]
                n989 = Subtract(x=w2201, y=w2269) -> (x-y=w2240:dbl[])
                n990 = Multiply(x=w2270, y=w2224) -> (x*y=w2277:dbl)
                n991 = Square Root(x=w2277) -> (sqrt(x)=w2239:dbl)
                n992 = for {
                  tunnel: w2240 -> [w2371] mode=indexing
                  tunnel: w2239 -> [w2372]
                  tunnel: w2243 -> [w2368] mode=indexing
                  tunnel: w2201 -> [w2367] mode=indexing
                  tunnel: [w2366] -> w2241 mode=indexing
                  tunnel: [w2365] -> w2242 mode=indexing
                  tunnel: w2238 -> [w2364] mode=indexing
                  tunnel: [w2363] -> w2237 mode=indexing
                  n993 = Absolute Value(x=w2371) -> (abs(x)=w2370:dbl)
                  n994 = Greater?(x=w2370, y=w2372) -> (0:w2369:bool)
                  n995 = case shown="False" w2369 {
                    tunnel: w2368 -> [w2375 _]
                    tunnel: w2367 -> [w2374 _]
                    tunnel: [w2375 w2376] -> w2366
                    tunnel: [w2374 w2376] -> w2365
                    tunnel: w2364 -> [w2373 _]
                    tunnel: [w2373 w2376] -> w2363
                    frame False {
                    }
                    frame True {
                      w2376 = 0.0
                    }
                  }
                }
                n996 = while {
                  shift-right: [w2359] -> _
                  shift-left: w2241 -> [w2361]
                  shift-right: [w2362] -> _
                  shift-left: w2242 -> [w2360]
                  tunnel: [w2362] -> w2247
                  tunnel: [w2359] -> w2248
                  shift-right: [w2355] -> w2244
                  shift-left: w2237 -> [w2354]
                  stop <- w2357 stop-if-true
                  w2358 = 0
                  n997 = Search 1D Array(1D array=w2360, element=w2358, start index (0)=w2358) -> (index of element=w2356:i32)
                  n998 = Less Than 0?(x=w2356) -> (x < 0?=w2357:bool)
                  n999 = Delete From Array(array=w2361, index=w2356) -> (array with subset deleted=w2359:dbl[])  [unwired: 1 in, 1 out]
                  n1000 = Delete From Array(array=w2354, index=w2356) -> (array with subset deleted=w2355:dbl[])  [unwired: 1 in, 1 out]
                  n1001 = Delete From Array(array=w2360, index=w2356) -> (array with subset deleted=w2362:dbl[])  [unwired: 1 in, 1 out]
                }
                n1002 = Insert Into Array(array=w2247, index=0, new element=0.0 ("new element/subarray")) -> (w2231:dbl[])
                n1003 = Insert Into Array(array=w2244, index=0, new element=1.0 ("new element/subarray")) -> (w2233:dbl[])
                n1004 = Insert Into Array(array=w2248, index=0, new element=0.0 ("new element/subarray")) -> (w2232:dbl[])
                n1005 = Divide(x=w2232, y=w2226) -> (x/y=w2230:dbl[])
                n1006 = Multiply(x=w2231, y=w2227) -> (x*y=w2228:dbl[])
                n1007 = Array Max & Min(array=w2230) -> (max value=w2217:dbl)  [unwired: 3 out]
                n1008 = Divide(x=w2217, y=w2261) -> (x/y=w2263:dbl)
                n1009 = call-poly <vilib>:"Constrained Nonlinear Curve Fit.vi"("Y"=w2231, "f(x,a)"=w2225, "X"=w2232, "Weight"=w2233, "initial parameters"=w2236, "termination"=w2266, "parameter bounds"=w2235) -> ("best fit parameters"=w2255:dbl[])  [unwired: 3 in, 5 out]
                n1010 = for {
                  N: w2262 -> [_]
                  tunnel: w2263 -> [w2382]
                  tunnel: [w2380] -> w2265 mode=indexing
                  i -> [w2381]
                  n1011 = Multiply(x=w2382, y=w2381) -> (x*y=w2380:dbl)
                }
                n1012 = for {
                  tunnel: w2265 -> [w2400] mode=indexing
                  tunnel: [w2401] -> w2254 mode=indexing
                  tunnel: w2255 -> [w2397]
                  tunnel: [w2400] -> w2253 mode=indexing
                  tunnel: w2227 -> [w2394]
                  tunnel: w2226 -> [w2384]
                  tunnel: [w2383] -> w2218
                  w2385 = 0.0
                  n1013 = Index Array(array=w2397, index=0) -> (element=w2396:dbl)
                  n1014 = Index Array(array=w2397, index=1) -> (element=w2395:dbl)
                  n1015 = Multiply(x=w2396, y=w2394) -> (x*y=w2390:dbl)
                  n1016 = Multiply(x=w2395, y=w2394) -> (x*y=w2388:dbl)
                  n1017 = Power Of X(1:w2384, 2:3.0 ("y")) -> (0:w2392:dbl)
                  n1018 = Power Of X(1:w2384, 2:5.0 ("y")) -> (0:w2389:dbl)
                  n1019 = Multiply(x=w2392, y=w2390) -> (x*y=w2386:dbl)
                  n1020 = Multiply(x=w2389, y=w2388) -> (x*y=w2387:dbl)
                  n1021 = Build Array(w2385, w2385, w2385, w2386, w2385, w2387) -> (w2383:dbl[])
                  n1022 = call-poly <vilib>:"Polynomial Evaluation.vi"("P(x)"=w2383, "a"=w2400) -> ("P(a)"=w2401:dbl)  [unwired: 1 out]
                }
                n1023 = for {
                  tunnel: [w2403] -> w2258 mode=indexing
                  tunnel: w2230 -> [w2402] mode=indexing
                  n1024 = Power Of X(1:w2402, 2:3.0 ("y")) -> (0:w2403:dbl)
                }
                n1025 = for {
                  tunnel: [w2378] -> w2264 mode=indexing
                  tunnel: w2253 -> [w2377] mode=indexing
                  n1026 = Power Of X(1:w2377, 2:3.0 ("y")) -> (0:w2378:dbl)
                }
                n1027 = Array Size(array=w2201) -> (size(s)=w2203:i32)
                n1028 = Build Cluster Array(w2258, w2228) -> (w2259:cluster{dbl, dbl}[])
                n1029 = Build Cluster Array(w2264, w2254) -> (w2260:cluster{dbl, "P(a)":dbl}[])
                n1030 = Build Cluster Array(w2230, w2228) -> (w2257:cluster{dbl, dbl}[])
                n1031 = Build Cluster Array(w2253, w2254) -> (w2256:cluster{dbl, "P(a)":dbl}[])
                n1032 = Array Size(array=w2228) -> (size(s)=w2199:i32)
                n1033 = Array Size(array=w2200) -> (size(s)=w2197:i32)
                n1034 = Decrement(x=w2203) -> (x-1=w2194:i32)
                n1035 = Build Cluster Array(w2259, w2260) -> (→"V3 Mag vs. a^3":cluster{cluster{dbl, "P(a)":dbl}[]}[])
                n1036 = Build Cluster Array(w2257, w2256) -> (→"V3 Mag":cluster{cluster{dbl, "P(a)":dbl}[]}[])
                n1037 = Subtract(x=w2203, y=w2199) -> (x-y=w2204:i32)
                n1038 = Subtract(x=w2197, y=w2194) -> (x-y=w2202:i32)
                n1039 = Array Size(array=w2195) -> (size(s)=w2193:i32)
                n1040 = Subtract(x=w2193, y=w2197) -> (x-y=w2196:i32)
                n1041 = Build Array(w2204, w2202, w2196) -> (w2198:i32[])
                n1042 = Index Array(array=w2218, index=3) -> (element=w2221:dbl)
                n1043 = Index Array(array=w2218, index=5) -> (element=w2222:dbl)
              }
              frame #7 {
                w2405 = 0 ("index")
                w2476 = 51
                # "V3 Re"
                # "V33 Re"
                # "V35 Re"
                n1044 = while {
                  shift-right: [w2495] -> _
                  shift-left: w2409 -> [w2497]
                  shift-right: [w2498] -> _
                  shift-left: w2420 -> [w2496]
                  tunnel: [w2498] -> w2413
                  tunnel: [w2495] -> w2419
                  stop <- w2493 stop-if-true
                  w2494 = 0
                  n1045 = Search 1D Array(1D array=w2496, element=w2494, start index (0)=w2494) -> (index of element=w2492:i32)
                  n1046 = Less Than 0?(x=w2492) -> (x < 0?=w2493:bool)
                  n1047 = Delete From Array(array=w2497, index=w2492) -> (array with subset deleted=w2495:dbl[])  [unwired: 1 in, 1 out]
                  n1048 = Delete From Array(array=w2496, index=w2492) -> (array with subset deleted=w2498:dbl[])  [unwired: 1 in, 1 out]
                }
                n1049 = case shown="True" w2421 {
                  tunnel: w2419 -> [w2500 w2504]
                  tunnel: [w2500 w2503] -> w2427
                  tunnel: w2413 -> [w2499 w2502]
                  tunnel: [w2499 w2501] -> w2426
                  frame False {
                  }
                  frame True {
                    n1050 = Reverse 1D Array(array=w2504) -> (reversed array=w2503:dbl[])
                    n1051 = Reverse 1D Array(array=w2502) -> (reversed array=w2501:dbl[])
                  }
                }
                n1052 = Delete From Array(array=w2426, length=w2422, index=w2405) -> (array with subset deleted=w2428:dbl[])  [unwired: 1 out]
                n1053 = Delete From Array(array=w2428) -> (deleted portion=w2430:dbl)  [unwired: 2 in, 1 out]
                n1054 = Absolute Value(x=w2430) -> (abs(x)=w2429:dbl)
                n1055 = expression code="10**floor(log(x))"(w2429) -> (w2425:dbl)
                n1056 = Delete From Array(array=w2427, length=w2422, index=w2405) -> (array with subset deleted=w2424:dbl[])  [unwired: 1 out]
                n1057 = Divide(x=w2425, y=w2444) -> (x/y=w2442:dbl)
                n1058 = Divide(x=w2428, y=w2425) -> (x/y=w2423:dbl[])
                n1059 = case shown="True" w2406 {
                  tunnel: w2424 -> [w2510 w2556]
                  tunnel: w2423 -> [w2527 w2544]
                  tunnel: [w2526 w2555] -> w2450
                  tunnel: [w2525 w2554] -> w2449
                  tunnel: w2448 -> [w2507 _]
                  frame True {
                    n1060 = for {
                      tunnel: [w2540] -> w2524 mode=indexing
                      tunnel: w2510 -> [w2541] mode=indexing
                      tunnel: [w2540] -> w2516
                      n1061 = Power Of X(1:w2541, 2:3.0 ("y")) -> (0:w2540:dbl)
                    }
                    n1062 = Divide(x=w2527, y=w2524) -> (x/y=w2523:dbl[])
                    n1063 = call <vilib>:"Median.vi"("X"=w2523) -> ("median"=w2505:dbl)  [unwired: 1 out]
                    n1064 = Multiply(x=w2505, y=w2516) -> (x*y=w2515:dbl)
                    n1065 = Multiply(x=w2515, y=w2507) -> (x*y=w2514:dbl)
                    n1066 = Delete From Array(array=w2510) -> (deleted portion=w2511:dbl)  [unwired: 2 in, 1 out]
                    n1067 = Power Of X(1:w2511, 2:5.0 ("y")) -> (0:w2509:dbl)
                    n1068 = Divide(x=w2514, y=w2509) -> (x/y=w2512:dbl)
                    n1069 = Multiply(x=w2505, y=10.0) -> (x*y=w2518:dbl)
                    n1070 = Build Array(w2505, 0.0 ("y")) -> (w2526:dbl[])
                    n1071 = Greater Than 0?(x=w2505) -> (x > 0?=w2519:bool)
                    n1072 = Negate(x=w2512) -> (-x=w2513:dbl)
                    n1073 = case shown="True" w2519 {
                      tunnel: [w2533 w2539] -> w2521
                      tunnel: [w2532 w2538] -> w2520
                      tunnel: w2518 -> [w2531 w2537]
                      tunnel: 0.0 ("y") -> [w2528 w2534]
                      tunnel: w2513 -> [w2530 w2535]
                      tunnel: w2512 -> [w2529 w2536]
                      frame True {
                        n1074 = Build Array(w2528, w2530) -> (w2533:dbl[])
                        n1075 = Build Array(w2531, w2529) -> (w2532:dbl[])
                      }
                      frame False {
                        n1076 = Build Array(w2534, w2535) -> (w2538:dbl[])
                        n1077 = Build Array(w2537, w2536) -> (w2539:dbl[])
                      }
                    }
                    n1078 = Bundle(w2521, w2520) -> (w2525:cluster{dbl[], dbl[]})  [unwired: 1 in]
                  }
                  frame False {
                    n1079 = for {
                      tunnel: [w2565] -> w2553 mode=indexing
                      tunnel: w2556 -> [w2566] mode=indexing
                      n1080 = Power Of X(1:w2566, 2:3.0 ("y")) -> (0:w2565:dbl)
                    }
                    n1081 = Divide(x=w2544, y=w2553) -> (x/y=w2543:dbl[])
                    n1082 = call <vilib>:"Median.vi"("X"=w2543) -> ("median"=w2545:dbl)  [unwired: 1 out]
                    n1083 = Multiply(x=w2545, y=10.0) -> (x*y=w2548:dbl)
                    n1084 = Build Array(w2545, 0.0 ("y")) -> (w2555:dbl[])
                    n1085 = Greater Than 0?(x=w2545) -> (x > 0?=w2549:bool)
                    n1086 = case shown="True" w2549 {
                      tunnel: [w2560 w2564] -> w2551
                      tunnel: [w2559 w2563] -> w2550
                      tunnel: w2548 -> [w2558 w2562]
                      tunnel: 0.0 ("y") -> [w2557 w2561]
                      frame True {
                        n1087 = Build Array(w2557, w2557) -> (w2560:dbl[])
                        n1088 = Build Array(w2558, w2557) -> (w2559:dbl[])
                      }
                      frame False {
                        n1089 = Build Array(w2561, w2561) -> (w2563:dbl[])
                        n1090 = Build Array(w2562, w2561) -> (w2564:dbl[])
                      }
                    }
                    n1091 = Bundle(w2551, w2550) -> (w2554:cluster{dbl[], dbl[]})  [unwired: 1 in]
                  }
                }
                n1092 = vi-ref "V3fit.vi"() -> (w2440:refnum<vi>)
                n1093 = Insert Into Array(array=w2438, index=0, new element=1.0 ("new element/subarray")) -> (w2452:dbl[])
                n1094 = Insert Into Array(array=w2423, index=0, new element=0.0 ("new element/subarray")) -> (w2414:dbl[])
                n1095 = Insert Into Array(array=w2424, index=0, new element=0.0 ("new element/subarray")) -> (w2457:dbl[])
                n1096 = Decrement(x=w2476) -> (x-1=w2475:i32)
                n1097 = call-poly <vilib>:"Constrained Nonlinear Curve Fit.vi"("Y"=w2414, "f(x,a)"=w2440, "X"=w2457, "Weight"=w2452, "initial parameters"=w2450, "termination"=w2480, "parameter bounds"=w2449) -> ("best nonlinear fit"=w2483:dbl[], "residue"=w2484:dbl)  [unwired: 3 in, 4 out]
                n1098 = Subtract(x=w2414, y=w2483) -> (x-y=w2454:dbl[])
                n1099 = Multiply(x=w2484, y=w2439) -> (x*y=w2491:dbl)
                n1100 = Square Root(x=w2491) -> (sqrt(x)=w2453:dbl)
                n1101 = for {
                  tunnel: w2454 -> [w2585] mode=indexing
                  tunnel: w2453 -> [w2586]
                  tunnel: w2457 -> [w2582] mode=indexing
                  tunnel: w2414 -> [w2581] mode=indexing
                  tunnel: [w2580] -> w2455 mode=indexing
                  tunnel: [w2579] -> w2456 mode=indexing
                  tunnel: w2452 -> [w2578] mode=indexing
                  tunnel: [w2577] -> w2451 mode=indexing
                  n1102 = Absolute Value(x=w2585) -> (abs(x)=w2584:dbl)
                  n1103 = Greater?(x=w2584, y=w2586) -> (0:w2583:bool)
                  n1104 = case shown="False" w2583 {
                    tunnel: w2582 -> [w2589 _]
                    tunnel: w2581 -> [w2588 _]
                    tunnel: [w2589 w2590] -> w2580
                    tunnel: [w2588 w2590] -> w2579
                    tunnel: w2578 -> [w2587 _]
                    tunnel: [w2587 w2590] -> w2577
                    frame False {
                    }
                    frame True {
                      w2590 = 0.0
                    }
                  }
                }
                n1105 = while {
                  shift-right: [w2573] -> _
                  shift-left: w2455 -> [w2575]
                  shift-right: [w2576] -> _
                  shift-left: w2456 -> [w2574]
                  tunnel: [w2576] -> w2461
                  tunnel: [w2573] -> w2462
                  shift-right: [w2569] -> w2458
                  shift-left: w2451 -> [w2568]
                  stop <- w2571 stop-if-true
                  w2572 = 0
                  n1106 = Search 1D Array(1D array=w2574, element=w2572, start index (0)=w2572) -> (index of element=w2570:i32)
                  n1107 = Less Than 0?(x=w2570) -> (x < 0?=w2571:bool)
                  n1108 = Delete From Array(array=w2575, index=w2570) -> (array with subset deleted=w2573:dbl[])  [unwired: 1 in, 1 out]
                  n1109 = Delete From Array(array=w2568, index=w2570) -> (array with subset deleted=w2569:dbl[])  [unwired: 1 in, 1 out]
                  n1110 = Delete From Array(array=w2574, index=w2570) -> (array with subset deleted=w2576:dbl[])  [unwired: 1 in, 1 out]
                }
                n1111 = Insert Into Array(array=w2461, index=0, new element=0.0 ("new element/subarray")) -> (w2431:dbl[])
                n1112 = Insert Into Array(array=w2458, index=0, new element=1.0 ("new element/subarray")) -> (w2447:dbl[])
                n1113 = Insert Into Array(array=w2462, index=0, new element=0.0 ("new element/subarray")) -> (w2446:dbl[])
                n1114 = Divide(x=w2446, y=w2441) -> (x/y=w2445:dbl[])
                n1115 = Multiply(x=w2431, y=w2442) -> (x*y=w2443:dbl[])
                n1116 = Array Max & Min(array=w2445) -> (max value=w2433:dbl)  [unwired: 3 out]
                n1117 = Divide(x=w2433, y=w2475) -> (x/y=w2477:dbl)
                n1118 = call-poly <vilib>:"Constrained Nonlinear Curve Fit.vi"("Y"=w2431, "f(x,a)"=w2440, "X"=w2446, "Weight"=w2447, "initial parameters"=w2450, "termination"=w2480, "parameter bounds"=w2449) -> ("best fit parameters"=w2469:dbl[])  [unwired: 3 in, 5 out]
                n1119 = for {
                  N: w2476 -> [_]
                  tunnel: w2477 -> [w2596]
                  tunnel: [w2594] -> w2479 mode=indexing
                  i -> [w2595]
                  n1120 = Multiply(x=w2596, y=w2595) -> (x*y=w2594:dbl)
                }
                n1121 = for {
                  tunnel: w2479 -> [w2614] mode=indexing
                  tunnel: [w2615] -> w2468 mode=indexing
                  tunnel: w2469 -> [w2611]
                  tunnel: [w2614] -> w2467 mode=indexing
                  tunnel: w2442 -> [w2608]
                  tunnel: w2441 -> [w2598]
                  tunnel: [w2597] -> w2434
                  w2599 = 0.0
                  n1122 = Index Array(array=w2611, index=0) -> (element=w2610:dbl)
                  n1123 = Index Array(array=w2611, index=1) -> (element=w2609:dbl)
                  n1124 = Multiply(x=w2610, y=w2608) -> (x*y=w2604:dbl)
                  n1125 = Multiply(x=w2609, y=w2608) -> (x*y=w2602:dbl)
                  n1126 = Power Of X(1:w2598, 2:3.0 ("y")) -> (0:w2606:dbl)
                  n1127 = Power Of X(1:w2598, 2:5.0 ("y")) -> (0:w2603:dbl)
                  n1128 = Multiply(x=w2606, y=w2604) -> (x*y=w2601:dbl)
                  n1129 = Multiply(x=w2603, y=w2602) -> (x*y=w2600:dbl)
                  n1130 = Build Array(w2599, w2599, w2599, w2601, w2599, w2600) -> (w2597:dbl[])
                  n1131 = call-poly <vilib>:"Polynomial Evaluation.vi"("P(x)"=w2597, "a"=w2614) -> ("P(a)"=w2615:dbl)  [unwired: 1 out]
                }
                n1132 = for {
                  tunnel: [w2617] -> w2472 mode=indexing
                  tunnel: w2445 -> [w2616] mode=indexing
                  n1133 = Power Of X(1:w2616, 2:3.0 ("y")) -> (0:w2617:dbl)
                }
                n1134 = for {
                  tunnel: [w2592] -> w2478 mode=indexing
                  tunnel: w2467 -> [w2591] mode=indexing
                  n1135 = Power Of X(1:w2591, 2:3.0 ("y")) -> (0:w2592:dbl)
                }
                n1136 = Array Size(array=w2414) -> (size(s)=w2417:i32)
                n1137 = Build Cluster Array(w2472, w2443) -> (w2473:cluster{dbl, dbl}[])
                n1138 = Build Cluster Array(w2478, w2468) -> (w2474:cluster{dbl, "P(a)":dbl}[])
                n1139 = Build Cluster Array(w2445, w2443) -> (w2471:cluster{dbl, dbl}[])
                n1140 = Build Cluster Array(w2467, w2468) -> (w2470:cluster{dbl, "P(a)":dbl}[])
                n1141 = Array Size(array=w2443) -> (size(s)=w2415:i32)
                n1142 = Array Size(array=w2413) -> (size(s)=w2411:i32)
                n1143 = Decrement(x=w2417) -> (x-1=w2408:i32)
                n1144 = Build Cluster Array(w2473, w2474) -> (→"V3 Re vs. a^3":cluster{cluster{dbl, "P(a)":dbl}[]}[])
                n1145 = Build Cluster Array(w2471, w2470) -> (→"V3 Re":cluster{cluster{dbl, "P(a)":dbl}[]}[])
                n1146 = Subtract(x=w2417, y=w2415) -> (x-y=w2418:i32)
                n1147 = Subtract(x=w2411, y=w2408) -> (x-y=w2416:i32)
                n1148 = Array Size(array=w2409) -> (size(s)=w2407:i32)
                n1149 = Subtract(x=w2407, y=w2411) -> (x-y=w2410:i32)
                n1150 = Build Array(w2418, w2416, w2410) -> (w2412:i32[])
                n1151 = Index Array(array=w2434, index=3) -> (element=w2432:dbl)
                n1152 = Index Array(array=w2434, index=5) -> (element=w2437:dbl)
              }
              frame #8 {
                w2619 = 0 ("index")
                w2690 = 51
                # "V35 Im"
                # "V33 Im"
                # "V3 Im"
                n1153 = while {
                  shift-right: [w2715] -> _
                  shift-left: w2623 -> [w2717]
                  shift-right: [w2718] -> _
                  shift-left: w2644 -> [w2716]
                  tunnel: [w2718] -> w2629
                  tunnel: [w2715] -> w2633
                  stop <- w2713 stop-if-true
                  w2714 = 0
                  n1154 = Search 1D Array(1D array=w2716, element=w2714, start index (0)=w2714) -> (index of element=w2712:i32)
                  n1155 = Less Than 0?(x=w2712) -> (x < 0?=w2713:bool)
                  n1156 = Delete From Array(array=w2717, index=w2712) -> (array with subset deleted=w2715:dbl[])  [unwired: 1 in, 1 out]
                  n1157 = Delete From Array(array=w2716, index=w2712) -> (array with subset deleted=w2718:dbl[])  [unwired: 1 in, 1 out]
                }
                n1158 = case shown="True" w2634 {
                  tunnel: w2633 -> [w2707 w2711]
                  tunnel: [w2707 w2710] -> w2640
                  tunnel: w2629 -> [w2706 w2709]
                  tunnel: [w2706 w2708] -> w2639
                  frame False {
                  }
                  frame True {
                    n1159 = Reverse 1D Array(array=w2711) -> (reversed array=w2710:dbl[])
                    n1160 = Reverse 1D Array(array=w2709) -> (reversed array=w2708:dbl[])
                  }
                }
                n1161 = Delete From Array(array=w2639, length=w2635, index=w2619) -> (array with subset deleted=w2641:dbl[])  [unwired: 1 out]
                n1162 = Delete From Array(array=w2641) -> (deleted portion=w2643:dbl)  [unwired: 2 in, 1 out]
                n1163 = Absolute Value(x=w2643) -> (abs(x)=w2642:dbl)
                n1164 = expression code="10**floor(log(x))"(w2642) -> (w2636:dbl)
                n1165 = Delete From Array(array=w2640, length=w2635, index=w2619) -> (array with subset deleted=w2637:dbl[])  [unwired: 1 out]
                n1166 = Divide(x=w2636, y=w2657) -> (x/y=w2655:dbl)
                n1167 = Divide(x=w2641, y=w2636) -> (x/y=w2638:dbl[])
                n1168 = case shown="True" w2620 {
                  tunnel: w2637 -> [w2724 w2770]
                  tunnel: w2638 -> [w2741 w2769]
                  tunnel: [w2740 w2768] -> w2664
                  tunnel: [w2739 w2767] -> w2663
                  tunnel: w2662 -> [w2721 _]
                  frame True {
                    n1169 = for {
                      tunnel: [w2754] -> w2738 mode=indexing
                      tunnel: w2724 -> [w2755] mode=indexing
                      tunnel: [w2754] -> w2730
                      n1170 = Power Of X(1:w2755, 2:3.0 ("y")) -> (0:w2754:dbl)
                    }
                    n1171 = Divide(x=w2741, y=w2738) -> (x/y=w2737:dbl[])
                    n1172 = call <vilib>:"Median.vi"("X"=w2737) -> ("median"=w2719:dbl)  [unwired: 1 out]
                    n1173 = Multiply(x=w2719, y=w2730) -> (x*y=w2729:dbl)
                    n1174 = Multiply(x=w2729, y=w2721) -> (x*y=w2728:dbl)
                    n1175 = Delete From Array(array=w2724) -> (deleted portion=w2725:dbl)  [unwired: 2 in, 1 out]
                    n1176 = Power Of X(1:w2725, 2:5.0 ("y")) -> (0:w2723:dbl)
                    n1177 = Divide(x=w2728, y=w2723) -> (x/y=w2726:dbl)
                    n1178 = Multiply(x=w2719, y=10.0) -> (x*y=w2732:dbl)
                    n1179 = Build Array(w2719, 0.0 ("y")) -> (w2740:dbl[])
                    n1180 = Greater Than 0?(x=w2719) -> (x > 0?=w2733:bool)
                    n1181 = Negate(x=w2726) -> (-x=w2727:dbl)
                    n1182 = case shown="True" w2733 {
                      tunnel: [w2747 w2753] -> w2735
                      tunnel: [w2746 w2752] -> w2734
                      tunnel: w2732 -> [w2745 w2751]
                      tunnel: 0.0 ("y") -> [w2742 w2748]
                      tunnel: w2727 -> [w2744 w2749]
                      tunnel: w2726 -> [w2743 w2750]
                      frame True {
                        n1183 = Build Array(w2742, w2744) -> (w2747:dbl[])
                        n1184 = Build Array(w2745, w2743) -> (w2746:dbl[])
                      }
                      frame False {
                        n1185 = Build Array(w2748, w2749) -> (w2752:dbl[])
                        n1186 = Build Array(w2751, w2750) -> (w2753:dbl[])
                      }
                    }
                    n1187 = Bundle(w2735, w2734) -> (w2739:cluster{dbl[], dbl[]})  [unwired: 1 in]
                  }
                  frame False {
                    n1188 = for {
                      tunnel: [w2779] -> w2766 mode=indexing
                      tunnel: w2770 -> [w2780] mode=indexing
                      n1189 = Power Of X(1:w2780, 2:3.0 ("y")) -> (0:w2779:dbl)
                    }
                    n1190 = Divide(x=w2769, y=w2766) -> (x/y=w2765:dbl[])
                    n1191 = call <vilib>:"Median.vi"("X"=w2765) -> ("median"=w2758:dbl)  [unwired: 1 out]
                    n1192 = Multiply(x=w2758, y=10.0) -> (x*y=w2760:dbl)
                    n1193 = Build Array(w2758, 0.0 ("y")) -> (w2768:dbl[])
                    n1194 = Greater Than 0?(x=w2758) -> (x > 0?=w2761:bool)
                    n1195 = case shown="True" w2761 {
                      tunnel: [w2774 w2778] -> w2763
                      tunnel: [w2773 w2777] -> w2762
                      tunnel: w2760 -> [w2772 w2776]
                      tunnel: 0.0 ("y") -> [w2771 w2775]
                      frame True {
                        n1196 = Build Array(w2771, w2771) -> (w2774:dbl[])
                        n1197 = Build Array(w2772, w2771) -> (w2773:dbl[])
                      }
                      frame False {
                        n1198 = Build Array(w2775, w2775) -> (w2777:dbl[])
                        n1199 = Build Array(w2776, w2775) -> (w2778:dbl[])
                      }
                    }
                    n1200 = Bundle(w2763, w2762) -> (w2767:cluster{dbl[], dbl[]})  [unwired: 1 in]
                  }
                }
                n1201 = vi-ref "V3fit.vi"() -> (w2653:refnum<vi>)
                n1202 = Insert Into Array(array=w2651, index=0, new element=1.0 ("new element/subarray")) -> (w2666:dbl[])
                n1203 = Insert Into Array(array=w2638, index=0, new element=0.0 ("new element/subarray")) -> (w2628:dbl[])
                n1204 = Insert Into Array(array=w2637, index=0, new element=0.0 ("new element/subarray")) -> (w2671:dbl[])
                n1205 = Decrement(x=w2690) -> (x-1=w2689:i32)
                n1206 = call-poly <vilib>:"Constrained Nonlinear Curve Fit.vi"("Y"=w2628, "f(x,a)"=w2653, "X"=w2671, "Weight"=w2666, "initial parameters"=w2664, "termination"=w2694, "parameter bounds"=w2663) -> ("best nonlinear fit"=w2697:dbl[], "residue"=w2698:dbl)  [unwired: 3 in, 4 out]
                n1207 = Subtract(x=w2628, y=w2697) -> (x-y=w2668:dbl[])
                n1208 = Multiply(x=w2698, y=w2652) -> (x*y=w2705:dbl)
                n1209 = Square Root(x=w2705) -> (sqrt(x)=w2667:dbl)
                n1210 = for {
                  tunnel: w2668 -> [w2799] mode=indexing
                  tunnel: w2667 -> [w2800]
                  tunnel: w2671 -> [w2796] mode=indexing
                  tunnel: w2628 -> [w2795] mode=indexing
                  tunnel: [w2794] -> w2669 mode=indexing
                  tunnel: [w2793] -> w2670 mode=indexing
                  tunnel: w2666 -> [w2792] mode=indexing
                  tunnel: [w2791] -> w2665 mode=indexing
                  n1211 = Absolute Value(x=w2799) -> (abs(x)=w2798:dbl)
                  n1212 = Greater?(x=w2798, y=w2800) -> (0:w2797:bool)
                  n1213 = case shown="False" w2797 {
                    tunnel: w2796 -> [w2803 _]
                    tunnel: w2795 -> [w2802 _]
                    tunnel: [w2803 w2804] -> w2794
                    tunnel: [w2802 w2804] -> w2793
                    tunnel: w2792 -> [w2801 _]
                    tunnel: [w2801 w2804] -> w2791
                    frame False {
                    }
                    frame True {
                      w2804 = 0.0
                    }
                  }
                }
                n1214 = while {
                  shift-right: [w2787] -> _
                  shift-left: w2669 -> [w2789]
                  shift-right: [w2790] -> _
                  shift-left: w2670 -> [w2788]
                  tunnel: [w2790] -> w2675
                  tunnel: [w2787] -> w2676
                  shift-right: [w2783] -> w2672
                  shift-left: w2665 -> [w2782]
                  stop <- w2785 stop-if-true
                  w2786 = 0
                  n1215 = Search 1D Array(1D array=w2788, element=w2786, start index (0)=w2786) -> (index of element=w2784:i32)
                  n1216 = Less Than 0?(x=w2784) -> (x < 0?=w2785:bool)
                  n1217 = Delete From Array(array=w2789, index=w2784) -> (array with subset deleted=w2787:dbl[])  [unwired: 1 in, 1 out]
                  n1218 = Delete From Array(array=w2782, index=w2784) -> (array with subset deleted=w2783:dbl[])  [unwired: 1 in, 1 out]
                  n1219 = Delete From Array(array=w2788, index=w2784) -> (array with subset deleted=w2790:dbl[])  [unwired: 1 in, 1 out]
                }
                n1220 = Insert Into Array(array=w2675, index=0, new element=0.0 ("new element/subarray")) -> (w2659:dbl[])
                n1221 = Insert Into Array(array=w2672, index=0, new element=1.0 ("new element/subarray")) -> (w2661:dbl[])
                n1222 = Insert Into Array(array=w2676, index=0, new element=0.0 ("new element/subarray")) -> (w2660:dbl[])
                n1223 = Divide(x=w2660, y=w2654) -> (x/y=w2658:dbl[])
                n1224 = Multiply(x=w2659, y=w2655) -> (x*y=w2656:dbl[])
                n1225 = Array Max & Min(array=w2658) -> (max value=w2646:dbl)  [unwired: 3 out]
                n1226 = Divide(x=w2646, y=w2689) -> (x/y=w2691:dbl)
                n1227 = call-poly <vilib>:"Constrained Nonlinear Curve Fit.vi"("Y"=w2659, "f(x,a)"=w2653, "X"=w2660, "Weight"=w2661, "initial parameters"=w2664, "termination"=w2694, "parameter bounds"=w2663) -> ("best fit parameters"=w2683:dbl[])  [unwired: 3 in, 5 out]
                n1228 = for {
                  N: w2690 -> [_]
                  tunnel: w2691 -> [w2810]
                  tunnel: [w2808] -> w2693 mode=indexing
                  i -> [w2809]
                  n1229 = Multiply(x=w2810, y=w2809) -> (x*y=w2808:dbl)
                }
                n1230 = for {
                  tunnel: w2693 -> [w2828] mode=indexing
                  tunnel: [w2829] -> w2682 mode=indexing
                  tunnel: w2683 -> [w2825]
                  tunnel: [w2828] -> w2681 mode=indexing
                  tunnel: w2655 -> [w2822]
                  tunnel: w2654 -> [w2812]
                  tunnel: [w2811] -> w2647
                  w2813 = 0.0
                  n1231 = Index Array(array=w2825, index=0) -> (element=w2824:dbl)
                  n1232 = Index Array(array=w2825, index=1) -> (element=w2823:dbl)
                  n1233 = Multiply(x=w2824, y=w2822) -> (x*y=w2818:dbl)
                  n1234 = Multiply(x=w2823, y=w2822) -> (x*y=w2816:dbl)
                  n1235 = Power Of X(1:w2812, 2:3.0 ("y")) -> (0:w2820:dbl)
                  n1236 = Power Of X(1:w2812, 2:5.0 ("y")) -> (0:w2817:dbl)
                  n1237 = Multiply(x=w2820, y=w2818) -> (x*y=w2815:dbl)
                  n1238 = Multiply(x=w2817, y=w2816) -> (x*y=w2814:dbl)
                  n1239 = Build Array(w2813, w2813, w2813, w2815, w2813, w2814) -> (w2811:dbl[])
                  n1240 = call-poly <vilib>:"Polynomial Evaluation.vi"("P(x)"=w2811, "a"=w2828) -> ("P(a)"=w2829:dbl)  [unwired: 1 out]
                }
                n1241 = for {
                  tunnel: [w2831] -> w2686 mode=indexing
                  tunnel: w2658 -> [w2830] mode=indexing
                  n1242 = Power Of X(1:w2830, 2:3.0 ("y")) -> (0:w2831:dbl)
                }
                n1243 = for {
                  tunnel: [w2806] -> w2692 mode=indexing
                  tunnel: w2681 -> [w2805] mode=indexing
                  n1244 = Power Of X(1:w2805, 2:3.0 ("y")) -> (0:w2806:dbl)
                }
                n1245 = Array Size(array=w2628) -> (size(s)=w2631:i32)
                n1246 = Build Cluster Array(w2686, w2656) -> (w2687:cluster{dbl, dbl}[])
                n1247 = Build Cluster Array(w2692, w2682) -> (w2688:cluster{dbl, "P(a)":dbl}[])
                n1248 = Build Cluster Array(w2658, w2656) -> (w2685:cluster{dbl, dbl}[])
                n1249 = Build Cluster Array(w2681, w2682) -> (w2684:cluster{dbl, "P(a)":dbl}[])
                n1250 = Array Size(array=w2656) -> (size(s)=w2627:i32)
                n1251 = Array Size(array=w2629) -> (size(s)=w2625:i32)
                n1252 = Decrement(x=w2631) -> (x-1=w2622:i32)
                n1253 = Build Cluster Array(w2687, w2688) -> (→"V3 Im vs. a^3":cluster{cluster{dbl, "P(a)":dbl}[]}[])
                n1254 = Build Cluster Array(w2685, w2684) -> (→"V3 Im":cluster{cluster{dbl, "P(a)":dbl}[]}[])
                n1255 = Subtract(x=w2631, y=w2627) -> (x-y=w2632:i32)
                n1256 = Subtract(x=w2625, y=w2622) -> (x-y=w2630:i32)
                n1257 = Array Size(array=w2623) -> (size(s)=w2621:i32)
                n1258 = Subtract(x=w2621, y=w2625) -> (x-y=w2624:i32)
                n1259 = Build Array(w2632, w2630, w2624) -> (w2626:i32[])
                n1260 = Index Array(array=w2647, index=3) -> (element=w2645:dbl)
                n1261 = Index Array(array=w2647, index=5) -> (element=w2650:dbl)
              }
              frame #9 {
                w2872 = 51
                # "V4 Mag"
                # "V44 Mag"
                n1262 = for {
                  tunnel: [w2966] -> w2904 mode=indexing
                  tunnel: w2836 -> [w2965] mode=indexing
                  tunnel: w2906 -> [w2964]
                  n1263 = Divide(x=w2965, y=w2964) -> (x/y=w2966:dbl)
                }
                n1264 = for {
                  tunnel: [w2963] -> w2903 mode=indexing
                  tunnel: w2878 -> [w2962] mode=indexing
                  tunnel: w2902 -> [w2961]
                  n1265 = Divide(x=w2962, y=w2961) -> (x/y=w2963:dbl)
                }
                n1266 = while {
                  shift-right: [w2951] -> _
                  shift-left: w2904 -> [w2953]
                  shift-right: [w2954] -> _
                  shift-left: w2903 -> [w2952]
                  tunnel: [w2954] -> w2896
                  tunnel: [w2951] -> w2897
                  stop <- w2949 stop-if-true
                  w2950 = 0
                  n1267 = Search 1D Array(1D array=w2952, element=w2950, start index (0)=w2950) -> (index of element=w2948:i32)
                  n1268 = Less Than 0?(x=w2948) -> (x < 0?=w2949:bool)
                  n1269 = Delete From Array(array=w2953, index=w2948) -> (array with subset deleted=w2951:dbl[])  [unwired: 1 in, 1 out]
                  n1270 = Delete From Array(array=w2952, index=w2948) -> (array with subset deleted=w2954:dbl[])  [unwired: 1 in, 1 out]
                }
                n1271 = case shown="True" w2895 {
                  tunnel: [w2955 w2957] -> w2889
                  tunnel: w2896 -> [w2955 w2956]
                  frame False {
                  }
                  frame True {
                    n1272 = Reverse 1D Array(array=w2956) -> (reversed array=w2957:dbl[])
                  }
                }
                n1273 = case shown="True" w2895 {
                  tunnel: w2897 -> [w2958 w2960]
                  tunnel: [w2958 w2959] -> w2890
                  frame False {
                  }
                  frame True {
                    n1274 = Reverse 1D Array(array=w2960) -> (reversed array=w2959:dbl[])
                  }
                }
                n1275 = for {
                  tunnel: [w2946] -> w2882 mode=indexing
                  tunnel: w2890 -> [w2945] mode=indexing
                  n1276 = Power Of X(1:w2945, 2:4.0 ("y")) -> (0:w2946:dbl)
                }
                n1277 = Divide(x=w2889, y=w2882) -> (x/y=w2883:dbl[])
                n1278 = call-poly <vilib>:"Mean.vi"("X"=w2883) -> ("mean"=w2881:dbl)  [unwired: 1 out]
                n1279 = Build Array(w2881) -> (w2888:dbl[])
                n1280 = Insert Into Array(array=w2877, index=0, new element=1.0 ("new element/subarray")) -> (w2843:dbl[])
                n1281 = Insert Into Array(array=w2889, index=0, new element=0.0 ("new element/subarray")) -> (w2846:dbl[])
                n1282 = Insert Into Array(array=w2890, index=0, new element=0.0 ("new element/subarray")) -> (w2847:dbl[])
                n1283 = vi-ref "V4fit.vi"() -> (w2884:refnum<vi>)
                n1284 = call-poly <vilib>:"Constrained Nonlinear Curve Fit.vi"("Y"=w2846, "f(x,a)"=w2884, "X"=w2847, "Weight"=w2843, "initial parameters"=w2888, "termination"=w2885) -> ("best nonlinear fit"=w2891:dbl[], "residue"=w2892:dbl)  [unwired: 4 in, 4 out]
                n1285 = Subtract(x=w2846, y=w2891) -> (x-y=w2844:dbl[])
                n1286 = Multiply(x=w2892, y=w2876) -> (x*y=w2905:dbl)
                n1287 = Square Root(x=w2905) -> (sqrt(x)=w2845:dbl)
                n1288 = Decrement(x=w2872) -> (x-1=w2871:i32)
                n1289 = for {
                  tunnel: w2844 -> [w2924] mode=indexing
                  tunnel: w2845 -> [w2925]
                  tunnel: w2847 -> [w2921] mode=indexing
                  tunnel: w2846 -> [w2920] mode=indexing
                  tunnel: [w2919] -> w2848 mode=indexing
                  tunnel: [w2918] -> w2849 mode=indexing
                  tunnel: w2843 -> [w2917] mode=indexing
                  tunnel: [w2916] -> w2842 mode=indexing
                  n1290 = Absolute Value(x=w2924) -> (abs(x)=w2923:dbl)
                  n1291 = Greater?(x=w2923, y=w2925) -> (0:w2922:bool)
                  n1292 = case shown="False" w2922 {
                    tunnel: w2921 -> [w2928 _]
                    tunnel: w2920 -> [w2927 _]
                    tunnel: [w2928 w2929] -> w2919
                    tunnel: [w2927 w2929] -> w2918
                    tunnel: w2917 -> [w2926 _]
                    tunnel: [w2926 w2929] -> w2916
                    frame False {
                    }
                    frame True {
                      w2929 = 0.0
                    }
                  }
                }
                n1293 = while {
                  shift-right: [w2912] -> _
                  shift-left: w2848 -> [w2914]
                  shift-right: [w2915] -> _
                  shift-left: w2849 -> [w2913]
                  tunnel: [w2915] -> w2855
                  tunnel: [w2912] -> w2856
                  shift-right: [w2908] -> w2852
                  shift-left: w2842 -> [w2907]
                  stop <- w2910 stop-if-true
                  w2911 = 0
                  n1294 = Search 1D Array(1D array=w2913, element=w2911, start index (0)=w2911) -> (index of element=w2909:i32)
                  n1295 = Less Than 0?(x=w2909) -> (x < 0?=w2910:bool)
                  n1296 = Delete From Array(array=w2914, index=w2909) -> (array with subset deleted=w2912:dbl[])  [unwired: 1 in, 1 out]
                  n1297 = Delete From Array(array=w2907, index=w2909) -> (array with subset deleted=w2908:dbl[])  [unwired: 1 in, 1 out]
                  n1298 = Delete From Array(array=w2913, index=w2909) -> (array with subset deleted=w2915:dbl[])  [unwired: 1 in, 1 out]
                }
                n1299 = Insert Into Array(array=w2855, index=0, new element=0.0 ("new element/subarray")) -> (w2851:dbl[])
                n1300 = Insert Into Array(array=w2852, index=0, new element=1.0 ("new element/subarray")) -> (w2850:dbl[])
                n1301 = Insert Into Array(array=w2856, index=0, new element=0.0 ("new element/subarray")) -> (w2841:dbl[])
                n1302 = call-poly <vilib>:"Constrained Nonlinear Curve Fit.vi"("Y"=w2851, "f(x,a)"=w2884, "X"=w2841, "Weight"=w2850, "initial parameters"=w2888, "termination"=w2885) -> ("best fit parameters"=w2865:dbl[])  [unwired: 4 in, 5 out]
                n1303 = for {
                  tunnel: [w2943] -> w2868 mode=indexing
                  tunnel: w2841 -> [w2942] mode=indexing
                  n1304 = Power Of X(1:w2942, 2:4.0 ("y")) -> (0:w2943:dbl)
                }
                n1305 = Array Max & Min(array=w2841) -> (max value=w2840:dbl)  [unwired: 3 out]
                n1306 = Divide(x=w2840, y=w2871) -> (x/y=w2873:dbl)
                n1307 = for {
                  N: w2872 -> [_]
                  tunnel: w2873 -> [w2935]
                  tunnel: [w2933] -> w2875 mode=indexing
                  i -> [w2934]
                  n1308 = Multiply(x=w2935, y=w2934) -> (x*y=w2933:dbl)
                }
                n1309 = for {
                  tunnel: w2875 -> [w2938] mode=indexing
                  tunnel: [w2940] -> w2862 mode=indexing
                  tunnel: w2865 -> [w2939]
                  tunnel: [w2938] -> w2861 mode=indexing
                  n1310 = Insert Into Array(array=w2939, index=0, new element=dbl[] [0.0, 0.0, 0.0, 0.0]) -> (w2936:dbl[])
                  n1311 = call-poly <vilib>:"Polynomial Evaluation.vi"("P(x)"=w2936, "a"=w2938) -> ("P(a)"=w2940:dbl)  [unwired: 1 out]
                }
                n1312 = for {
                  tunnel: [w2931] -> w2874 mode=indexing
                  tunnel: w2861 -> [w2930] mode=indexing
                  n1313 = Power Of X(1:w2930, 2:4.0 ("y")) -> (0:w2931:dbl)
                }
                n1314 = Array Size(array=w2851) -> (size(s)=w2837:i32)
                n1315 = Build Cluster Array(w2868, w2851) -> (w2869:cluster{dbl, dbl}[])
                n1316 = Build Cluster Array(w2874, w2862) -> (w2870:cluster{dbl, "P(a)":dbl}[])
                n1317 = Build Cluster Array(w2841, w2851) -> (w2867:cluster{dbl, dbl}[])
                n1318 = Build Cluster Array(w2861, w2862) -> (w2866:cluster{dbl, "P(a)":dbl}[])
                n1319 = Array Size(array=w2846) -> (size(s)=w2838:i32)
                n1320 = Build Cluster Array(w2869, w2870) -> (→"V4 Mag vs. a^4":cluster{cluster{dbl, "P(a)":dbl}[]}[])
                n1321 = Build Cluster Array(w2867, w2866) -> (→"V4 Mag":cluster{cluster{dbl, "P(a)":dbl}[]}[])
                n1322 = Array Size(array=w2836) -> (size(s)=w2839:i32)
                n1323 = Subtract(x=w2838, y=w2837) -> (x-y=w2894:i32)
                n1324 = Increment(x=w2839) -> (x+1=w2835:i32)
                n1325 = Subtract(x=w2835, y=w2838) -> (x-y=w2834:i32)
                n1326 = Index Array(array=w2865, index=0) -> (element=w2880:dbl)
                n1327 = Build Array(w2894, 0, w2834) -> (w2879:i32[])
              }
              frame #10 {
                w3008 = 51
                # "V44 Re"
                # "V4 Re"
                n1328 = for {
                  tunnel: [w3100] -> w3038 mode=indexing
                  tunnel: w2969 -> [w3099] mode=indexing
                  tunnel: w3040 -> [w3098]
                  n1329 = Divide(x=w3099, y=w3098) -> (x/y=w3100:dbl)
                }
                n1330 = for {
                  tunnel: [w3097] -> w3037 mode=indexing
                  tunnel: w3012 -> [w3096] mode=indexing
                  tunnel: w3036 -> [w3095]
                  n1331 = Divide(x=w3096, y=w3095) -> (x/y=w3097:dbl)
                }
                n1332 = while {
                  shift-right: [w3085] -> _
                  shift-left: w3038 -> [w3087]
                  shift-right: [w3088] -> _
                  shift-left: w3037 -> [w3086]
                  tunnel: [w3088] -> w3030
                  tunnel: [w3085] -> w3031
                  stop <- w3083 stop-if-true
                  w3084 = 0
                  n1333 = Search 1D Array(1D array=w3086, element=w3084, start index (0)=w3084) -> (index of element=w3082:i32)
                  n1334 = Less Than 0?(x=w3082) -> (x < 0?=w3083:bool)
                  n1335 = Delete From Array(array=w3087, index=w3082) -> (array with subset deleted=w3085:dbl[])  [unwired: 1 in, 1 out]
                  n1336 = Delete From Array(array=w3086, index=w3082) -> (array with subset deleted=w3088:dbl[])  [unwired: 1 in, 1 out]
                }
                n1337 = case shown="True" w3029 {
                  tunnel: [w3089 w3091] -> w3024
                  tunnel: w3030 -> [w3089 w3090]
                  frame False {
                  }
                  frame True {
                    n1338 = Reverse 1D Array(array=w3090) -> (reversed array=w3091:dbl[])
                  }
                }
                n1339 = case shown="True" w3029 {
                  tunnel: w3031 -> [w3092 w3094]
                  tunnel: [w3092 w3093] -> w3025
                  frame False {
                  }
                  frame True {
                    n1340 = Reverse 1D Array(array=w3094) -> (reversed array=w3093:dbl[])
                  }
                }
                n1341 = for {
                  tunnel: [w3080] -> w3017 mode=indexing
                  tunnel: w3025 -> [w3079] mode=indexing
                  n1342 = Power Of X(1:w3079, 2:4.0 ("y")) -> (0:w3080:dbl)
                }
                n1343 = Divide(x=w3024, y=w3017) -> (x/y=w3018:dbl[])
                n1344 = call-poly <vilib>:"Mean.vi"("X"=w3018) -> ("mean"=w3016:dbl)  [unwired: 1 out]
                n1345 = Build Array(w3016) -> (w3023:dbl[])
                n1346 = Insert Into Array(array=w3014, index=0, new element=1.0 ("new element/subarray")) -> (w2979:dbl[])
                n1347 = Insert Into Array(array=w3024, index=0, new element=0.0 ("new element/subarray")) -> (w2972:dbl[])
                n1348 = Insert Into Array(array=w3025, index=0, new element=0.0 ("new element/subarray")) -> (w2983:dbl[])
                n1349 = vi-ref "V4fit.vi"() -> (w3019:refnum<vi>)
                n1350 = call-poly <vilib>:"Constrained Nonlinear Curve Fit.vi"("Y"=w2972, "f(x,a)"=w3019, "X"=w2983, "Weight"=w2979, "initial parameters"=w3023, "termination"=w3020) -> ("best nonlinear fit"=w3026:dbl[], "residue"=w3027:dbl)  [unwired: 4 in, 4 out]
                n1351 = Subtract(x=w2972, y=w3026) -> (x-y=w2985:dbl[])
                n1352 = Multiply(x=w3027, y=w3013) -> (x*y=w3039:dbl)
                n1353 = Square Root(x=w3039) -> (sqrt(x)=w2984:dbl)
                n1354 = Decrement(x=w3008) -> (x-1=w3007:i32)
                n1355 = for {
                  tunnel: w2985 -> [w3058] mode=indexing
                  tunnel: w2984 -> [w3059]
                  tunnel: w2983 -> [w3055] mode=indexing
                  tunnel: w2972 -> [w3054] mode=indexing
                  tunnel: [w3053] -> w2981 mode=indexing
                  tunnel: [w3052] -> w2982 mode=indexing
                  tunnel: w2979 -> [w3051] mode=indexing
                  tunnel: [w3050] -> w2980 mode=indexing
                  n1356 = Absolute Value(x=w3058) -> (abs(x)=w3057:dbl)
                  n1357 = Greater?(x=w3057, y=w3059) -> (0:w3056:bool)
                  n1358 = case shown="False" w3056 {
                    tunnel: w3055 -> [w3062 _]
                    tunnel: w3054 -> [w3061 _]
                    tunnel: [w3062 w3063] -> w3053
                    tunnel: [w3061 w3063] -> w3052
                    tunnel: w3051 -> [w3060 _]
                    tunnel: [w3060 w3063] -> w3050
                    frame False {
                    }
                    frame True {
                      w3063 = 0.0
                    }
                  }
                }
                n1359 = while {
                  shift-right: [w3046] -> _
                  shift-left: w2981 -> [w3048]
                  shift-right: [w3049] -> _
                  shift-left: w2982 -> [w3047]
                  tunnel: [w3049] -> w2991
                  tunnel: [w3046] -> w2992
                  shift-right: [w3042] -> w2988
                  shift-left: w2980 -> [w3041]
                  stop <- w3044 stop-if-true
                  w3045 = 0
                  n1360 = Search 1D Array(1D array=w3047, element=w3045, start index (0)=w3045) -> (index of element=w3043:i32)
                  n1361 = Less Than 0?(x=w3043) -> (x < 0?=w3044:bool)
                  n1362 = Delete From Array(array=w3048, index=w3043) -> (array with subset deleted=w3046:dbl[])  [unwired: 1 in, 1 out]
                  n1363 = Delete From Array(array=w3041, index=w3043) -> (array with subset deleted=w3042:dbl[])  [unwired: 1 in, 1 out]
                  n1364 = Delete From Array(array=w3047, index=w3043) -> (array with subset deleted=w3049:dbl[])  [unwired: 1 in, 1 out]
                }
                n1365 = Insert Into Array(array=w2991, index=0, new element=0.0 ("new element/subarray")) -> (w2987:dbl[])
                n1366 = Insert Into Array(array=w2988, index=0, new element=1.0 ("new element/subarray")) -> (w2986:dbl[])
                n1367 = Insert Into Array(array=w2992, index=0, new element=0.0 ("new element/subarray")) -> (w2978:dbl[])
                n1368 = call-poly <vilib>:"Constrained Nonlinear Curve Fit.vi"("Y"=w2987, "f(x,a)"=w3019, "X"=w2978, "Weight"=w2986, "initial parameters"=w3023, "termination"=w3020) -> ("best fit parameters"=w3001:dbl[])  [unwired: 4 in, 5 out]
                n1369 = for {
                  tunnel: [w3077] -> w3004 mode=indexing
                  tunnel: w2978 -> [w3076] mode=indexing
                  n1370 = Power Of X(1:w3076, 2:4.0 ("y")) -> (0:w3077:dbl)
                }
                n1371 = Array Max & Min(array=w2978) -> (max value=w2977:dbl)  [unwired: 3 out]
                n1372 = Divide(x=w2977, y=w3007) -> (x/y=w3009:dbl)
                n1373 = for {
                  N: w3008 -> [_]
                  tunnel: w3009 -> [w3069]
                  tunnel: [w3067] -> w3011 mode=indexing
                  i -> [w3068]
                  n1374 = Multiply(x=w3069, y=w3068) -> (x*y=w3067:dbl)
                }
                n1375 = for {
                  tunnel: w3011 -> [w3072] mode=indexing
                  tunnel: [w3074] -> w2998 mode=indexing
                  tunnel: w3001 -> [w3073]
                  tunnel: [w3072] -> w2997 mode=indexing
                  n1376 = Insert Into Array(array=w3073, index=0, new element=dbl[] [0.0, 0.0, 0.0, 0.0]) -> (w3070:dbl[])
                  n1377 = call-poly <vilib>:"Polynomial Evaluation.vi"("P(x)"=w3070, "a"=w3072) -> ("P(a)"=w3074:dbl)  [unwired: 1 out]
                }
                n1378 = for {
                  tunnel: [w3065] -> w3010 mode=indexing
                  tunnel: w2997 -> [w3064] mode=indexing
                  n1379 = Power Of X(1:w3064, 2:4.0 ("y")) -> (0:w3065:dbl)
                }
                n1380 = Array Size(array=w2987) -> (size(s)=w2971:i32)
                n1381 = Build Cluster Array(w3004, w2987) -> (w3005:cluster{dbl, dbl}[])
                n1382 = Build Cluster Array(w3010, w2998) -> (w3006:cluster{dbl, "P(a)":dbl}[])
                n1383 = Build Cluster Array(w2978, w2987) -> (w3003:cluster{dbl, dbl}[])
                n1384 = Build Cluster Array(w2997, w2998) -> (w3002:cluster{dbl, "P(a)":dbl}[])
                n1385 = Array Size(array=w2972) -> (size(s)=w2974:i32)
                n1386 = Build Cluster Array(w3005, w3006) -> (→"V4 Re vs. a^4":cluster{cluster{dbl, "P(a)":dbl}[]}[])
                n1387 = Build Cluster Array(w3003, w3002) -> (→"V4 Re":cluster{cluster{dbl, "P(a)":dbl}[]}[])
                n1388 = Array Size(array=w2969) -> (size(s)=w2975:i32)
                n1389 = Subtract(x=w2974, y=w2971) -> (x-y=w2976:i32)
                n1390 = Increment(x=w2975) -> (x+1=w2973:i32)
                n1391 = Subtract(x=w2973, y=w2974) -> (x-y=w2967:i32)
                n1392 = Index Array(array=w3001, index=0) -> (element=w3015:dbl)
                n1393 = Build Array(w2976, 0, w2967) -> (w2970:i32[])
              }
              frame #11 {
                w3142 = 51
                # "V4 Im"
                # "V44 Im"
                n1394 = for {
                  tunnel: [w3234] -> w3172 mode=indexing
                  tunnel: w3104 -> [w3233] mode=indexing
                  tunnel: w3174 -> [w3232]
                  n1395 = Divide(x=w3233, y=w3232) -> (x/y=w3234:dbl)
                }
                n1396 = for {
                  tunnel: [w3231] -> w3171 mode=indexing
                  tunnel: w3146 -> [w3230] mode=indexing
                  tunnel: w3170 -> [w3229]
                  n1397 = Divide(x=w3230, y=w3229) -> (x/y=w3231:dbl)
                }
                n1398 = while {
                  shift-right: [w3219] -> _
                  shift-left: w3172 -> [w3221]
                  shift-right: [w3222] -> _
                  shift-left: w3171 -> [w3220]
                  tunnel: [w3222] -> w3164
                  tunnel: [w3219] -> w3165
                  stop <- w3217 stop-if-true
                  w3218 = 0
                  n1399 = Search 1D Array(1D array=w3220, element=w3218, start index (0)=w3218) -> (index of element=w3216:i32)
                  n1400 = Less Than 0?(x=w3216) -> (x < 0?=w3217:bool)
                  n1401 = Delete From Array(array=w3221, index=w3216) -> (array with subset deleted=w3219:dbl[])  [unwired: 1 in, 1 out]
                  n1402 = Delete From Array(array=w3220, index=w3216) -> (array with subset deleted=w3222:dbl[])  [unwired: 1 in, 1 out]
                }
                n1403 = case shown="True" w3163 {
                  tunnel: [w3223 w3225] -> w3158
                  tunnel: w3164 -> [w3223 w3224]
                  frame False {
                  }
                  frame True {
                    n1404 = Reverse 1D Array(array=w3224) -> (reversed array=w3225:dbl[])
                  }
                }
                n1405 = case shown="True" w3163 {
                  tunnel: w3165 -> [w3226 w3228]
                  tunnel: [w3226 w3227] -> w3159
                  frame False {
                  }
                  frame True {
                    n1406 = Reverse 1D Array(array=w3228) -> (reversed array=w3227:dbl[])
                  }
                }
                n1407 = for {
                  tunnel: [w3214] -> w3151 mode=indexing
                  tunnel: w3159 -> [w3213] mode=indexing
                  n1408 = Power Of X(1:w3213, 2:4.0 ("y")) -> (0:w3214:dbl)
                }
                n1409 = Divide(x=w3158, y=w3151) -> (x/y=w3152:dbl[])
                n1410 = call-poly <vilib>:"Mean.vi"("X"=w3152) -> ("mean"=w3150:dbl)  [unwired: 1 out]
                n1411 = Build Array(w3150) -> (w3157:dbl[])
                n1412 = Insert Into Array(array=w3147, index=0, new element=1.0 ("new element/subarray")) -> (w3113:dbl[])
                n1413 = Insert Into Array(array=w3158, index=0, new element=0.0 ("new element/subarray")) -> (w3105:dbl[])
                n1414 = Insert Into Array(array=w3159, index=0, new element=0.0 ("new element/subarray")) -> (w3117:dbl[])
                n1415 = vi-ref "V4fit.vi"() -> (w3153:refnum<vi>)
                n1416 = call-poly <vilib>:"Constrained Nonlinear Curve Fit.vi"("Y"=w3105, "f(x,a)"=w3153, "X"=w3117, "Weight"=w3113, "initial parameters"=w3157, "termination"=w3154) -> ("best nonlinear fit"=w3160:dbl[], "residue"=w3161:dbl)  [unwired: 4 in, 4 out]
                n1417 = Subtract(x=w3105, y=w3160) -> (x-y=w3114:dbl[])
                n1418 = Multiply(x=w3161, y=w3149) -> (x*y=w3173:dbl)
                n1419 = Square Root(x=w3173) -> (sqrt(x)=w3115:dbl)
                n1420 = Decrement(x=w3142) -> (x-1=w3141:i32)
                n1421 = for {
                  tunnel: w3114 -> [w3192] mode=indexing
                  tunnel: w3115 -> [w3193]
                  tunnel: w3117 -> [w3189] mode=indexing
                  tunnel: w3105 -> [w3188] mode=indexing
                  tunnel: [w3187] -> w3118 mode=indexing
                  tunnel: [w3186] -> w3119 mode=indexing
                  tunnel: w3113 -> [w3185] mode=indexing
                  tunnel: [w3184] -> w3116 mode=indexing
                  n1422 = Absolute Value(x=w3192) -> (abs(x)=w3191:dbl)
                  n1423 = Greater?(x=w3191, y=w3193) -> (0:w3190:bool)
                  n1424 = case shown="False" w3190 {
                    tunnel: w3189 -> [w3196 _]
                    tunnel: w3188 -> [w3195 _]
                    tunnel: [w3196 w3197] -> w3187
                    tunnel: [w3195 w3197] -> w3186
                    tunnel: w3185 -> [w3194 _]
                    tunnel: [w3194 w3197] -> w3184
                    frame False {
                    }
                    frame True {
                      w3197 = 0.0
                    }
                  }
                }
                n1425 = while {
                  shift-right: [w3180] -> _
                  shift-left: w3118 -> [w3182]
                  shift-right: [w3183] -> _
                  shift-left: w3119 -> [w3181]
                  tunnel: [w3183] -> w3125
                  tunnel: [w3180] -> w3126
                  shift-right: [w3176] -> w3122
                  shift-left: w3116 -> [w3175]
                  stop <- w3178 stop-if-true
                  w3179 = 0
                  n1426 = Search 1D Array(1D array=w3181, element=w3179, start index (0)=w3179) -> (index of element=w3177:i32)
                  n1427 = Less Than 0?(x=w3177) -> (x < 0?=w3178:bool)
                  n1428 = Delete From Array(array=w3182, index=w3177) -> (array with subset deleted=w3180:dbl[])  [unwired: 1 in, 1 out]
                  n1429 = Delete From Array(array=w3175, index=w3177) -> (array with subset deleted=w3176:dbl[])  [unwired: 1 in, 1 out]
                  n1430 = Delete From Array(array=w3181, index=w3177) -> (array with subset deleted=w3183:dbl[])  [unwired: 1 in, 1 out]
                }
                n1431 = Insert Into Array(array=w3125, index=0, new element=0.0 ("new element/subarray")) -> (w3121:dbl[])
                n1432 = Insert Into Array(array=w3122, index=0, new element=1.0 ("new element/subarray")) -> (w3120:dbl[])
                n1433 = Insert Into Array(array=w3126, index=0, new element=0.0 ("new element/subarray")) -> (w3112:dbl[])
                n1434 = call-poly <vilib>:"Constrained Nonlinear Curve Fit.vi"("Y"=w3121, "f(x,a)"=w3153, "X"=w3112, "Weight"=w3120, "initial parameters"=w3157, "termination"=w3154) -> ("best fit parameters"=w3135:dbl[])  [unwired: 4 in, 5 out]
                n1435 = for {
                  tunnel: [w3211] -> w3138 mode=indexing
                  tunnel: w3112 -> [w3210] mode=indexing
                  n1436 = Power Of X(1:w3210, 2:4.0 ("y")) -> (0:w3211:dbl)
                }
                n1437 = Array Max & Min(array=w3112) -> (max value=w3111:dbl)  [unwired: 3 out]
                n1438 = Divide(x=w3111, y=w3141) -> (x/y=w3143:dbl)
                n1439 = for {
                  N: w3142 -> [_]
                  tunnel: w3143 -> [w3203]
                  tunnel: [w3201] -> w3145 mode=indexing
                  i -> [w3202]
                  n1440 = Multiply(x=w3203, y=w3202) -> (x*y=w3201:dbl)
                }
                n1441 = for {
                  tunnel: w3145 -> [w3206] mode=indexing
                  tunnel: [w3208] -> w3132 mode=indexing
                  tunnel: w3135 -> [w3207]
                  tunnel: [w3206] -> w3131 mode=indexing
                  n1442 = Insert Into Array(array=w3207, index=0, new element=dbl[] [0.0, 0.0, 0.0, 0.0]) -> (w3204:dbl[])
                  n1443 = call-poly <vilib>:"Polynomial Evaluation.vi"("P(x)"=w3204, "a"=w3206) -> ("P(a)"=w3208:dbl)  [unwired: 1 out]
                }
                n1444 = for {
                  tunnel: [w3199] -> w3144 mode=indexing
                  tunnel: w3131 -> [w3198] mode=indexing
                  n1445 = Power Of X(1:w3198, 2:4.0 ("y")) -> (0:w3199:dbl)
                }
                n1446 = Array Size(array=w3121) -> (size(s)=w3106:i32)
                n1447 = Build Cluster Array(w3138, w3121) -> (w3139:cluster{dbl, dbl}[])
                n1448 = Build Cluster Array(w3144, w3132) -> (w3140:cluster{dbl, "P(a)":dbl}[])
                n1449 = Build Cluster Array(w3112, w3121) -> (w3137:cluster{dbl, dbl}[])
                n1450 = Build Cluster Array(w3131, w3132) -> (w3136:cluster{dbl, "P(a)":dbl}[])
                n1451 = Array Size(array=w3105) -> (size(s)=w3108:i32)
                n1452 = Build Cluster Array(w3139, w3140) -> (→"V4 Im vs. a^4":cluster{cluster{dbl, "P(a)":dbl}[]}[])
                n1453 = Build Cluster Array(w3137, w3136) -> (→"V4 Im":cluster{cluster{dbl, "P(a)":dbl}[]}[])
                n1454 = Array Size(array=w3104) -> (size(s)=w3109:i32)
                n1455 = Subtract(x=w3108, y=w3106) -> (x-y=w3110:i32)
                n1456 = Increment(x=w3109) -> (x+1=w3107:i32)
                n1457 = Subtract(x=w3107, y=w3108) -> (x-y=w3102:i32)
                n1458 = Index Array(array=w3135, index=0) -> (element=w3148:dbl)
                n1459 = Build Array(w3110, 0, w3102) -> (w3103:i32[])
              }
              frame #12 {
                w3276 = 51
                # "V55 Mag"
                # "V5 Mag"
                n1460 = for {
                  tunnel: [w3368] -> w3306 mode=indexing
                  tunnel: w3240 -> [w3367] mode=indexing
                  tunnel: w3308 -> [w3366]
                  n1461 = Divide(x=w3367, y=w3366) -> (x/y=w3368:dbl)
                }
                n1462 = for {
                  tunnel: [w3365] -> w3305 mode=indexing
                  tunnel: w3280 -> [w3364] mode=indexing
                  tunnel: w3304 -> [w3363]
                  n1463 = Divide(x=w3364, y=w3363) -> (x/y=w3365:dbl)
                }
                n1464 = while {
                  shift-right: [w3353] -> _
                  shift-left: w3306 -> [w3355]
                  shift-right: [w3356] -> _
                  shift-left: w3305 -> [w3354]
                  tunnel: [w3356] -> w3298
                  tunnel: [w3353] -> w3299
                  stop <- w3351 stop-if-true
                  w3352 = 0
                  n1465 = Search 1D Array(1D array=w3354, element=w3352, start index (0)=w3352) -> (index of element=w3350:i32)
                  n1466 = Less Than 0?(x=w3350) -> (x < 0?=w3351:bool)
                  n1467 = Delete From Array(array=w3355, index=w3350) -> (array with subset deleted=w3353:dbl[])  [unwired: 1 in, 1 out]
                  n1468 = Delete From Array(array=w3354, index=w3350) -> (array with subset deleted=w3356:dbl[])  [unwired: 1 in, 1 out]
                }
                n1469 = case shown="True" w3297 {
                  tunnel: [w3357 w3359] -> w3292
                  tunnel: w3298 -> [w3357 w3358]
                  frame False {
                  }
                  frame True {
                    n1470 = Reverse 1D Array(array=w3358) -> (reversed array=w3359:dbl[])
                  }
                }
                n1471 = case shown="True" w3297 {
                  tunnel: w3299 -> [w3360 w3362]
                  tunnel: [w3360 w3361] -> w3293
                  frame False {
                  }
                  frame True {
                    n1472 = Reverse 1D Array(array=w3362) -> (reversed array=w3361:dbl[])
                  }
                }
                n1473 = for {
                  tunnel: [w3348] -> w3285 mode=indexing
                  tunnel: w3293 -> [w3347] mode=indexing
                  n1474 = Power Of X(1:w3347, 2:5.0 ("y")) -> (0:w3348:dbl)
                }
                n1475 = Divide(x=w3292, y=w3285) -> (x/y=w3286:dbl[])
                n1476 = call-poly <vilib>:"Mean.vi"("X"=w3286) -> ("mean"=w3284:dbl)  [unwired: 1 out]
                n1477 = Build Array(w3284) -> (w3291:dbl[])
                n1478 = Insert Into Array(array=w3282, index=0, new element=1.0 ("new element/subarray")) -> (w3247:dbl[])
                n1479 = Insert Into Array(array=w3292, index=0, new element=0.0 ("new element/subarray")) -> (w3239:dbl[])
                n1480 = Insert Into Array(array=w3293, index=0, new element=0.0 ("new element/subarray")) -> (w3250:dbl[])
                n1481 = vi-ref "V5fit.vi"() -> (w3287:refnum<vi>)
                n1482 = call-poly <vilib>:"Constrained Nonlinear Curve Fit.vi"("Y"=w3239, "f(x,a)"=w3287, "X"=w3250, "Weight"=w3247, "initial parameters"=w3291, "termination"=w3288) -> ("best nonlinear fit"=w3294:dbl[], "residue"=w3295:dbl)  [unwired: 4 in, 4 out]
                n1483 = Subtract(x=w3239, y=w3294) -> (x-y=w3248:dbl[])
                n1484 = Multiply(x=w3295, y=w3283) -> (x*y=w3307:dbl)
                n1485 = Square Root(x=w3307) -> (sqrt(x)=w3249:dbl)
                n1486 = Decrement(x=w3276) -> (x-1=w3275:i32)
                n1487 = for {
                  tunnel: w3248 -> [w3326] mode=indexing
                  tunnel: w3249 -> [w3327]
                  tunnel: w3250 -> [w3323] mode=indexing
                  tunnel: w3239 -> [w3322] mode=indexing
                  tunnel: [w3321] -> w3252 mode=indexing
                  tunnel: [w3320] -> w3253 mode=indexing
                  tunnel: w3247 -> [w3319] mode=indexing
                  tunnel: [w3318] -> w3251 mode=indexing
                  n1488 = Absolute Value(x=w3326) -> (abs(x)=w3325:dbl)
                  n1489 = Greater?(x=w3325, y=w3327) -> (0:w3324:bool)
                  n1490 = case shown="False" w3324 {
                    tunnel: w3323 -> [w3330 _]
                    tunnel: w3322 -> [w3329 _]
                    tunnel: [w3330 w3331] -> w3321
                    tunnel: [w3329 w3331] -> w3320
                    tunnel: w3319 -> [w3328 _]
                    tunnel: [w3328 w3331] -> w3318
                    frame False {
                    }
                    frame True {
                      w3331 = 0.0
                    }
                  }
                }
                n1491 = while {
                  shift-right: [w3314] -> _
                  shift-left: w3252 -> [w3316]
                  shift-right: [w3317] -> _
                  shift-left: w3253 -> [w3315]
                  tunnel: [w3317] -> w3259
                  tunnel: [w3314] -> w3260
                  shift-right: [w3310] -> w3256
                  shift-left: w3251 -> [w3309]
                  stop <- w3312 stop-if-true
                  w3313 = 0
                  n1492 = Search 1D Array(1D array=w3315, element=w3313, start index (0)=w3313) -> (index of element=w3311:i32)
                  n1493 = Less Than 0?(x=w3311) -> (x < 0?=w3312:bool)
                  n1494 = Delete From Array(array=w3316, index=w3311) -> (array with subset deleted=w3314:dbl[])  [unwired: 1 in, 1 out]
                  n1495 = Delete From Array(array=w3309, index=w3311) -> (array with subset deleted=w3310:dbl[])  [unwired: 1 in, 1 out]
                  n1496 = Delete From Array(array=w3315, index=w3311) -> (array with subset deleted=w3317:dbl[])  [unwired: 1 in, 1 out]
                }
                n1497 = Insert Into Array(array=w3259, index=0, new element=0.0 ("new element/subarray")) -> (w3255:dbl[])
                n1498 = Insert Into Array(array=w3256, index=0, new element=1.0 ("new element/subarray")) -> (w3254:dbl[])
                n1499 = Insert Into Array(array=w3260, index=0, new element=0.0 ("new element/subarray")) -> (w3246:dbl[])
                n1500 = call-poly <vilib>:"Constrained Nonlinear Curve Fit.vi"("Y"=w3255, "f(x,a)"=w3287, "X"=w3246, "Weight"=w3254, "initial parameters"=w3291, "termination"=w3288) -> ("best fit parameters"=w3269:dbl[])  [unwired: 4 in, 5 out]
                n1501 = for {
                  tunnel: [w3345] -> w3272 mode=indexing
                  tunnel: w3246 -> [w3344] mode=indexing
                  n1502 = Power Of X(1:w3344, 2:5.0 ("y")) -> (0:w3345:dbl)
                }
                n1503 = Array Max & Min(array=w3246) -> (max value=w3245:dbl)  [unwired: 3 out]
                n1504 = Divide(x=w3245, y=w3275) -> (x/y=w3277:dbl)
                n1505 = for {
                  N: w3276 -> [_]
                  tunnel: w3277 -> [w3337]
                  tunnel: [w3335] -> w3279 mode=indexing
                  i -> [w3336]
                  n1506 = Multiply(x=w3337, y=w3336) -> (x*y=w3335:dbl)
                }
                n1507 = for {
                  tunnel: w3279 -> [w3340] mode=indexing
                  tunnel: [w3342] -> w3266 mode=indexing
                  tunnel: w3269 -> [w3341]
                  tunnel: [w3340] -> w3265 mode=indexing
                  n1508 = Insert Into Array(array=w3341, index=0, new element=dbl[] [0.0, 0.0, 0.0, 0.0, 0.0]) -> (w3338:dbl[])
                  n1509 = call-poly <vilib>:"Polynomial Evaluation.vi"("P(x)"=w3338, "a"=w3340) -> ("P(a)"=w3342:dbl)  [unwired: 1 out]
                }
                n1510 = for {
                  tunnel: [w3333] -> w3278 mode=indexing
                  tunnel: w3265 -> [w3332] mode=indexing
                  n1511 = Power Of X(1:w3332, 2:5.0 ("y")) -> (0:w3333:dbl)
                }
                n1512 = Array Size(array=w3255) -> (size(s)=w3238:i32)
                n1513 = Build Cluster Array(w3272, w3255) -> (w3273:cluster{dbl, dbl}[])
                n1514 = Build Cluster Array(w3278, w3266) -> (w3274:cluster{dbl, "P(a)":dbl}[])
                n1515 = Build Cluster Array(w3246, w3255) -> (w3271:cluster{dbl, dbl}[])
                n1516 = Build Cluster Array(w3265, w3266) -> (w3270:cluster{dbl, "P(a)":dbl}[])
                n1517 = Array Size(array=w3239) -> (size(s)=w3242:i32)
                n1518 = Build Cluster Array(w3273, w3274) -> (→"V5 Mag vs. a^5":cluster{cluster{dbl, "P(a)":dbl}[]}[])
                n1519 = Build Cluster Array(w3271, w3270) -> (→"V5 Mag":cluster{cluster{dbl, "P(a)":dbl}[]}[])
                n1520 = Array Size(array=w3240) -> (size(s)=w3243:i32)
                n1521 = Subtract(x=w3242, y=w3238) -> (x-y=w3244:i32)
                n1522 = Increment(x=w3243) -> (x+1=w3241:i32)
                n1523 = Subtract(x=w3241, y=w3242) -> (x-y=w3236:i32)
                n1524 = Index Array(array=w3269, index=0) -> (element=w3281:dbl)
                n1525 = Build Array(w3244, 0, w3236) -> (w3237:i32[])
              }
              frame #13 {
                w3410 = 51
                # "V55 Re"
                # "V5 Re"
                n1526 = for {
                  tunnel: [w3502] -> w3440 mode=indexing
                  tunnel: w3371 -> [w3501] mode=indexing
                  tunnel: w3442 -> [w3500]
                  n1527 = Divide(x=w3501, y=w3500) -> (x/y=w3502:dbl)
                }
                n1528 = for {
                  tunnel: [w3499] -> w3439 mode=indexing
                  tunnel: w3414 -> [w3498] mode=indexing
                  tunnel: w3438 -> [w3497]
                  n1529 = Divide(x=w3498, y=w3497) -> (x/y=w3499:dbl)
                }
                n1530 = while {
                  shift-right: [w3487] -> _
                  shift-left: w3440 -> [w3489]
                  shift-right: [w3490] -> _
                  shift-left: w3439 -> [w3488]
                  tunnel: [w3490] -> w3432
                  tunnel: [w3487] -> w3433
                  stop <- w3485 stop-if-true
                  w3486 = 0
                  n1531 = Search 1D Array(1D array=w3488, element=w3486, start index (0)=w3486) -> (index of element=w3484:i32)
                  n1532 = Less Than 0?(x=w3484) -> (x < 0?=w3485:bool)
                  n1533 = Delete From Array(array=w3489, index=w3484) -> (array with subset deleted=w3487:dbl[])  [unwired: 1 in, 1 out]
                  n1534 = Delete From Array(array=w3488, index=w3484) -> (array with subset deleted=w3490:dbl[])  [unwired: 1 in, 1 out]
                }
                n1535 = case shown="True" w3431 {
                  tunnel: [w3491 w3493] -> w3426
                  tunnel: w3432 -> [w3491 w3492]
                  frame False {
                  }
                  frame True {
                    n1536 = Reverse 1D Array(array=w3492) -> (reversed array=w3493:dbl[])
                  }
                }
                n1537 = case shown="True" w3431 {
                  tunnel: w3433 -> [w3494 w3496]
                  tunnel: [w3494 w3495] -> w3427
                  frame False {
                  }
                  frame True {
                    n1538 = Reverse 1D Array(array=w3496) -> (reversed array=w3495:dbl[])
                  }
                }
                n1539 = for {
                  tunnel: [w3482] -> w3419 mode=indexing
                  tunnel: w3427 -> [w3481] mode=indexing
                  n1540 = Power Of X(1:w3481, 2:5.0 ("y")) -> (0:w3482:dbl)
                }
                n1541 = Divide(x=w3426, y=w3419) -> (x/y=w3420:dbl[])
                n1542 = call-poly <vilib>:"Mean.vi"("X"=w3420) -> ("mean"=w3418:dbl)  [unwired: 1 out]
                n1543 = Build Array(w3418) -> (w3425:dbl[])
                n1544 = Insert Into Array(array=w3416, index=0, new element=1.0 ("new element/subarray")) -> (w3381:dbl[])
                n1545 = Insert Into Array(array=w3426, index=0, new element=0.0 ("new element/subarray")) -> (w3373:dbl[])
                n1546 = Insert Into Array(array=w3427, index=0, new element=0.0 ("new element/subarray")) -> (w3384:dbl[])
                n1547 = vi-ref "V5fit.vi"() -> (w3421:refnum<vi>)
                n1548 = call-poly <vilib>:"Constrained Nonlinear Curve Fit.vi"("Y"=w3373, "f(x,a)"=w3421, "X"=w3384, "Weight"=w3381, "initial parameters"=w3425, "termination"=w3422) -> ("best nonlinear fit"=w3428:dbl[], "residue"=w3429:dbl)  [unwired: 4 in, 4 out]
                n1549 = Subtract(x=w3373, y=w3428) -> (x-y=w3382:dbl[])
                n1550 = Multiply(x=w3429, y=w3417) -> (x*y=w3441:dbl)
                n1551 = Square Root(x=w3441) -> (sqrt(x)=w3383:dbl)
                n1552 = Decrement(x=w3410) -> (x-1=w3409:i32)
                n1553 = for {
                  tunnel: w3382 -> [w3460] mode=indexing
                  tunnel: w3383 -> [w3461]
                  tunnel: w3384 -> [w3457] mode=indexing
                  tunnel: w3373 -> [w3456] mode=indexing
                  tunnel: [w3455] -> w3386 mode=indexing
                  tunnel: [w3454] -> w3387 mode=indexing
                  tunnel: w3381 -> [w3453] mode=indexing
                  tunnel: [w3452] -> w3385 mode=indexing
                  n1554 = Absolute Value(x=w3460) -> (abs(x)=w3459:dbl)
                  n1555 = Greater?(x=w3459, y=w3461) -> (0:w3458:bool)
                  n1556 = case shown="False" w3458 {
                    tunnel: w3457 -> [w3464 _]
                    tunnel: w3456 -> [w3463 _]
                    tunnel: [w3464 w3465] -> w3455
                    tunnel: [w3463 w3465] -> w3454
                    tunnel: w3453 -> [w3462 _]
                    tunnel: [w3462 w3465] -> w3452
                    frame False {
                    }
                    frame True {
                      w3465 = 0.0
                    }
                  }
                }
                n1557 = while {
                  shift-right: [w3448] -> _
                  shift-left: w3386 -> [w3450]
                  shift-right: [w3451] -> _
                  shift-left: w3387 -> [w3449]
                  tunnel: [w3451] -> w3393
                  tunnel: [w3448] -> w3394
                  shift-right: [w3444] -> w3390
                  shift-left: w3385 -> [w3443]
                  stop <- w3446 stop-if-true
                  w3447 = 0
                  n1558 = Search 1D Array(1D array=w3449, element=w3447, start index (0)=w3447) -> (index of element=w3445:i32)
                  n1559 = Less Than 0?(x=w3445) -> (x < 0?=w3446:bool)
                  n1560 = Delete From Array(array=w3450, index=w3445) -> (array with subset deleted=w3448:dbl[])  [unwired: 1 in, 1 out]
                  n1561 = Delete From Array(array=w3443, index=w3445) -> (array with subset deleted=w3444:dbl[])  [unwired: 1 in, 1 out]
                  n1562 = Delete From Array(array=w3449, index=w3445) -> (array with subset deleted=w3451:dbl[])  [unwired: 1 in, 1 out]
                }
                n1563 = Insert Into Array(array=w3393, index=0, new element=0.0 ("new element/subarray")) -> (w3389:dbl[])
                n1564 = Insert Into Array(array=w3390, index=0, new element=1.0 ("new element/subarray")) -> (w3388:dbl[])
                n1565 = Insert Into Array(array=w3394, index=0, new element=0.0 ("new element/subarray")) -> (w3380:dbl[])
                n1566 = call-poly <vilib>:"Constrained Nonlinear Curve Fit.vi"("Y"=w3389, "f(x,a)"=w3421, "X"=w3380, "Weight"=w3388, "initial parameters"=w3425, "termination"=w3422) -> ("best fit parameters"=w3403:dbl[])  [unwired: 4 in, 5 out]
                n1567 = for {
                  tunnel: [w3479] -> w3406 mode=indexing
                  tunnel: w3380 -> [w3478] mode=indexing
                  n1568 = Power Of X(1:w3478, 2:5.0 ("y")) -> (0:w3479:dbl)
                }
                n1569 = Array Max & Min(array=w3380) -> (max value=w3379:dbl)  [unwired: 3 out]
                n1570 = Divide(x=w3379, y=w3409) -> (x/y=w3411:dbl)
                n1571 = for {
                  N: w3410 -> [_]
                  tunnel: w3411 -> [w3471]
                  tunnel: [w3469] -> w3413 mode=indexing
                  i -> [w3470]
                  n1572 = Multiply(x=w3471, y=w3470) -> (x*y=w3469:dbl)
                }
                n1573 = for {
                  tunnel: w3413 -> [w3474] mode=indexing
                  tunnel: [w3476] -> w3400 mode=indexing
                  tunnel: w3403 -> [w3475]
                  tunnel: [w3474] -> w3399 mode=indexing
                  n1574 = Insert Into Array(array=w3475, index=0, new element=dbl[] [0.0, 0.0, 0.0, 0.0, 0.0]) -> (w3472:dbl[])
                  n1575 = call-poly <vilib>:"Polynomial Evaluation.vi"("P(x)"=w3472, "a"=w3474) -> ("P(a)"=w3476:dbl)  [unwired: 1 out]
                }
                n1576 = for {
                  tunnel: [w3467] -> w3412 mode=indexing
                  tunnel: w3399 -> [w3466] mode=indexing
                  n1577 = Power Of X(1:w3466, 2:5.0 ("y")) -> (0:w3467:dbl)
                }
                n1578 = Array Size(array=w3389) -> (size(s)=w3374:i32)
                n1579 = Build Cluster Array(w3406, w3389) -> (w3407:cluster{dbl, dbl}[])
                n1580 = Build Cluster Array(w3412, w3400) -> (w3408:cluster{dbl, "P(a)":dbl}[])
                n1581 = Build Cluster Array(w3380, w3389) -> (w3405:cluster{dbl, dbl}[])
                n1582 = Build Cluster Array(w3399, w3400) -> (w3404:cluster{dbl, "P(a)":dbl}[])
                n1583 = Array Size(array=w3373) -> (size(s)=w3376:i32)
                n1584 = Build Cluster Array(w3407, w3408) -> (→"V5 Re vs. a^5":cluster{cluster{dbl, "P(a)":dbl}[]}[])
                n1585 = Build Cluster Array(w3405, w3404) -> (→"V5 Re":cluster{cluster{dbl, "P(a)":dbl}[]}[])
                n1586 = Array Size(array=w3371) -> (size(s)=w3377:i32)
                n1587 = Subtract(x=w3376, y=w3374) -> (x-y=w3378:i32)
                n1588 = Increment(x=w3377) -> (x+1=w3375:i32)
                n1589 = Subtract(x=w3375, y=w3376) -> (x-y=w3370:i32)
                n1590 = Index Array(array=w3403, index=0) -> (element=w3415:dbl)
                n1591 = Build Array(w3378, 0, w3370) -> (w3372:i32[])
              }
              frame #14 {
                w3544 = 51
                # "V55 Im"
                # "V5 Im"
                n1592 = for {
                  tunnel: [w3636] -> w3574 mode=indexing
                  tunnel: w3505 -> [w3635] mode=indexing
                  tunnel: w3576 -> [w3634]
                  n1593 = Divide(x=w3635, y=w3634) -> (x/y=w3636:dbl)
                }
                n1594 = for {
                  tunnel: [w3633] -> w3573 mode=indexing
                  tunnel: w3548 -> [w3632] mode=indexing
                  tunnel: w3572 -> [w3631]
                  n1595 = Divide(x=w3632, y=w3631) -> (x/y=w3633:dbl)
                }
                n1596 = while {
                  shift-right: [w3621] -> _
                  shift-left: w3574 -> [w3623]
                  shift-right: [w3624] -> _
                  shift-left: w3573 -> [w3622]
                  tunnel: [w3624] -> w3566
                  tunnel: [w3621] -> w3567
                  stop <- w3619 stop-if-true
                  w3620 = 0
                  n1597 = Search 1D Array(1D array=w3622, element=w3620, start index (0)=w3620) -> (index of element=w3618:i32)
                  n1598 = Less Than 0?(x=w3618) -> (x < 0?=w3619:bool)
                  n1599 = Delete From Array(array=w3623, index=w3618) -> (array with subset deleted=w3621:dbl[])  [unwired: 1 in, 1 out]
                  n1600 = Delete From Array(array=w3622, index=w3618) -> (array with subset deleted=w3624:dbl[])  [unwired: 1 in, 1 out]
                }
                n1601 = case shown="True" w3565 {
                  tunnel: [w3625 w3627] -> w3560
                  tunnel: w3566 -> [w3625 w3626]
                  frame False {
                  }
                  frame True {
                    n1602 = Reverse 1D Array(array=w3626) -> (reversed array=w3627:dbl[])
                  }
                }
                n1603 = case shown="True" w3565 {
                  tunnel: w3567 -> [w3628 w3630]
                  tunnel: [w3628 w3629] -> w3561
                  frame False {
                  }
                  frame True {
                    n1604 = Reverse 1D Array(array=w3630) -> (reversed array=w3629:dbl[])
                  }
                }
                n1605 = for {
                  tunnel: [w3616] -> w3553 mode=indexing
                  tunnel: w3561 -> [w3615] mode=indexing
                  n1606 = Power Of X(1:w3615, 2:5.0 ("y")) -> (0:w3616:dbl)
                }
                n1607 = Divide(x=w3560, y=w3553) -> (x/y=w3554:dbl[])
                n1608 = call-poly <vilib>:"Mean.vi"("X"=w3554) -> ("mean"=w3552:dbl)  [unwired: 1 out]
                n1609 = Build Array(w3552) -> (w3559:dbl[])
                n1610 = Insert Into Array(array=w3550, index=0, new element=1.0 ("new element/subarray")) -> (w3516:dbl[])
                n1611 = Insert Into Array(array=w3560, index=0, new element=0.0 ("new element/subarray")) -> (w3508:dbl[])
                n1612 = Insert Into Array(array=w3561, index=0, new element=0.0 ("new element/subarray")) -> (w3519:dbl[])
                n1613 = vi-ref "V5fit.vi"() -> (w3555:refnum<vi>)
                n1614 = call-poly <vilib>:"Constrained Nonlinear Curve Fit.vi"("Y"=w3508, "f(x,a)"=w3555, "X"=w3519, "Weight"=w3516, "initial parameters"=w3559, "termination"=w3556) -> ("best nonlinear fit"=w3562:dbl[], "residue"=w3563:dbl)  [unwired: 4 in, 4 out]
                n1615 = Subtract(x=w3508, y=w3562) -> (x-y=w3517:dbl[])
                n1616 = Multiply(x=w3563, y=w3551) -> (x*y=w3575:dbl)
                n1617 = Square Root(x=w3575) -> (sqrt(x)=w3518:dbl)
                n1618 = Decrement(x=w3544) -> (x-1=w3543:i32)
                n1619 = for {
                  tunnel: w3517 -> [w3594] mode=indexing
                  tunnel: w3518 -> [w3595]
                  tunnel: w3519 -> [w3591] mode=indexing
                  tunnel: w3508 -> [w3590] mode=indexing
                  tunnel: [w3589] -> w3520 mode=indexing
                  tunnel: [w3588] -> w3521 mode=indexing
                  tunnel: w3516 -> [w3587] mode=indexing
                  tunnel: [w3586] -> w3515 mode=indexing
                  n1620 = Absolute Value(x=w3594) -> (abs(x)=w3593:dbl)
                  n1621 = Greater?(x=w3593, y=w3595) -> (0:w3592:bool)
                  n1622 = case shown="False" w3592 {
                    tunnel: w3591 -> [w3598 _]
                    tunnel: w3590 -> [w3597 _]
                    tunnel: [w3598 w3599] -> w3589
                    tunnel: [w3597 w3599] -> w3588
                    tunnel: w3587 -> [w3596 _]
                    tunnel: [w3596 w3599] -> w3586
                    frame False {
                    }
                    frame True {
                      w3599 = 0.0
                    }
                  }
                }
                n1623 = while {
                  shift-right: [w3582] -> _
                  shift-left: w3520 -> [w3584]
                  shift-right: [w3585] -> _
                  shift-left: w3521 -> [w3583]
                  tunnel: [w3585] -> w3527
                  tunnel: [w3582] -> w3528
                  shift-right: [w3578] -> w3524
                  shift-left: w3515 -> [w3577]
                  stop <- w3580 stop-if-true
                  w3581 = 0
                  n1624 = Search 1D Array(1D array=w3583, element=w3581, start index (0)=w3581) -> (index of element=w3579:i32)
                  n1625 = Less Than 0?(x=w3579) -> (x < 0?=w3580:bool)
                  n1626 = Delete From Array(array=w3584, index=w3579) -> (array with subset deleted=w3582:dbl[])  [unwired: 1 in, 1 out]
                  n1627 = Delete From Array(array=w3577, index=w3579) -> (array with subset deleted=w3578:dbl[])  [unwired: 1 in, 1 out]
                  n1628 = Delete From Array(array=w3583, index=w3579) -> (array with subset deleted=w3585:dbl[])  [unwired: 1 in, 1 out]
                }
                n1629 = Insert Into Array(array=w3527, index=0, new element=0.0 ("new element/subarray")) -> (w3523:dbl[])
                n1630 = Insert Into Array(array=w3524, index=0, new element=1.0 ("new element/subarray")) -> (w3522:dbl[])
                n1631 = Insert Into Array(array=w3528, index=0, new element=0.0 ("new element/subarray")) -> (w3514:dbl[])
                n1632 = call-poly <vilib>:"Constrained Nonlinear Curve Fit.vi"("Y"=w3523, "f(x,a)"=w3555, "X"=w3514, "Weight"=w3522, "initial parameters"=w3559, "termination"=w3556) -> ("best fit parameters"=w3537:dbl[])  [unwired: 4 in, 5 out]
                n1633 = for {
                  tunnel: [w3613] -> w3540 mode=indexing
                  tunnel: w3514 -> [w3612] mode=indexing
                  n1634 = Power Of X(1:w3612, 2:5.0 ("y")) -> (0:w3613:dbl)
                }
                n1635 = Array Max & Min(array=w3514) -> (max value=w3513:dbl)  [unwired: 3 out]
                n1636 = Divide(x=w3513, y=w3543) -> (x/y=w3545:dbl)
                n1637 = for {
                  N: w3544 -> [_]
                  tunnel: w3545 -> [w3605]
                  tunnel: [w3603] -> w3547 mode=indexing
                  i -> [w3604]
                  n1638 = Multiply(x=w3605, y=w3604) -> (x*y=w3603:dbl)
                }
                n1639 = for {
                  tunnel: w3547 -> [w3608] mode=indexing
                  tunnel: [w3610] -> w3534 mode=indexing
                  tunnel: w3537 -> [w3609]
                  tunnel: [w3608] -> w3533 mode=indexing
                  n1640 = Insert Into Array(array=w3609, index=0, new element=dbl[] [0.0, 0.0, 0.0, 0.0, 0.0]) -> (w3606:dbl[])
                  n1641 = call-poly <vilib>:"Polynomial Evaluation.vi"("P(x)"=w3606, "a"=w3608) -> ("P(a)"=w3610:dbl)  [unwired: 1 out]
                }
                n1642 = for {
                  tunnel: [w3601] -> w3546 mode=indexing
                  tunnel: w3533 -> [w3600] mode=indexing
                  n1643 = Power Of X(1:w3600, 2:5.0 ("y")) -> (0:w3601:dbl)
                }
                n1644 = Array Size(array=w3523) -> (size(s)=w3507:i32)
                n1645 = Build Cluster Array(w3540, w3523) -> (w3541:cluster{dbl, dbl}[])
                n1646 = Build Cluster Array(w3546, w3534) -> (w3542:cluster{dbl, "P(a)":dbl}[])
                n1647 = Build Cluster Array(w3514, w3523) -> (w3539:cluster{dbl, dbl}[])
                n1648 = Build Cluster Array(w3533, w3534) -> (w3538:cluster{dbl, "P(a)":dbl}[])
                n1649 = Array Size(array=w3508) -> (size(s)=w3510:i32)
                n1650 = Build Cluster Array(w3541, w3542) -> (→"V5 Im vs. a^5":cluster{cluster{dbl, "P(a)":dbl}[]}[])
                n1651 = Build Cluster Array(w3539, w3538) -> (→"V5 Im":cluster{cluster{dbl, "P(a)":dbl}[]}[])
                n1652 = Array Size(array=w3505) -> (size(s)=w3511:i32)
                n1653 = Subtract(x=w3510, y=w3507) -> (x-y=w3512:i32)
                n1654 = Increment(x=w3511) -> (x+1=w3509:i32)
                n1655 = Subtract(x=w3509, y=w3510) -> (x-y=w3504:i32)
                n1656 = Index Array(array=w3537, index=0) -> (element=w3549:dbl)
                n1657 = Build Array(w3512, 0, w3504) -> (w3506:i32[])
              }
            }
            n1658 = Build Array(w574, w573, w572, w571, w570, w569, w568, w567, w566, w565, w564, w563, w562, w561, w560) -> (w575:i32[])
            n1659 = Reverse 1D Array(array=w575) -> (reversed array=w556:i32[])
            "Number of Amps used" <- w556
            n1660 = Build Array(w580, w581, w582, w583, w584, w585, w586, w587, w588, w589, w590, w591, w592, w593, w594) -> (w595:i32[][])
            n1661 = Transpose 2D Array(2D array=w595) -> (transposed array=w578:i32[][])
            n1662 = while {
              tunnel: w578 -> [w754]
              tunnel: [w753] -> w579 mode=indexing
              tunnel: [w749] -> _
              tunnel: [w748] -> w554
              i -> [w750]
              stop <- w748 stop-if-true
              w749 = 0
              n1663 = Delete From Array(array=w754, index (row)=w750) -> (deleted portion=w751:i32[])  [unwired: 2 in, 1 out]
              n1664 = Array Size(array=w751) -> (size(s)=w752:i32)
              n1665 = Reverse 1D Array(array=w751) -> (reversed array=w753:i32[])
              n1666 = Equal?(x=w752, y=w749) -> (x = y?=w748:bool)
            }
            "Graphs Updated" <- w554
            n1667 = Delete From Array(array=w579) -> (array with subset deleted=w555:i32[][])  [unwired: 3 in, 1 out]
            "Number of Amps erased" <- w555
            n1668 = event shown="[1] \"Sigma Noise Filter\", \"Error Noise Filter\", \"stop\", \"Fitting Method (vk)\", \"Tolerance (vk)\", \"Gaussian Window Parameter (B)\", \"LS Program\", \"Baseline\", \"Lookup Table\": Value Change" {
              selector: _ -> [_ _]
              dyn-events: _ -> [_ _]
              timeout: _ -> [_ _]
              tunnel: w556 -> [_ _]
              tunnel: w555 -> [_ _]
              tunnel: [w734 TRUE] -> w553
              tunnel: [w734 FALSE] -> w552
              tunnel: [w734 "stop"] -> w495
              event "V13 Fitting", "V24 Fitting", "V15 & V35", "V1 MSE Multiplier", "V2 MSE Multiplier", "V3 MSE Multiplier", "Amps Erase", "V2 Amps Erase", "Alpha Fitting Filters", "V1 Amps Erase", "V3 Amps Erase", "MSE Multiplier", "Tolerance (a)", "Max Iterations (a)", "V1/Alpha Amp to Noise Ratio", "V2 Amp to Noise Ratio", "V3 Amp to Noise Ratio", "V4 Amp to Noise Ratio", "V5 Amp to Noise Ratio", "Weighting", "% of V11", "% of V22/V33": Value Change {
                w734 = FALSE
                n1669 = event-data() -> ()  [unwired: 1 in, 1 out]
              }
              event "Sigma Noise Filter", "Error Noise Filter", "stop", "Fitting Method (vk)", "Tolerance (vk)", "Gaussian Window\nParameter (B)", "LS Program", "Baseline", "Lookup Table": Value Change {
                n1670 = event-data() -> ()  [unwired: 1 in, 3 out]
              }
            }
            n1671 = local write "Graphs Updated"(w552) -> ()
          }
        }
      }
    }
    n1672 = case shown="True" "Write SUBVI Array?" {
      tunnel: w91 -> [_ w3666]
      tunnel: w90 -> [_ w3665]
      frame False {
      }
      frame True {
        n1673 = stacked-sequence {
          seq-local: [w3669 _] -> [_ w3673]
          tunnel: w3666 -> [_ w3676]
          tunnel: w3665 -> [w3667 _]
          frame #0 {
            # "SUBVI Array Labels"
            n1674 = case shown="False" w3667 {
              tunnel: [string[] ["V1 Re", "I1 Re", "I1 Im", "I2 Re", "I2 Im", "I3 Re", "I3 Im", "I4 Re", "I4 Im", "I5 Re", "I5 Im", "I1 Mag", "I2 Mag", "I3 Mag", "I4 Mag", "I5 Mag", "I1 theta", "I2 theta", "I3 theta", "I4 theta", "I5 theta", "", ""] string[] ["I1 Re", "V1 Re", "V1 Im", "V2 Re", "V2 Im", "V3 Re", "V3 Im", "V4 Re", "V4 Im", "V5 Re", "V5 Im", "V1 Mag", "V2 Mag", "V3 Mag", "V4 Mag", "V5 Mag", "V1 theta", "V2 theta", "V3 theta", "V4 theta", "V5 theta", "", ""]] -> w3668
              frame False {
              }
              frame True {
              }
            }
            n1675 = Array To Spreadsheet String(array=w3668, 3:"%s" ("format string")) -> (spreadsheet string=w3669:string)  [unwired: 1 in]
          }
          frame #1 {
            n1676 = Array To Spreadsheet String(array=w3676, 3:"%.8f" ("format (%.3f)")) -> (spreadsheet string=w3675:string)  [unwired: 1 in]
            n1677 = Concatenate Strings(w3673, w3675) -> (w3677:string)
            n1678 = call <vilib>:"Write Characters To File.vi"("append to file? (new file:F)"=TRUE, "character string"=w3677, "file path (dialog if empty)"="File Path Write SUBVI Array") -> ()  [unwired: 2 in, 1 out]
          }
        }
      }
    }
  }
  n1679 = case shown="\"Dimensional\", Default" "Harmonic Nondimensionalization" {
    tunnel: ["Temperature" "Temperature 2"] -> w8
    frame "Dimensional", Default {
    }
    frame "NonDimensional" {
    }
  }
  n1680 = Add(x=w8, y=273.15) -> (x+y=w15:dbl)
  n1681 = Multiply(x=8.314, y=w15) -> (x*y=w11:dbl)
  n1682 = Multiply(x=2, y=96485.34) -> (x*y=w12:dbl)
  n1683 = Divide(x=w11, y=w12) -> (x/y=w1:dbl)
  n1684 = case shown="\"Dimensional\", Default" "Harmonic Nondimensionalization" {
    tunnel: w1 -> [w3682 w3683]
    frame "Dimensional", Default {
      "Vstar" <- w3682
    }
    frame "NonDimensional" {
      "Vstar 2" <- w3683
    }
  }
  n1685 = case shown="\"Dimensional\", Default" "Harmonic Nondimensionalization" {
    tunnel: "Istar Entered" -> [_ w3710]
    tunnel: w51 -> [_ w3709]
    tunnel: [w3684 w3708] -> w50
    tunnel: w49 -> [_ w3707]
    tunnel: w48 -> [_ w3706]
    tunnel: w47 -> [_ w3705]
    tunnel: w46 -> [_ w3704]
    tunnel: w45 -> [_ w3703]
    tunnel: w44 -> [_ w3702]
    tunnel: w43 -> [_ w3701]
    tunnel: w42 -> [_ w3700]
    tunnel: w41 -> [w3685 w3699]
    tunnel: [w3684 w3698] -> w40
    tunnel: [w3684 w3697] -> w39
    tunnel: [w3684 w3696] -> w38
    tunnel: [w3684 w3695] -> w37
    tunnel: [w3684 w3694] -> w36
    tunnel: [w3684 w3693] -> w35
    tunnel: [w3684 w3692] -> w34
    tunnel: [w3684 w3691] -> w33
    tunnel: [w3684 w3690] -> w32
    tunnel: "Rchem" -> [_ w3689]
    tunnel: w1 -> [_ w3688]
    frame "Dimensional", Default {
      n1686 = Array Size(array=w3685) -> (size(s)=w3686:i32)
      n1687 = Initialize Array(nan, w3686) -> (w3684:dbl[])
    }
    frame "NonDimensional" {
      n1688 = case shown="False" w3710 {
        tunnel: w3707 -> [w3752 w3771]
        tunnel: w3688 -> [w3738 w3768]
        tunnel: w3706 -> [w3750 w3770]
        tunnel: w3704 -> [w3746 w3769]
        tunnel: w3703 -> [w3745 w3767]
        tunnel: w3702 -> [w3744 w3766]
        tunnel: w3705 -> [w3749 w3765]
        tunnel: w3701 -> [w3743 w3764]
        tunnel: w3700 -> [w3742 w3763]
        tunnel: w3699 -> [w3741 w3762]
        tunnel: [w3751 w3761] -> w3698
        tunnel: [w3733 w3760] -> w3697
        tunnel: [w3732 w3759] -> w3696
        tunnel: [w3725 w3758] -> w3695
        tunnel: [w3724 w3757] -> w3694
        tunnel: [w3719 w3756] -> w3693
        tunnel: [w3718 w3755] -> w3692
        tunnel: [w3712 w3754] -> w3691
        tunnel: [w3711 w3753] -> w3690
        tunnel: w3689 -> [w3716 _]
        frame False {
          n1689 = Square(x=w3738) -> (x^2=w3747:dbl)
          n1690 = Square(x=w3738) -> (x^2=w3748:dbl)
          n1691 = Power Of X(1:w3738, 2:4) -> (0:w3731:dbl)
          n1692 = Power Of X(1:w3738, 2:3) -> (0:w3730:dbl)
          n1693 = Multiply(x=w3745, y=w3747) -> (x*y=w3726:dbl[])
          n1694 = Multiply(x=w3746, y=w3748) -> (x*y=w3727:dbl[])
          n1695 = Multiply(x=w3749, y=w3738) -> (x*y=w3735:dbl[])
          n1696 = Multiply(x=w3750, y=w3738) -> (x*y=w3736:dbl[])
          n1697 = Multiply(x=w3741, y=w3731) -> (x*y=w3713:dbl[])
          n1698 = Multiply(x=w3742, y=w3731) -> (x*y=w3714:dbl[])
          n1699 = Multiply(x=w3743, y=w3730) -> (x*y=w3720:dbl[])
          n1700 = Multiply(x=w3744, y=w3730) -> (x*y=w3721:dbl[])
          n1701 = Square(x=w3716) -> (x^2=w3737:dbl)
          n1702 = Square(x=w3716) -> (x^2=w3734:dbl)
          n1703 = Power Of X(1:w3716, 2:4) -> (0:w3722:dbl)
          n1704 = Power Of X(1:w3716, 2:3) -> (0:w3728:dbl)
          n1705 = Power Of X(1:w3716, 2:5) -> (0:w3715:dbl)
          n1706 = Divide(x=w3735, y=w3734) -> (x/y=w3732:dbl[])
          n1707 = Divide(x=w3736, y=w3737) -> (x/y=w3733:dbl[])
          n1708 = Divide(x=w3752, y=w3716) -> (x/y=w3751:dbl[])
          n1709 = Divide(x=w3726, y=w3728) -> (x/y=w3724:dbl[])
          n1710 = Divide(x=w3721, y=w3722) -> (x/y=w3719:dbl[])
          n1711 = Divide(x=w3720, y=w3722) -> (x/y=w3718:dbl[])
          n1712 = Divide(x=w3727, y=w3728) -> (x/y=w3725:dbl[])
          n1713 = Divide(x=w3713, y=w3715) -> (x/y=w3711:dbl[])
          n1714 = Divide(x=w3714, y=w3715) -> (x/y=w3712:dbl[])
        }
        frame True {
          n1715 = Divide(x=w3771, y=w3768) -> (x/y=w3761:dbl[])
          n1716 = Divide(x=w3770, y=w3768) -> (x/y=w3760:dbl[])
          n1717 = Divide(x=w3765, y=w3768) -> (x/y=w3759:dbl[])
          n1718 = Divide(x=w3762, y=w3768) -> (x/y=w3753:dbl[])
          n1719 = Divide(x=w3763, y=w3768) -> (x/y=w3754:dbl[])
          n1720 = Divide(x=w3764, y=w3768) -> (x/y=w3755:dbl[])
          n1721 = Divide(x=w3767, y=w3768) -> (x/y=w3757:dbl[])
          n1722 = Divide(x=w3769, y=w3768) -> (x/y=w3758:dbl[])
          n1723 = Divide(x=w3766, y=w3768) -> (x/y=w3756:dbl[])
        }
      }
      n1724 = case shown="False" w3710 {
        tunnel: w3709 -> [w3774 w3783]
        tunnel: [w3773 w3779] -> w3708
        tunnel: w3688 -> [_ w3778]
        tunnel: w3689 -> [w3772 _]
        frame False {
          n1725 = Index Array(array=w3774, index=0) -> (element=w3777:dbl)
          n1726 = Subtract(x=w3774, y=w3777) -> (x-y=w3775:dbl[])
          n1727 = Divide(x=w3775, y=w3772) -> (x/y=w3773:dbl[])
        }
        frame True {
          n1728 = Index Array(array=w3783, index=0) -> (element=w3782:dbl)
          n1729 = Subtract(x=w3783, y=w3782) -> (x-y=w3780:dbl[])
          n1730 = Divide(x=w3780, y=w3778) -> (x/y=w3779:dbl[])
        }
      }
    }
  }
  n1731 = case shown="True" w75 {
    tunnel: [string[] ["Frequency (Hz)", "I11 Mag (Amps)", "I13 Mag", "I22 Mag", "I24 Mag", "I33 Mag", "I35 Mag", "I44 Mag", "I55 Mag", "I11 Real", "I11 Imag", "I13 Real", "I13 Imag", "I22 Real", "I22 Imag", "I24 Real", "I24 Imag", "I33 Real", "I33 Imag", "I44 Real", "I44 Imag", "I55 Real", "I55 Imag (Amps)"] string[] ["Frequency (Hz)", "V11 Mag", "V13 Mag", "V22 Mag", "V24 Mag", "V33 Mag", "V35 Mag", "V44 Mag", "V55 Mag", "V11 Re", "U11 Re", "V11 Im", "U11 Im", "V13 Re", "V13 Im", "V15 Re", "V15 Im", "V22 Re", "U22 Re", "V22 Im", "U22 Im", "V24 Re", "V24 Im", "V33 Re", "U33 Re", "V33 Im", "U33 Im", "V35 Re", "V35 Im", "V44 Re", "U44 Re", "V44 Im", "U44 Im", "V55 Re", "U55 Re", "V55 Im", "U55 Im"]] -> w74
    frame False {
      # "Potentiostatic"
    }
    frame True {
      # "Galvanostatic"
    }
  }
  n1732 = Build Array(w72, w71, w70, w69, w68, w67, w66, w65, w55, w51, w50, w49, w40, w64, w63, w62, w53, w48, w39, w47, w38, w61, w52, w46, w37, w45, w36, w60, w59, w44, w35, w43, w34, w42, w33, w41, w32) -> (w58:dbl[][])
  n1733 = Format Value(format string="%.8f" ("format (%.3f)"), value (0)=w18) -> (output string=w23:string)  [unwired: 1 in]
  n1734 = Format Value(format string="%.8f" ("format (%.3f)"), value (0)="Rchem") -> (output string=w19:string)  [unwired: 1 in]
  n1735 = Format Value(format string="%.8f" ("format (%.3f)"), value (0)=w1) -> (output string=w21:string)  [unwired: 1 in]
  n1736 = Format Value(format string="%.8f" ("format (%.3f)"), value (0)=w8) -> (output string=w6:string)  [unwired: 1 in]
  n1737 = Transpose 2D Array(2D array=w58) -> (transposed array=w57:dbl[][])
  n1738 = Build Array("Istar", w23, "Vstar", w21, "Rchem", w19, "Temp", w6) -> (w17:string[])
  n1739 = case shown="True" "Write NLEIS VIEW to File?" {
    tunnel: w57 -> [_ w3793]
    tunnel: w74 -> [_ w3790]
    tunnel: w17 -> [_ w3787]
    frame False {
    }
    frame True {
      n1740 = Array To Spreadsheet String(array=w3793, 3:"%.8f" ("format (%.3f)")) -> (spreadsheet string=w3795:string)  [unwired: 1 in]
      n1741 = Array To Spreadsheet String(array=w3787, 3:"%s" ("format string")) -> (spreadsheet string=w3786:string)  [unwired: 1 in]
      n1742 = Array To Spreadsheet String(array=w3790, 3:"%s" ("format string")) -> (spreadsheet string=w3794:string)  [unwired: 1 in]
      n1743 = Concatenate Strings(w3786, w3794, w3795) -> (w3792:string)
      n1744 = call <vilib>:"Write Characters To File.vi"("append to file? (new file:F)"="Append To File?", "character string"=w3792, "file path (dialog if empty)"="File Path Write NLEISVIEW Data") -> ()  [unwired: 2 in, 1 out]
    }
  }
